vi "Dust_Control_Giraffe.vi"(7 "error in":errorcluster) -> (0 "error out":errorcluster)   [LabVIEW 2013]
doc: "This VI specifies the properties of the pulse used for running the dust source. When program is stopped, the voltage is incrementally reduced to zero to avoid quick drops."
uses:
  Private/Controls/dust_soruce_control.ctl
  Private/Controls/XYVoltageFGV.ctl
  <vilib>/Utility/miscctls.llb/LVPointTypeDef.ctl
  <vilib>/Utility/error.llb/DialogType.ctl
  <vilib>/Utility/miscctls.llb/LVMinMaxIncTypeDef.ctl
  <vilib>/Utility/miscctls.llb/LVRangeTypeDef.ctl
  <vilib>/DAQmx/read.llb/DAQmx Read (Analog 1D Wfm NChan NSamp).vi
  <vilib>/Analysis/baseanly.llb/Mean (DBL).vi
  <vilib>/DAQmx/write.llb/DAQmx Write (Analog 1D Wfm NChan NSamp).vi
  <vilib>/DAQmx/read.llb/DAQmx Read (Counter U32 1Chan 1Samp).vi
  <vilib>/DAQmx/create/channels.llb/DAQmx Create Channel (AI-Voltage-Basic).vi
  <vilib>/DAQmx/configure/timing.llb/DAQmx Timing (Sample Clock).vi
  <vilib>/DAQmx/create/channels.llb/DAQmx Create Channel (AO-Voltage-Basic).vi
  <vilib>/DAQmx/create/channels.llb/DAQmx Create Channel (CI-Count Edges).vi
  <vilib>/measure/mascope.llb/Amplitude and Levels 1 chan.vi
  <vilib>/DAQmx/miscellaneous.llb/DAQmx Fill In Error Info.vi
  Private/UI Elements/throttle.vi
  <userlib>/_OpenG.lib/comparison/comparison.llb/Boolean Changed__ogtk.vi
  Private/UI Elements/throttle from query.vi
  <userlib>/_OpenG.lib/comparison/comparison.llb/DBL Changed__ogtk.vi
  <vilib>/addons/database/Connection.llb/Conn Execute.vi
  <vilib>/addons/database/Recordset.llb/Rec Fetch Recordset Data (R).vi
  <vilib>/addons/database/Recordset.llb/Rec Destroy - Connection.vi
  Private/Sub-Polymorphic/post_dust_source.vi
  <vilib>/addons/database/_DB Variant To Data/Database Variant To Data.xnode
  <resource>/objmgr/daqmx.rc
  <vilib>/measure/NI_MAPro.lvlib
  <vilib>/Analysis/NI_AALBase.lvlib
  <vilib>/addons/database/NI_Database_API.lvlib
panel:
  out "Einzel and Steering":T1
  out "Y Vs":dbl[](array[numeric])
  out "X Vs":dbl[](array[numeric])
  out "Einzel Vs":dbl[](array[numeric])
  out "Old Einzel":dbl min=0.0 max=10.0 step=0.01 format="%.2g"
  out "Rate Data":dbl[][][](array[numeric])
  out "Freq. Before Throttle":dbl
  out "On/Off":bool
  out "Finished":bool=TRUE
  out "Output waveform":waveform(dbl)={"t0"=timestamp(0 s since 1904-01-01), "dt"=4e-06, "Y"=array[50000 elements]}
  out "Input waveform":waveform(dbl)={"t0"=timestamp(3437998856.0330505 s since 1904-01-01), "dt"=0.00019999999999999998, "Y"=array[1000 elements], "attributes"=variant("NI_ChannelName"=variant(string "Dev5/ai20"), "NI_UnitDescription"=variant(string "Volts"))}
  out "output cluster":T2={"Integer Timestamp"=0, "Einzel Voltage"=0.0, "Needle Voltage"=0.0, "Frequency"=1.0, "Width (ms) : 0.1 "=0.1, "Desired Amplitude (V)"=0.0, "X Voltage"=0.0, "Y Voltage"=0.0, "Settings ID"="", "ID#"=0} {"Needle Voltage" min=0.0 max=10.0 step=0.01 format="%.2g"; "Y Voltage" min=0.0 max=9.0 step=0.01 format="%.2g"; "X Voltage" min=0.0 max=9.0 step=0.01 format="%.2g"; "Einzel Voltage" min=0.0 max=10.0 step=0.01 format="%.2g"; "Desired Amplitude (V)" min=0.0 max=10.0 step=0.01 format="%5.2f"; "Width (ms) : 0.1" min=0.05 max=5.0 step=0.01 format="%6.2f"; "Frequency" min=1.0 max=100.0 step=0.01 format="%.1f"}
  in  "Tab Control":T3(tab)
  in  "Things to Scan":cluster{"Einzel":bool, "X":bool, "Y":bool}={"Einzel"=TRUE, "X"=TRUE, "Y"=TRUE}
  in  "Ein. Range":dbl[](array[numeric])=[0.0, 10.0] min=0.0 max=10.0 step=0.05 format="%#.2g"
  out "Steps to go":i32
  out "Num Steps":i16
  in  "# of Steps":i16[](array[numeric])=[5, 5, 5] min=0 max=10 step=1
  in  "Y Range":dbl[](array[numeric])=[-2.5, 2.5] min=-2.5 max=2.5 step=0.05 format="%#.2g"
  in  "X Range":dbl[](array[numeric])=[-2.5, 2.5] min=-2.5 max=2.5 step=0.05 format="%#.2g"
  in  "Calibrate XY":bool
  out "Actual output width (ms)":dbl caption="Output Width (ms)" format="%.2f"
  out "Actual output Frequency":dbl caption="Output  Freq.(hz)" format="%.2f"
  in  "Width (ms) : 0.1":dbl=0.1 caption="Width (ms)" min=0.0 max=5.0 step=0.01 format="%6.2f"
  out "Actual Amplitude (V) 2":dbl=0.0012999050305587314 caption="Tube Drive" format="%.2f"
  in  "Desired Amplitude (V)":dbl caption="Amplitude (V)" min=0.0 max=10.0 step=0.01 format="%5.2f"
  out "Actual output Amplitude (V)":dbl caption="Output Amp. (V)" format="%.2f"
  in  "Frequency":dbl=1.0 caption="Freq. (Hz)" min=0.0 max=30.0 step=0.01 format="%.1f"
  in  "Abort Change":bool
  out "Actual Needle (kV)":dbl=-1.1093266413053247 caption="Actual Einzel (V)" format="%.2f"
  out "Actual Needle Output (V)":dbl caption="Actual Einzel (V)" format="%.2f"
  in  "Needle Voltage":dbl min=0.0 max=10.0 step=0.01 format="%.2g"
  out "Actual Steerer Y (kV)":dbl=-0.02640654867851852 caption="Actual Einzel (V)" format="%.2f"
  out "Actual Y Output (V)":dbl=4.5 caption="Actual Einzel (V)" format="%.2f"
  in  "Y Voltage":dbl min=-2.5 max=2.5 step=0.01 format="%.2g"
  out "Actual Steerer X (kV)":dbl=-0.07767573560151271 caption="Actual Einzel (V)" format="%.2f"
  out "Actual X Output (V)":dbl=4.5 caption="Actual Einzel (V)" format="%.2f"
  in  "X Voltage":dbl min=-2.5 max=2.5 step=0.01 format="%.2g"
  out "Actual Einzel (kV)":dbl=-1.1709848579608468 caption="Actual Einzel (V)" format="%.2f"
  out "Actual Einzel Output (V)":dbl caption="Actual Einzel (V)" format="%.2f"
  in  "Einzel Voltage":dbl min=0.0 max=10.0 step=0.01 format="%.2g"
  in  "Save Settings?":bool
  in  "Settings ID":string
  out "CONTROLS":waveform(dbl)[](graph)=[{"t0"=timestamp(0 s since 1904-01-01), "dt"=4e-06, "Y"=array[50000 elements]}, {"t0"=timestamp(3437998856.0330505 s since 1904-01-01), "dt"=0.00019999999999999998, "Y"=array[1000 elements], "attributes"=variant("NI_ChannelName"=variant(string "Dev5/ai20"), "NI_UnitDescription"=variant(string "Volts"))}]
  in  "Retrieve Settings":bool
  out "Det2/Det1":dbl
  out "Det3/Det1":dbl
  out "PSU/Det3":dbl
  out "PSU/Det2":dbl
  out "First detector since\nlast source change:":i64
  out "Third detector since\nlast source change:":i64
  out "Source Efficiency":dbl
  out "Det1 Rate":dbl
  out "PSU Rate":dbl
  out "Det3 Rate":dbl
  in  "Cycles to Avg.":i32=10
  out "Hours Run":dbl
  in  "Y Slice":dbl(slide) min=-2.5 max=2.5 step=1.25 scale=-2.5..2.5
  in  "X Slice":dbl(slide) min=-2.5 max=2.5 step=1.25 scale=-2.5..2.5
  in  "Einzel Slice":dbl(slide) min=0.0 max=10.0 step=2.5 scale=0.0..10.0
  out "Y Slice Data":dbl[][](graph)
  out "X Slice Data":dbl[][](graph)
  out "Einzel Slice Data":dbl[][](graph)
  in  "Maximums":cluster{"Width":dbl, "Freq.":dbl}
  out "Testing":bool
  in  "Physical Channels":tag="Dev4/ao19, Dev4/ao9, Dev4/ao11:12, Dev4/ao16" caption="Physical Output Channels"
  in  "Physical Input Channels":tag="Dev5/ai19:23"
  out "Execution Number:":i32=341
  in  "Cal Test?":bool
  in  "Counters On/Off":bool=TRUE
  in  "Reset Counters":bool
  in  "Det1":tag="Dev5/ctr0"
  in  "Det2":tag="Dev5/ctr1"
  in  "Det3":tag="Dev4/ctr0"
  in  "PSU":tag="Dev4/ctr1"
  out "PSU":u32
  out "Det3":u32
  out "Det2":u32
  out "Det1":u32
  out "error?":bool
  out "Actual Sample Clock Rate":dbl=250000.0 format="%.2f"
  in  "stop":bool
  # "Dust Source Control"
  # "Hold Down to\nStop Changes"
  # "E"
  # "x"
  # "y"
  # "Tube Drive (Ao0, Ai4)"
  # "Needle Control (Ao4, Ai0)"
  # "Steerer Y Control (Ao3, Ai3)"
  # "Steerer X Control (Ao2, Ai2)"
  # "Einzel Lens (Ao1, Ai1)"
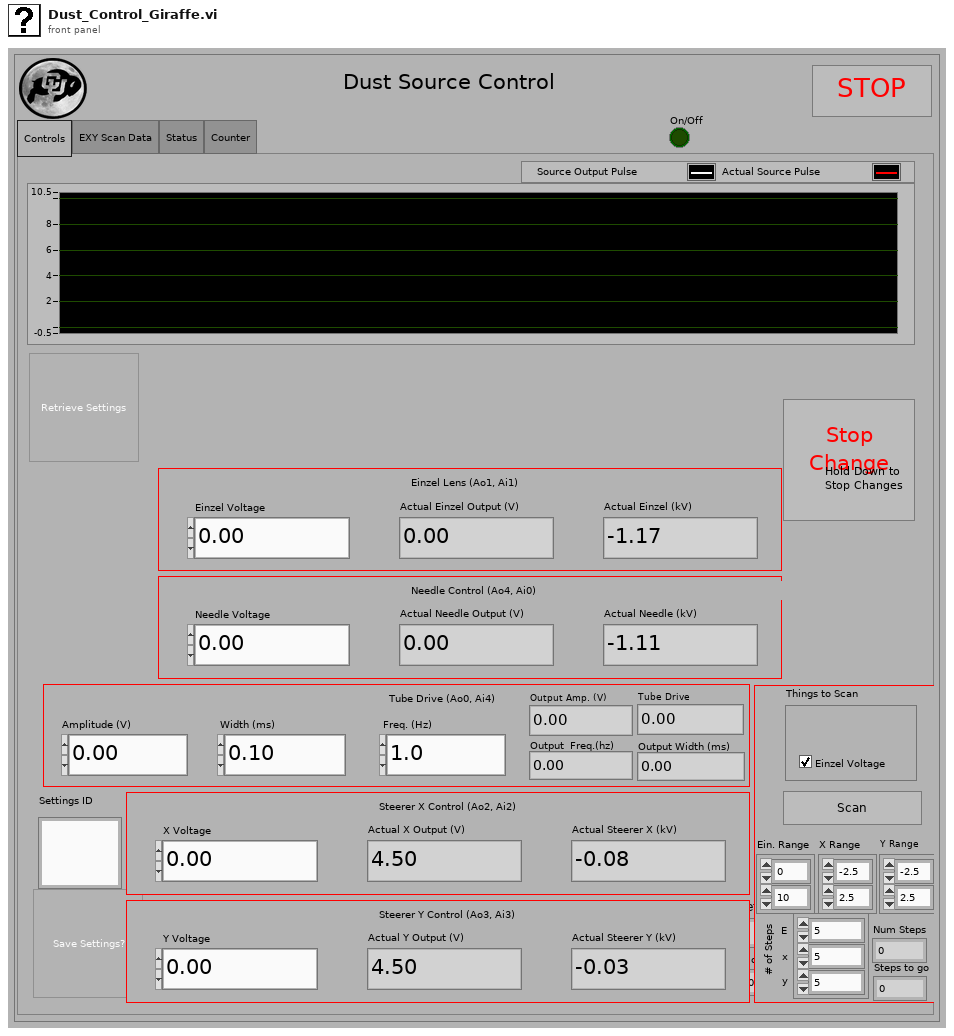
[diagram p1: front panel]
types:
  T1 = cluster{"Einzel Voltage":dbl, "X Voltage":dbl, "Y Voltage":dbl}
  T2 = typedef "dust_soruce_control.ctl" = cluster{"Integer Timestamp":u64, "Einzel Voltage":dbl, "Needle Voltage":dbl, "Frequency":dbl, "Width (ms) : 0.1 ":dbl, "Desired Amplitude (V)":dbl, "X Voltage":dbl, "Y Voltage":dbl, "Settings ID":string, "ID#":i32}
  T3 = enum32{"Controls", "EXY Scan Data", "Status", "Counter"}
  T4 = typedef "LVPointTypeDef.ctl" = cluster{"Horizontal":i16, "Vertical":i16}
  T5 = typedef "XYVoltageFGV.ctl" = u16
  T6 = enum8{"Enabled", "Disabled", "Disabled and Grayed Out"}
  T7 = typedef "DialogType.ctl" = u16
  T8 = typedef "NI_Database_API.lvlib/Conn ObjectReference.ctl" = refnum<k1>
  T9 = typedef "NI_Database_API.lvlib/Rec ObjectReference.ctl" = refnum<k1>
  T10 = typedef "LVRangeTypeDef.ctl" = cluster{"Minimum":dbl, "Maximum":dbl, "Increment":dbl, "Minor Increment":dbl, "Start":dbl}
  T11 = typedef "LVMinMaxIncTypeDef.ctl" = cluster{"Minimum":dbl, "Maximum":dbl, "Increment":dbl}
  T12 = cluster{"data":u32, "data":u32, "data":u32, "data":u32}
  T13 = cluster{"Minimum":dbl, dbl, "Increment":dbl, "Minor Increment":dbl, "Start":dbl}
  T14 = cluster{"Integer Time":i64, "Integer Time":i64, "data":i32}
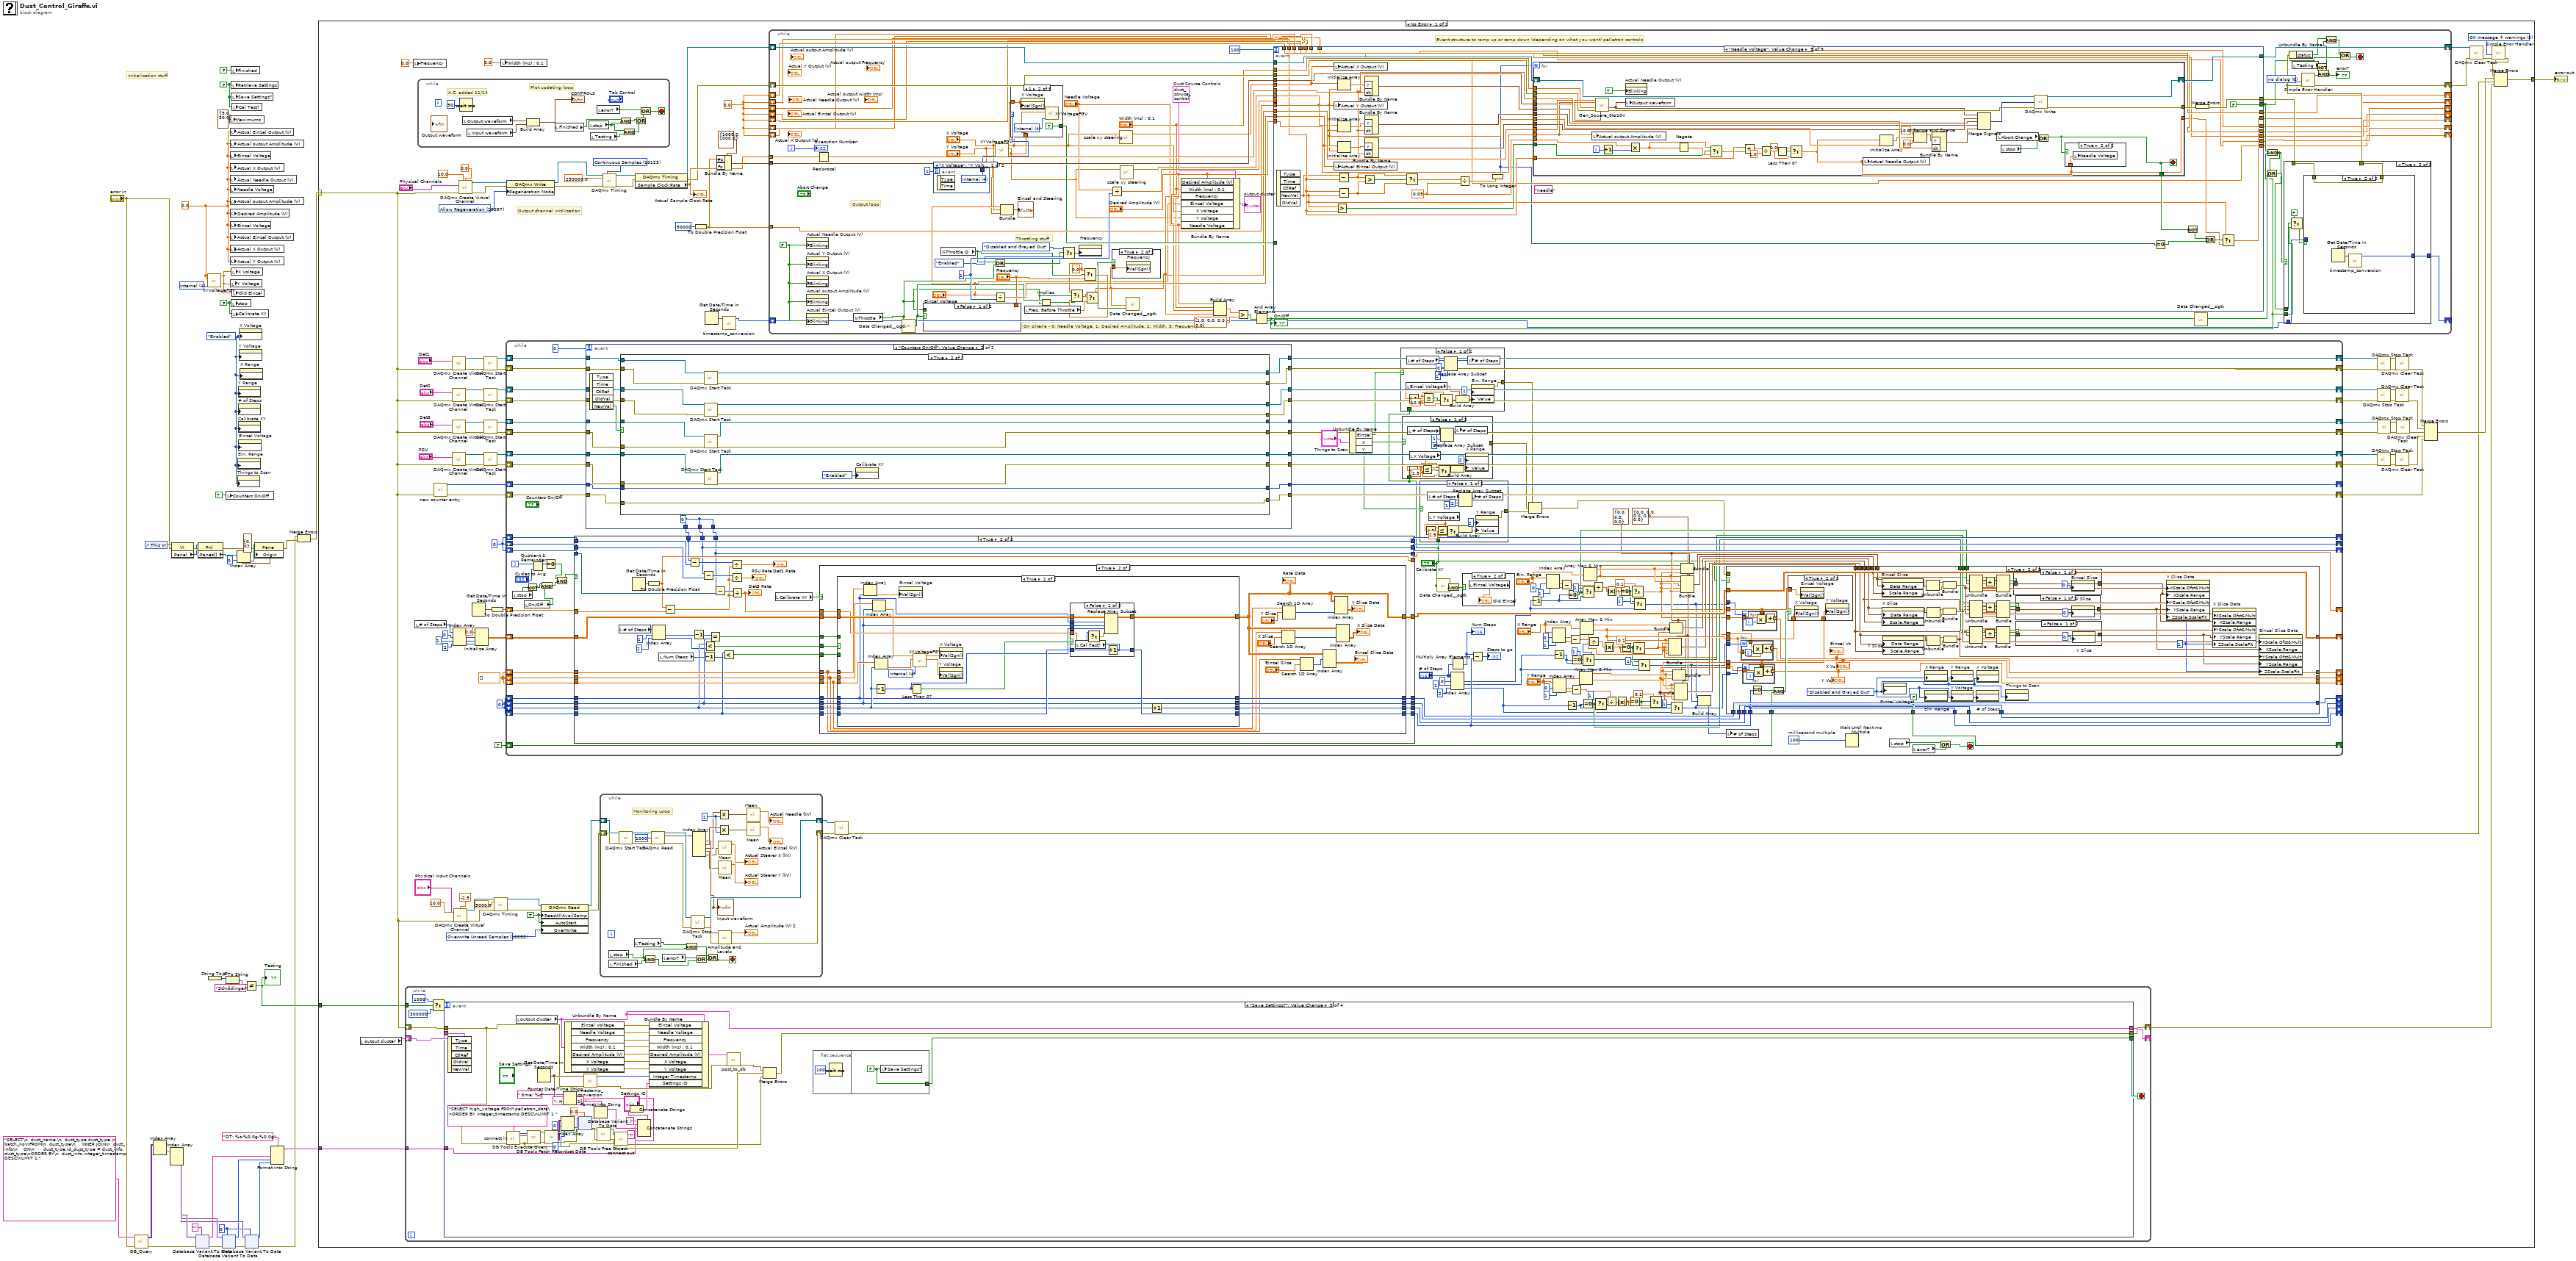
[diagram p0: block diagram]
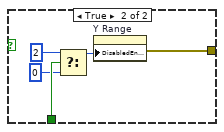
[diagram p2: hidden frame]
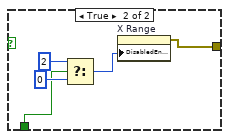
[diagram p3: hidden frame]
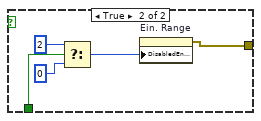
[diagram p4: hidden frame]
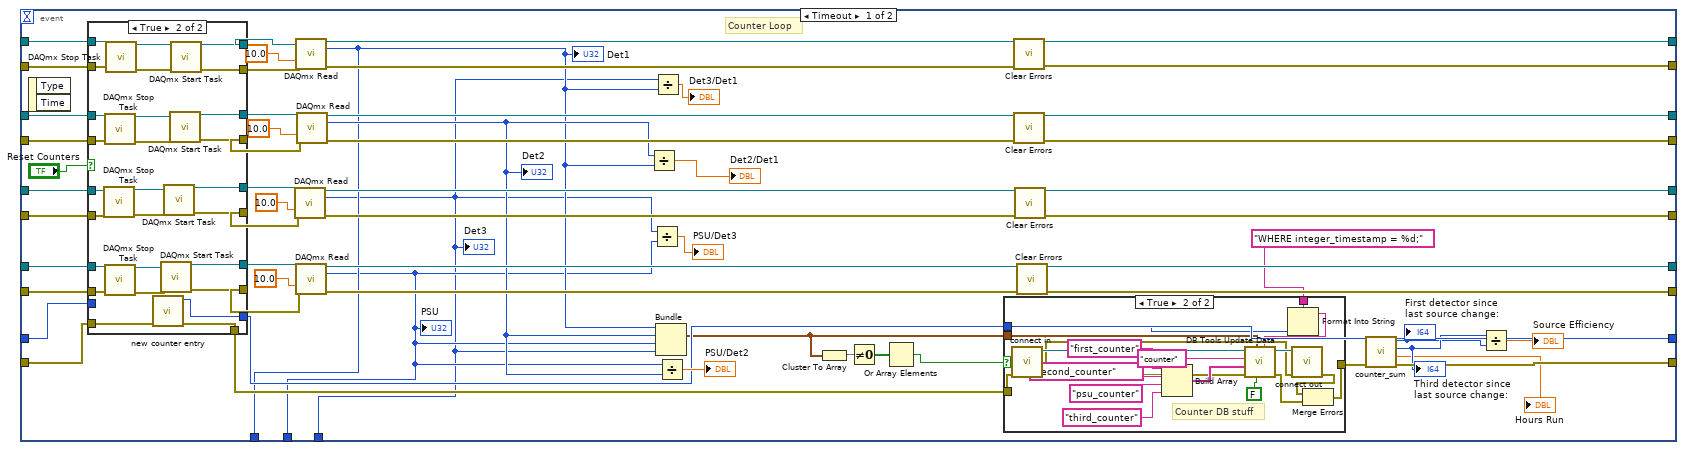
[diagram p6: hidden frame]
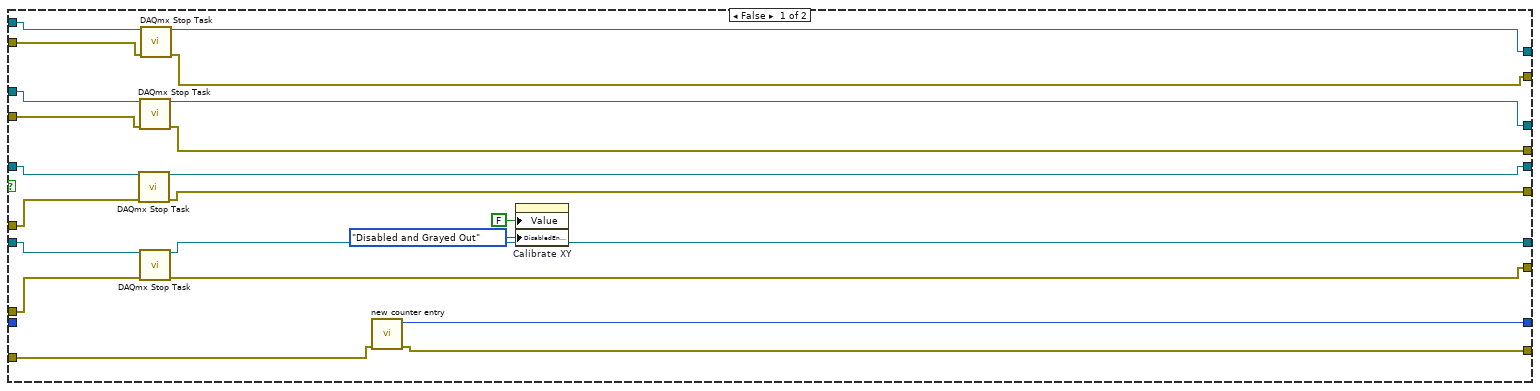
[diagram p9: hidden frame]
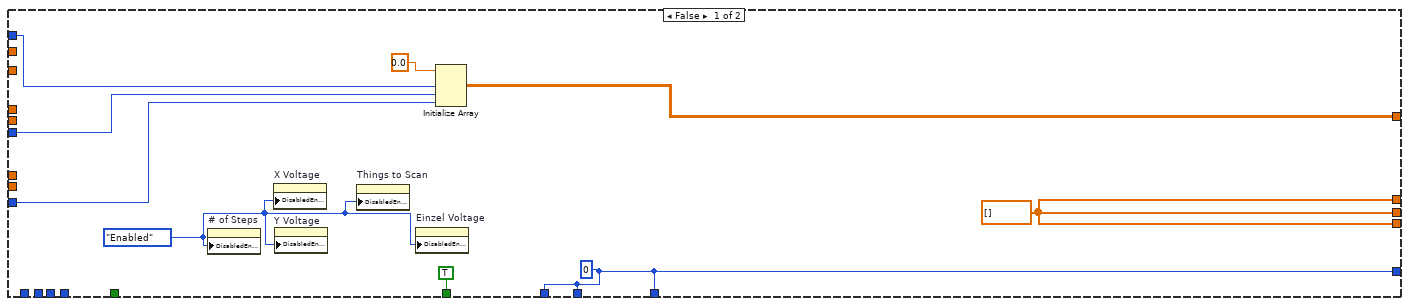
[diagram p10: hidden frame]
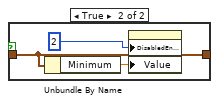
[diagram p11: hidden frame]
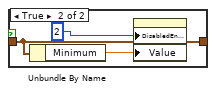
[diagram p12: hidden frame]
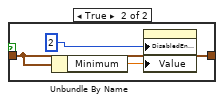
[diagram p13: hidden frame]
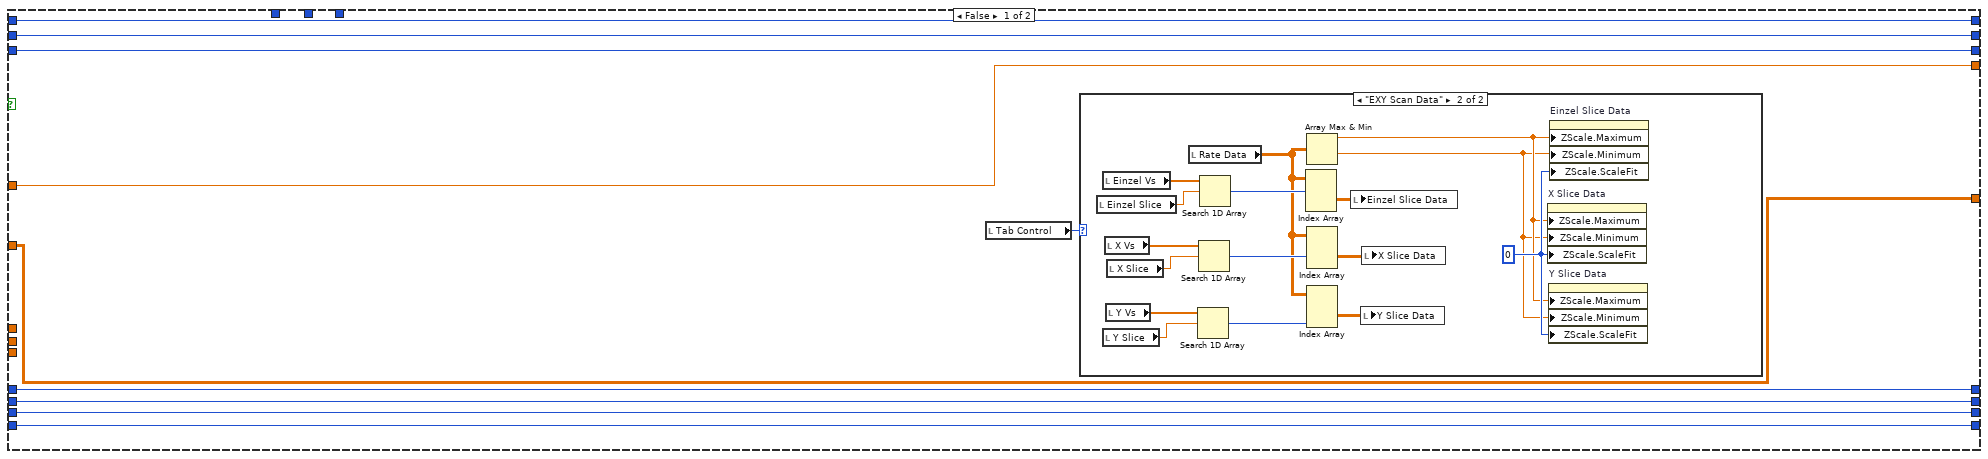
[diagram p15: hidden frame]
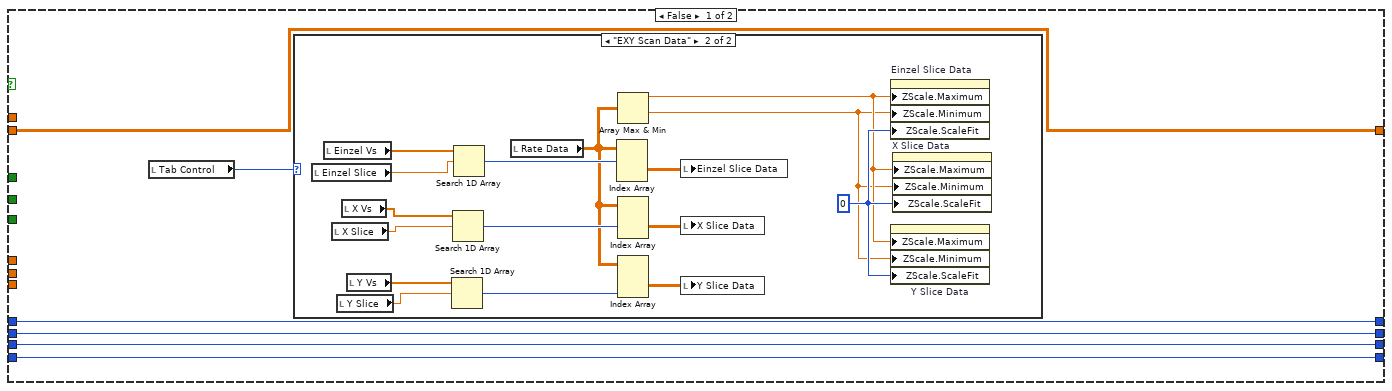
[diagram p17: hidden frame]
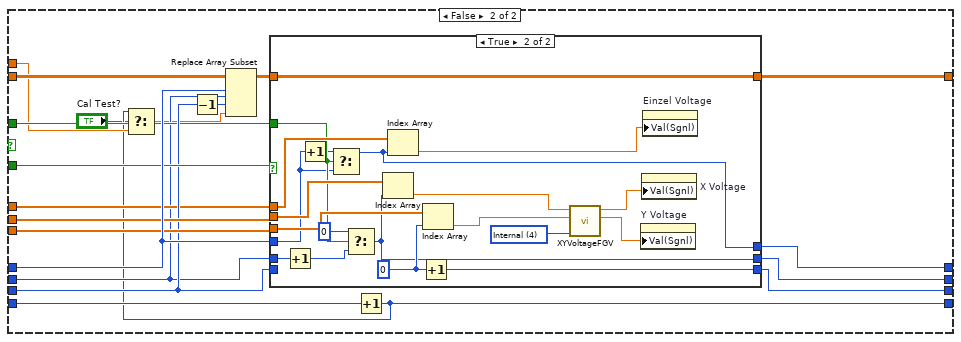
[diagram p20: hidden frame]
diagram:
  w29 = 0
  w38 = T5 4 items=["Get", "Set X", "Set Y", "Set XY", "Internal"] ("Ring")
  w16 = T6."Enabled" ("Disabled")
  w17 = FALSE ("Retrieve Settings")
  w40 = 0.0 ("Actual Output (V)")
  w39 = FALSE ("Shutdown")
  # "Initialization stuff"
  n1 = call "DB_Query.vi"("error in (no error)"="error in", "Parameterized Query"="SELECT\n  dust_name,\n  dust_type.dust_type,\n  batch_no\nFROM\n  dust_type\n    INNER JOIN\n  dust_info\n    ON\n      dust_type.id_dust_type = dust_info.dust_type\nORDER BY\n  dust_info.integer_timestamp DESC\nLIMIT 1;" ("SQL query")) -> ("error out"=w3:errorcluster, "Results"=w2:variant[][])  [unwired: 7 in, 1 out]
  n2 = control-ref of="This VI"() -> (w15:refnum<vi>)
  n3 = Index Array(array=w2) -> (element=w36:variant[])  [unwired: 2 in]
  n4 = Index Array(array=w36) -> (element #1=w35:variant, element #2=w32:variant, element #3=w31:variant)  [unwired: 3 in]
  n5 = property class="VI"(reference=w15, error in="error in") -> (error out=w14:errorcluster, "Panel"=w13:refnum<vi>)  [unwired: 1 out]
  n6 = xnode "Database Variant To Data"("database variant"=w35, "error in (no error)"=w3, "type"="") -> ("data"=w27:string, "error out"=w34:errorcluster)
  n7 = property class="Pnl"(reference=w13, error in=w14) -> (error out=w12:errorcluster, "Panes[]"=w11:refnum<vi>[])  [unwired: 1 out]
  n8 = call "XYVoltageFGV.vi"("X Voltage"=w40, "Y Voltage"=w40, "Ring"=w38) -> ("X Voltage 2"=w18:dbl)  [unwired: 5 in, 2 out]
  n9 = String To IP() -> (0:w23:u32)  [unwired: 1 in]
  n10 = xnode "Database Variant To Data"("database variant"=w32, "error in (no error)"=w34, "type"=w29) -> ("data"=w26:i32, "error out"=w33:errorcluster)
  n11 = local write "Counters On/Off"(TRUE ("Counters On/Off")) -> ()
  n12 = IP To String(2:w23) -> (0:w22:string)  [unwired: 1 in]
  n13 = local write "Maximums"(cluster{"Width":dbl, "Freq.":dbl} {"Width"=5.0, "Freq."=30.0} ("Maximums")) -> ()
  n14 = local write "Actual Einzel Output (V)"(w40) -> ()
  n15 = local write "Actual output Amplitude (V)"(w40) -> ()
  n16 = local write "Einzel Voltage"(w40) -> ()
  n17 = local write "Actual X Output (V)"(w40) -> ()
  n18 = local write "Actual Needle Output (V)"(w40) -> ()
  n19 = local write "Needle Voltage"(w40) -> ()
  n20 = local write "Actual output Amplitude (V)"(w40) -> ()
  n21 = local write "Desired Amplitude (V)"(w40) -> ()
  n22 = local write "Einzel Voltage"(w40) -> ()
  n23 = local write "Actual Einzel Output (V)"(w40) -> ()
  n24 = local write "Actual X Output (V)"(w40) -> ()
  n25 = local write "Actual Y Output (V)"(w40) -> ()
  n26 = local write "Y Voltage"(w18) -> ()
  n27 = local write "Finished"(FALSE ("Finished")) -> ()
  n28 = local write "Retrieve Settings"(w17) -> ()
  n29 = local write "Save Settings?"(w17) -> ()
  n30 = local write "X Voltage"(w18) -> ()
  n31 = local write "stop"(w39) -> ()
  n32 = local write "Cal Test?"(w17) -> ()
  n33 = local write "Old Einzel"(w18) -> ()
  n34 = local write "Calibrate XY"(w39) -> ()
  n35 = Index Array(array=w11, index=0) -> (element=w9:refnum<vi>)
  n36 = property on="Things to Scan" class="Clust (strict)"("DisabledEnum"=w16) -> ()  [unwired: 2 in, 2 out]
  n37 = property on="Ein. Range" class="Arr (strict)"("DisabledEnum"=w16) -> ()  [unwired: 2 in, 2 out]
  n38 = property on="Y Range" class="Arr (strict)"("DisabledEnum"=w16) -> ()  [unwired: 2 in, 2 out]
  n39 = property on="# of Steps" class="Arr (strict)"("DisabledEnum"=w16) -> ()  [unwired: 2 in, 2 out]
  n40 = property on="Calibrate XY" class="Bool (strict)"("DisabledEnum"=w16) -> ()  [unwired: 2 in, 2 out]
  n41 = property on="Einzel Voltage" class="DigNum (strict)"("DisabledEnum"=w16) -> ()  [unwired: 2 in, 2 out]
  n42 = property on="Y Voltage" class="DigNum (strict)"("DisabledEnum"=w16) -> ()  [unwired: 2 in, 2 out]
  n43 = property on="X Voltage" class="DigNum (strict)"("DisabledEnum"=w16) -> ()  [unwired: 2 in, 2 out]
  n44 = property on="X Range" class="Arr (strict)"("DisabledEnum"=w16) -> ()  [unwired: 2 in, 2 out]
  n45 = Not Equal?(x=w22, y="Schrödinger") -> (x != y?=w20:bool)
  "Testing" <- w20
  n46 = xnode "Database Variant To Data"("database variant"=w31, "error in (no error)"=w33, "type"=w29) -> ("data"=w25:i32, "error out"=w1:errorcluster)
  n47 = property class="Pane"(reference=w9, error in=w12, "Origin"=T4 {"Horizontal"=0, "Vertical"=0}) -> (error out=w7:errorcluster)  [unwired: 1 out]
  n48 = Format Into String(format string="DT: %s-%0.0g-%0.0g", w27, w26, w25) -> (resulting string=w24:string)  [unwired: 2 in, 1 out]
  n49 = Merge Errors(w1, w7) -> (w6:errorcluster)
  n50 = case shown="No Error" w6 {
    selector: w6 -> [w64 w2376]
    tunnel: [w43 w2376] -> w42
    tunnel: w24 -> [w50 _]
    tunnel: w20 -> [w49 _]
    frame No Error {
      w53 = 0.0 ("Width (ms) : 3.5")
      w48 = dbl[] []
      w45 = 0
      w74 = 10252 items=["Overwrite Unread Samples"=10252, "Do Not Overwrite Unread Samples"=10159] ("OverWrite")
      w75 = TRUE ("ReadAllAvailSamp")
      w44 = u32 0 ("data")
      w142 = 10097 items=["Allow Regeneration"=10097, "Do Not Allow Regeneration"=10158] ("RegenMode")
      w147 = T7 3 items=["no dialog", "OK message", "continue or stop message", "OK message + warnings", "continue/stop + warnings"] ("type of dialog (OK msg:1)")
      w151 = 10123 items=["Finite Samples"=10178, "Continuous Samples"=10123] ("sample mode")
      # "Output channel initilization"
      n51 = local read "output cluster"() -> (w127:T2)
      n52 = while {
        shift-right: [w907] -> w83
        shift-left: w64 -> [w906]
        shift-right: [w910] -> _
        shift-left: w127 -> [w909]
        tunnel: w50 -> [w904]
        tunnel: w49 -> [w902]
        stop <- w905 stop-if-true
        n53 = Select(t=1000, s=w902, f=300000) -> (s? t:f=w903:i32)
        n54 = event shown="[2] \"Save Settings?\": Value Change" {
          selector: _ -> [_ _ _ _]
          dyn-events: _ -> [_ _ _ _]
          timeout: w903 -> [_ _ _ _]
          tunnel: [w940 w1017 w1061 w1098] -> w910
          tunnel: w909 -> [w939 w1017 _ _]
          tunnel: [w912 w1018 w1028 w1100] -> w907
          tunnel: w906 -> [w913 w1018 w1030 w1099]
          tunnel: [w915 w1014 w1058 _] -> w905
          tunnel: w904 -> [w911 _ w1024 _]
          event Timeout {
            n55 = event-data() -> ()  [unwired: 1 in, 2 out]
            n56 = local read "output cluster"() -> (w940:T2)
            n57 = Unbundle By Name(w940) -> ("Einzel Voltage"=w937:dbl, "Needle Voltage"=w936:dbl, "Frequency"=w934:dbl, "Width (ms) : 0.1"=w932:dbl, "Desired Amplitude (V)"=w930:dbl, "X Voltage"=w929:dbl, "Y Voltage"=w927:dbl)
            n58 = Unbundle By Name(w939) -> ("Einzel Voltage"=w938:dbl, "Needle Voltage"=w935:dbl, "Frequency"=w933:dbl, "Width (ms) : 0.1"=w918:dbl, "Desired Amplitude (V)"=w931:dbl, "X Voltage"=w928:dbl, "Y Voltage"=w926:dbl)
            n59 = Equal?(x=w937, y=w938) -> (x = y?=w925:bool)
            n60 = Equal?(x=w936, y=w935) -> (x = y?=w924:bool)
            n61 = Equal?(x=w934, y=w933) -> (x = y?=w923:bool)
            n62 = Equal?(x=w932, y=w918) -> (x = y?=w922:bool)
            n63 = Equal?(x=w930, y=w931) -> (x = y?=w921:bool)
            n64 = Equal?(x=w929, y=w928) -> (x = y?=w920:bool)
            n65 = Equal?(x=w927, y=w926) -> (x = y?=w919:bool)
            n66 = Compound Arithmetic op=AND(w925, w924, w923, w922, w921, w920, w919) -> (w914:bool)
            n67 = case shown="False" w914 {
              tunnel: w913 -> [w942 w1013]
              tunnel: [w957 w1013] -> w912
              tunnel: w911 -> [w947 _]
              frame False {
                n68 = call "DB_Query.vi"("error in (no error)"=w942, "Parameterized Query"="SELECT\n  high_voltage\nFROM\n  pelletron_data\nORDER BY\n  integer_timestamp DESC\nLIMIT 1; " ("SQL query")) -> ("error out"=w943:errorcluster, "Results"=w944:variant[][])  [unwired: 7 in, 1 out]
                n69 = local read "output cluster"() -> (w959:T2)
                n70 = Get Date/Time In Seconds() -> (seconds since 1Jan1904=w974:timestamp)
                n71 = Format Date/Time String(time format string (%c)="Time: %c)" ("Settings ID"), seconds (now)=w974) -> (date/time string=w949:string)  [unwired: 1 in]
                n72 = Index Array(array=w944, index (row)=0, index (col)=0 ("disabled index (col)")) -> (element=w954:variant)
                n73 = Unbundle By Name(w959) -> ("Einzel Voltage"=w972:dbl, "Needle Voltage"=w971:dbl, "Frequency"=w965:dbl, "Width (ms) : 0.1"=w964:dbl, "Desired Amplitude (V)"=w970:dbl, "X Voltage"=w968:dbl, "Y Voltage"=w967:dbl)
                n74 = xnode "Database Variant To Data"("database variant"=w954, "error in (no error)"=w943, "type"=0.0 ("input 1")) -> ("data"=w952:dbl, "error out"=w941:errorcluster)
                n75 = call "timestamp_conversion.vi"("error in (no error)"=w941, "Time Stamp"=w974) -> ("error out"=w975:errorcluster, "Integer Time"=w976:i64)  [unwired: 7 in]
                n76 = Format Into String(format string="Automatic Update (%s; HV: %0.1f; ", w947, w952) -> (resulting string=w950:string)  [unwired: 2 in, 1 out]
                n77 = Concatenate Strings(w950, w949) -> (w948:string)
                n78 = Bundle By Name(cluster=w959, "Einzel Voltage"=w972, "Needle Voltage"=w971, "Frequency"=w965, "Width (ms) : 0.1"=w964, "Desired Amplitude (V)"=w970, "X Voltage"=w968, "Y Voltage"=w967, "Integer Timestamp"=w976, "Settings ID"=w948) -> (w960:T2)
                n79 = Build Array(w971, w970) -> (w969:dbl[])
                n80 = Less Or Equal?(x=w964, y=0.01) -> (x <= y?=w958:bool)
                n81 = Less?(x=w969, y=0.1) -> (x < y?=w962:bool[])
                n82 = Build Array (concatenate)(w962, w958) -> (w961:bool[])
                n83 = Or Array Elements(Boolean array=w961) -> (logical OR=w946:bool)
                n84 = case shown="False" w946 {
                  tunnel: w960 -> [w1009 _]
                  tunnel: [w1011 w1012] -> w957
                  tunnel: w975 -> [w1010 w1012]
                  frame False {
                    n85 = call-poly "post_to_db.vi"("error in (no error)"=w1010, "Dust control settings"=w1009) -> ("error out"=w1011:errorcluster)  [unwired: 9 in]
                  }
                  frame True {
                  }
                }
              }
              frame True {
              }
            }
            n86 = local read "error?"() -> (w916:bool)
            n87 = local read "stop"() -> (w917:bool)
            n88 = Or(x=w917, y=w916) -> (x .or. y?=w915:bool)
          }
          event "stop": Value Change {
            n89 = event-data() -> ()  [unwired: 1 in, 5 out]
            n90 = local read "stop"() -> (w1016:bool)
            n91 = local read "error?"() -> (w1015:bool)
            n92 = Or(x=w1016, y=w1015) -> (x .or. y?=w1014:bool)
          }
          event "Save Settings?": Value Change {
            n93 = event-data() -> ()  [unwired: 1 in, 5 out]
            n94 = call "connect in.vi"("error in (no error)"=w1030) -> ("error out"=w1043:errorcluster, "Database Connection"=w1046:T8)  [unwired: 6 in, 1 out]
            n95 = local read "output cluster"() -> (w1061:T2)
            n96 = call-poly <vilib>:"DB Tools Execute Query.vi"("error in (no error)"=w1043, "SQL query"="SELECT high_voltage FROM pelletron_data\nORDER BY integer_timestamp DESC\nLIMIT 1 ", "connection reference"=w1046) -> ("error out"=w1045:errorcluster, "recordset reference"=w1044:T9)  [unwired: 5 in]
            n97 = Get Date/Time In Seconds() -> (seconds since 1Jan1904=w1056:timestamp)
            n98 = call-poly <vilib>:"DB Tools Fetch Recordset Data.vi"("error in (no error)"=w1045, "recordset reference"=w1044) -> ("error out"=w1034:errorcluster, "recordset data"=w1038:variant[][], "recordset reference out"=w1042:T9)  [unwired: 3 in]
            n99 = Index Array(array=w1038, index (row)=0, index (col)=0 ("disabled index (col)")) -> (element=w1035:variant)
            n100 = Format Date/Time String(time format string (%c)=" time: %c" ("Settings ID"), seconds (now)=w1056) -> (date/time string=w1022:string)  [unwired: 1 in]
            n101 = Unbundle By Name(w1061) -> ("Einzel Voltage"=w1055:dbl, "Needle Voltage"=w1054:dbl, "Frequency"=w1053:dbl, "Width (ms) : 0.1"=w1052:dbl, "Desired Amplitude (V)"=w1051:dbl, "X Voltage"=w1050:dbl, "Y Voltage"=w1049:dbl)
            n102 = xnode "Database Variant To Data"("database variant"=w1035, "error in (no error)"=w1034, "type"=0.0 ("input 1")) -> ("data"=w1031:dbl, "error out"=w1033:errorcluster)
            n103 = call "timestamp_conversion.vi"("error in (no error)"=w1030, "Time Stamp"=w1056) -> ("error out"=w1059:errorcluster, "Integer Time"=w1060:i64)  [unwired: 7 in]
            n104 = Format Into String(format string="; HV: %0.1f; ", w1031) -> (resulting string=w1023:string)  [unwired: 2 in, 1 out]
            n105 = call-poly <vilib>:"DB Tools Free Object.vi"("error in (no error)"=w1033, "recordset reference"=w1042) -> ("error out"=w1027:errorcluster, "connection reference"=w1041:T8)  [unwired: 8 in]
            n106 = call "connect out.vi"("error in (no error)"=w1043, "connection reference"=w1041) -> ("error out"=w1026:errorcluster)  [unwired: 9 in]
            n107 = Concatenate Strings(" (" ("string"), w1024, w1023, w1022, ")" ("string")) -> (w1020:string)
            n108 = Concatenate Strings("Settings ID", w1020) -> (w1047:string)
            n109 = Bundle By Name(cluster=w1061, "Einzel Voltage"=w1055, "Needle Voltage"=w1054, "Frequency"=w1053, "Width (ms) : 0.1"=w1052, "Desired Amplitude (V)"=w1051, "X Voltage"=w1050, "Y Voltage"=w1049, "Integer Timestamp"=w1060, "Settings ID"=w1047) -> (w1019:T2)
            n110 = call-poly "post_to_db.vi"("error in (no error)"=w1059, "Dust control settings"=w1019) -> ("error out"=w1029:errorcluster)  [unwired: 9 in]
            n111 = Merge Errors(w1029, w1027, w1026) -> (w1028:errorcluster)
            n112 = flat-sequence {
              tunnel: [w1095] -> w1058
              frame #0 {
                n113 = Wait (ms)(milliseconds to wait=u32 100) -> ()  [unwired: 1 out]
              }
              frame #1 {
                w1095 = FALSE
                n114 = local write "Save Settings?"(w1095) -> ()
              }
            }
          }
          event "Retrieve Settings": Value Change {
            n115 = event-data() -> ()  [unwired: 1 in, 5 out]
            n116 = local write "Retrieve Settings"(FALSE) -> ()
            n117 = call "Query_source_settings_menu.vi"("error in (no error)"=w1099) -> ("error out"=w1097:errorcluster, "Cancelled?"=w1096:bool, "Output cluster"=w1098:T2)  [unwired: 8 in]
            n118 = Unbundle By Name(w1098) -> ("Einzel Voltage"=w1108:dbl, "Needle Voltage"=w1107:dbl, "Frequency"=w1106:dbl, "Width (ms) : 0.1"=w1105:dbl, "Desired Amplitude (V)"=w1104:dbl, "X Voltage"=w1103:dbl, "Y Voltage"=w1102:dbl)
            n119 = case shown="False" w1096 {
              tunnel: w1108 -> [w1121 _]
              tunnel: w1097 -> [w1145 w1253]
              tunnel: w1107 -> [w1118 _]
              tunnel: w1106 -> [w1112 _]
              tunnel: w1105 -> [w1115 _]
              tunnel: w1104 -> [w1111 _]
              tunnel: w1103 -> [w1144 _]
              tunnel: w1102 -> [w1128 _]
              tunnel: [w1122 w1253] -> w1100
              frame False {
                n120 = flat-sequence {
                  tunnel: w1145 -> [w1147]
                  tunnel: [w1146] -> w1143
                  tunnel: w1144 -> [w1148]
                  tunnel: [w1148] -> w1142
                  tunnel: w1143 -> [w1150]
                  tunnel: [w1150] -> w1141
                  tunnel: w1142 -> [w1149]
                  tunnel: [w1149] -> w1140
                  tunnel: w1141 -> [w1153]
                  tunnel: [w1152] -> w1139
                  tunnel: w1140 -> [w1154]
                  tunnel: w1139 -> [w1168]
                  tunnel: [w1169] -> w1127
                  tunnel: w1128 -> [w1167]
                  tunnel: [w1167] -> w1123
                  tunnel: w1127 -> [w1172]
                  tunnel: [w1172] -> w1126
                  tunnel: [w1170] -> w1124
                  tunnel: w1123 -> [w1170]
                  tunnel: w1126 -> [w1175]
                  tunnel: [w1174] -> w1125
                  tunnel: w1124 -> [w1173]
                  tunnel: w1125 -> [w1189]
                  tunnel: [w1190] -> w1138
                  tunnel: w1121 -> [w1188]
                  tunnel: [w1188] -> w1120
                  tunnel: w1138 -> [w1192]
                  tunnel: [w1192] -> w1137
                  tunnel: w1120 -> [w1191]
                  tunnel: [w1191] -> w1119
                  tunnel: w1137 -> [w1195]
                  tunnel: [w1196] -> w1136
                  tunnel: w1119 -> [w1194]
                  tunnel: w1136 -> [w1206]
                  tunnel: [w1207] -> w1135
                  tunnel: w1118 -> [w1205]
                  tunnel: [w1205] -> w1116
                  tunnel: [w1209] -> w1134
                  tunnel: w1135 -> [w1209]
                  tunnel: [w1208] -> w1117
                  tunnel: w1116 -> [w1208]
                  tunnel: w1134 -> [w1212]
                  tunnel: [w1213] -> w1133
                  tunnel: w1117 -> [w1211]
                  tunnel: w1133 -> [w1227]
                  tunnel: [w1226] -> w1132
                  tunnel: w1111 -> [w1225]
                  tunnel: [w1225] -> w1109
                  tunnel: w1132 -> [w1230]
                  tunnel: [w1231] -> w1131
                  tunnel: w1115 -> [w1229]
                  tunnel: [w1228] -> w1110
                  tunnel: w1109 -> [w1228]
                  tunnel: w1131 -> [w1234]
                  tunnel: [w1233] -> w1130
                  tunnel: [w1235] -> w1113
                  tunnel: w1112 -> [w1232]
                  tunnel: w1110 -> [w1235]
                  tunnel: w1130 -> [w1237]
                  tunnel: [w1237] -> w1129
                  tunnel: [w1236] -> w1114
                  tunnel: w1113 -> [w1236]
                  tunnel: w1129 -> [w1241]
                  tunnel: [w1240] -> w1122
                  tunnel: w1114 -> [w1239]
                  frame #0 {
                    n121 = property on="X Voltage" class="DigNum (strict)"(error in=w1147, "Val(Sgnl)"=w1148) -> (error out=w1146:errorcluster)  [unwired: 1 in, 1 out]
                  }
                  frame #1 {
                    n122 = Wait (ms)(milliseconds to wait=u32 100) -> ()  [unwired: 1 out]
                  }
                  frame #2 {
                    n123 = while {
                      tunnel: w1154 -> [w1162]
                      shift-right: [w1166] -> w1152
                      shift-left: w1153 -> [w1166]
                      stop <- w1160 stop-if-true
                      n124 = local read "Actual X Output (V)"() -> (w1155:dbl)
                      n125 = local read "stop"() -> (w1157:bool)
                      n126 = local read "Abort Change"() -> (w1158:bool)
                      n127 = call "scale xy steering.vi"("0 to 9 V input"=w1155) -> ("-2.5 to 2.5 V output"=w1156:dbl)  [unwired: 1 in, 1 out]
                      n128 = Subtract(x=w1162, y=w1156) -> (x-y=w1165:dbl)
                      n129 = Absolute Value(x=w1165) -> (abs(x)=w1164:dbl)
                      n130 = Or(x=w1157, y=w1158) -> (x .or. y?=w1159:bool)
                      n131 = Less?(x=w1164, y=0.1) -> (x < y?=w1161:bool)
                      n132 = Or(x=w1161, y=w1159) -> (x .or. y?=w1160:bool)
                    }
                  }
                  frame #3 {
                    n133 = property on="Y Voltage" class="DigNum (strict)"(error in=w1168, "Val(Sgnl)"=w1167) -> (error out=w1169:errorcluster)  [unwired: 1 in, 1 out]
                  }
                  frame #4 {
                    n134 = Wait (ms)(milliseconds to wait=u32 100) -> ()  [unwired: 1 out]
                  }
                  frame #5 {
                    n135 = while {
                      shift-right: [w1187] -> w1174
                      shift-left: w1175 -> [w1187]
                      tunnel: w1173 -> [w1178]
                      stop <- w1181 stop-if-true
                      n136 = local read "Actual Y Output (V)"() -> (w1177:dbl)
                      n137 = local read "Abort Change"() -> (w1180:bool)
                      n138 = local read "stop"() -> (w1179:bool)
                      n139 = call "scale xy steering.vi"("0 to 9 V input"=w1177) -> ("-2.5 to 2.5 V output"=w1176:dbl)  [unwired: 1 in, 1 out]
                      n140 = Subtract(x=w1178, y=w1176) -> (x-y=w1186:dbl)
                      n141 = Absolute Value(x=w1186) -> (abs(x)=w1185:dbl)
                      n142 = Or(x=w1180, y=w1179) -> (x .or. y?=w1182:bool)
                      n143 = Less?(x=w1185, y=0.1) -> (x < y?=w1184:bool)
                      n144 = Or(x=w1184, y=w1182) -> (x .or. y?=w1181:bool)
                    }
                  }
                  frame #6 {
                    n145 = property on="Einzel Voltage" class="DigNum (strict)"(error in=w1189, "Val(Sgnl)"=w1188) -> (error out=w1190:errorcluster)  [unwired: 1 in, 1 out]
                  }
                  frame #7 {
                    n146 = Wait (ms)(milliseconds to wait=u32 100) -> ()  [unwired: 1 out]
                  }
                  frame #8 {
                    n147 = while {
                      shift-right: [w1204] -> w1196
                      shift-left: w1195 -> [w1204]
                      tunnel: w1194 -> [w1197]
                      stop <- w1201 stop-if-true
                      n148 = local read "Actual Einzel Output (V)"() -> (w1202:dbl)
                      n149 = local read "Abort Change"() -> (w1200:bool)
                      n150 = local read "stop"() -> (w1198:bool)
                      n151 = Or(x=w1200, y=w1198) -> (x .or. y?=w1199:bool)
                      n152 = Equal?(x=w1202, y=w1197) -> (x = y?=w1203:bool)
                      n153 = Or(x=w1203, y=w1199) -> (x .or. y?=w1201:bool)
                    }
                  }
                  frame #9 {
                    n154 = property on="Needle Voltage" class="DigNum (strict)"(error in=w1206, "Val(Sgnl)"=w1205) -> (error out=w1207:errorcluster)  [unwired: 1 in, 1 out]
                  }
                  frame #10 {
                    n155 = Wait (ms)(milliseconds to wait=u32 100) -> ()  [unwired: 1 out]
                  }
                  frame #11 {
                    n156 = while {
                      shift-right: [w1224] -> w1213
                      shift-left: w1212 -> [w1224]
                      tunnel: w1211 -> [w1214]
                      stop <- w1218 stop-if-true
                      n157 = local read "Actual Needle Output (V)"() -> (w1220:dbl)
                      n158 = local read "stop"() -> (w1215:bool)
                      n159 = local read "Abort Change"() -> (w1217:bool)
                      n160 = Subtract(x=w1220, y=w1214) -> (x-y=w1223:dbl)
                      n161 = Absolute Value(x=w1223) -> (abs(x)=w1222:dbl)
                      n162 = Or(x=w1215, y=w1217) -> (x .or. y?=w1216:bool)
                      n163 = Less?(x=w1222, y=0.1) -> (x < y?=w1219:bool)
                      n164 = Or(x=w1216, y=w1219) -> (x .or. y?=w1218:bool)
                    }
                  }
                  frame #12 {
                    n165 = property on="Desired Amplitude (V)" class="DigNum (strict)"(error in=w1227, "Val(Sgnl)"=w1225) -> (error out=w1226:errorcluster)  [unwired: 1 in, 1 out]
                  }
                  frame #13 {
                    n166 = property on="Width (ms) : 0.1" class="DigNum (strict)"(error in=w1230, "Val(Sgnl)"=w1229) -> (error out=w1231:errorcluster)  [unwired: 1 in, 1 out]
                  }
                  frame #14 {
                    n167 = property on="Frequency" class="DigNum (strict)"(error in=w1234, "Val(Sgnl)"=w1232) -> (error out=w1233:errorcluster)  [unwired: 1 in, 1 out]
                  }
                  frame #15 {
                    n168 = Wait (ms)(milliseconds to wait=u32 100) -> ()  [unwired: 1 out]
                  }
                  frame #16 {
                    n169 = while {
                      shift-right: [w1251] -> w1240
                      shift-left: w1241 -> [w1251]
                      tunnel: w1239 -> [w1242]
                      stop <- w1246 stop-if-true
                      n170 = local read "Actual output Amplitude (V)"() -> (w1252:dbl)
                      n171 = local read "stop"() -> (w1243:bool)
                      n172 = local read "Abort Change"() -> (w1244:bool)
                      n173 = Subtract(x=w1252, y=w1242) -> (x-y=w1249:dbl)
                      n174 = Absolute Value(x=w1249) -> (abs(x)=w1248:dbl)
                      n175 = Or(x=w1244, y=w1243) -> (x .or. y?=w1245:bool)
                      n176 = Less?(x=w1248, y=0.1) -> (x < y?=w1250:bool)
                      n177 = Or(x=w1250, y=w1245) -> (x .or. y?=w1246:bool)
                    }
                  }
                }
              }
              frame True {
              }
            }
          }
        }
      }
      n178 = local write "Frequency"(0.0 ("Frequency")) -> ()
      n179 = local read "# of Steps"() -> (w59:i16[])
      n180 = while {
        stop <- w867 stop-if-true
        # "Plot updating loop"
        # "A.C. added 11/14"
        n181 = Wait (ms)(milliseconds to wait=u32 50) -> ()  [unwired: 1 out]
        n182 = local read "Output waveform"() -> (w864:waveform(dbl))
        n183 = local read "Input waveform"() -> (w865:waveform(dbl))
        n184 = Build Array(w864, w865) -> (→"CONTROLS":waveform(dbl)[])
        n185 = local read "Finished"() -> (w863:bool)
        n186 = local read "stop"() -> (w858:bool)
        n187 = local read "Testing"() -> (w859:bool)
        n188 = local read "error?"() -> (w866:bool)
        n189 = And(x=w863, y=w858) -> (x .and. y?=w860:bool)
        n190 = And(x=w858, y=w859) -> (x .and. y?=w857:bool)
        n191 = Or(x=w860, y=w857) -> (x .or. y?=w861:bool)
        n192 = Or(x=w866, y=w861) -> (x .or. y?=w867:bool)
      }
      n193 = call "new counter entry.vi"("error in"=w64) -> ("error out"=w81:errorcluster, "Integer Time"=w80:i64)  [unwired: 9 in]
      n194 = call-poly <vilib>:"DAQmx Create Virtual Channel.vi"("counter"="Det1", "error in"=w64) -> ("task out"=w97:refnum<k21>, "error out"=w90:errorcluster)  [unwired: 12 in]
      n195 = call-poly <vilib>:"DAQmx Create Virtual Channel.vi"("counter"="Det2", "error in"=w64) -> ("task out"=w96:refnum<k21>, "error out"=w91:errorcluster)  [unwired: 12 in]
      n196 = call-poly <vilib>:"DAQmx Create Virtual Channel.vi"("counter"="Det3", "error in"=w64) -> ("task out"=w95:refnum<k21>, "error out"=w94:errorcluster)  [unwired: 12 in]
      n197 = call-poly <vilib>:"DAQmx Create Virtual Channel.vi"("counter"="PSU", "error in"=w64) -> ("task out"=w93:refnum<k21>, "error out"=w92:errorcluster)  [unwired: 12 in]
      n198 = Index Array(array=w59, index #1=0 ("index"), index #2=1 ("index"), index #3=2 ("index")) -> (element #1=w56:i16, element #2=w55:i16, element #3=w46:i16)
      n199 = call-poly <vilib>:"DAQmx Create Virtual Channel.vi"("maximum value"=10.0 ("Maximum Value"), "minimum value"=-2.5 ("Minimum Value"), "physical channels"="Physical Input Channels", "error in"=w64) -> ("task out"=w68:refnum<k21>, "error out"=w67:errorcluster)  [unwired: 10 in]
      n200 = call-poly <vilib>:"DAQmx Create Virtual Channel.vi"("maximum value"=10.0 ("Maximum Value"), "minimum value"=0.0 ("Minimum Value"), "physical channels"="Physical Channels", "error in"=w64) -> ("task out"=w141:refnum<k21>, "error out"=w140:errorcluster)  [unwired: 10 in]
      n201 = Get Date/Time In Seconds() -> (seconds since 1Jan1904=w79:timestamp)
      n202 = Initialize Array(0.0 ("element"), w56, w55, w46) -> (w60:dbl[][][])
      n203 = call <vilib>:"DAQmx Start Task.vi"("task/channels in"=w97, "error in"=w90) -> ("task out"=w121:refnum<k21>, "error out"=w114:errorcluster)  [unwired: 12 in]
      n204 = call <vilib>:"DAQmx Start Task.vi"("task/channels in"=w96, "error in"=w91) -> ("task out"=w120:refnum<k21>, "error out"=w115:errorcluster)  [unwired: 12 in]
      n205 = call <vilib>:"DAQmx Start Task.vi"("task/channels in"=w95, "error in"=w94) -> ("task out"=w119:refnum<k21>, "error out"=w116:errorcluster)  [unwired: 12 in]
      n206 = call <vilib>:"DAQmx Start Task.vi"("task/channels in"=w93, "error in"=w92) -> ("task out"=w118:refnum<k21>, "error out"=w117:errorcluster)  [unwired: 12 in]
      n207 = To Double Precision Float(number=w79) -> (double precision float=w78:dbl)
      n208 = call-poly <vilib>:"DAQmx Timing.vi"("task/channels in"=w68, "rate"=5000.0, "error in"=w67) -> ("task out"=w73:refnum<k21>, "error out"=w72:errorcluster)  [unwired: 11 in]
      n209 = local write "Width (ms) : 0.1"(0.0 ("Width (ms) : 3.5")) -> ()
      n210 = while {
        shift-right: [w283] -> _
        shift-left: w80 -> [w285]
        shift-right: [w275] -> _
        shift-left: w78 -> [w270]
        shift-right: [w274] -> _
        shift-left: w44 -> [w281]
        shift-right: [w273] -> _
        shift-left: w44 -> [w280]
        shift-right: [w272] -> _
        shift-left: w44 -> [w279]
        shift-right: [w252] -> _
        shift-left: w48 -> [w248]
        shift-right: [w251] -> _
        shift-left: w48 -> [w247]
        shift-right: [w253] -> _
        shift-left: w60 -> [w254]
        shift-right: [w250] -> _
        shift-left: w45 -> [w246]
        shift-right: [w249] -> _
        shift-left: w45 -> [w245]
        shift-right: [w242] -> _
        shift-left: w45 -> [w241]
        shift-right: [w235] -> _
        shift-left: TRUE -> [w236]
        shift-right: [w305] -> w113
        shift-left: w121 -> [w293]
        shift-right: [w295] -> w112
        shift-left: w114 -> [w292]
        shift-right: [w304] -> w111
        shift-left: w120 -> [w291]
        shift-right: [w301] -> w110
        shift-left: w115 -> [w290]
        shift-right: [w303] -> w109
        shift-left: w119 -> [w289]
        shift-right: [w300] -> w108
        shift-left: w116 -> [w288]
        shift-right: [w302] -> w107
        shift-left: w118 -> [w287]
        shift-right: [w299] -> w106
        shift-left: w117 -> [w286]
        shift-right: [w294] -> w88
        shift-left: w81 -> [w284]
        shift-right: [w213] -> _
        shift-left: w48 -> [w212]
        shift-right: [w208] -> _
        shift-left: w45 -> [w223]
        i -> [w226]
        stop <- w296 stop-if-true
        w183 = T10 {"Minimum"=0.0, "Maximum"=0.0, "Increment"=0.0, "Minor Increment"=0.0, "Start"=0.0} ("Scale.Range")
        w184 = T11 {"Minimum"=0.0, "Maximum"=0.0, "Increment"=0.0} ("Data Entry Limits")
        w298 = u32 100  # millisecond multiple
        n211 = local read "stop"() -> (w269:bool)
        n212 = local read "On/Off"() -> (w225:bool)
        n213 = Not(x=w269) -> (.not. x?=w268:bool)
        n214 = Quotient & Remainder(x=w226, y="Cycles to Avg.") -> (x-y*floor(x/y)=w271:i32)  [unwired: 1 out]
        n215 = And(x=w268, y=w225) -> (x .and. y?=w265:bool)
        n216 = Equal To 0?(x=w271) -> (x = 0?=w266:bool)
        n217 = And(x=w266, y=w265) -> (x .and. y?=w267:bool)
        n218 = event shown="[1] \"Counters On/Off\": Value Change" {
          selector: _ -> [_ _]
          dyn-events: _ -> [_ _]
          timeout: 0 -> [_ _]
          tunnel: [w413 w486] -> w305
          tunnel: [w408 w484] -> w304
          tunnel: [w407 w482] -> w303
          tunnel: [w406 w480] -> w302
          tunnel: [w405 w483] -> w301
          tunnel: [w404 w481] -> w300
          tunnel: [w403 w479] -> w299
          tunnel: [w394 w485] -> w295
          tunnel: [w393 w471] -> w294
          tunnel: w293 -> [w389 w475]
          tunnel: w292 -> [w388 w490]
          tunnel: w291 -> [w387 w476]
          tunnel: w290 -> [w386 w489]
          tunnel: w289 -> [w385 w477]
          tunnel: w288 -> [w384 w488]
          tunnel: w287 -> [w383 w478]
          tunnel: w286 -> [w382 w487]
          tunnel: w285 -> [w372 w474]
          tunnel: w284 -> [w371 w472]
          tunnel: [w369 w473] -> w283
          tunnel: [w365 w470] -> w278
          tunnel: [w364 w470] -> w277
          tunnel: [w363 w470] -> w276
          event Timeout {
            # "Counter Loop"
            n219 = event-data() -> ()  [unwired: 1 in, 2 out]
            n220 = case shown="True" "Reset Counters" {
              tunnel: w389 -> [w442 w469]
              tunnel: [w442 w467] -> w381
              tunnel: w388 -> [w441 w466]
              tunnel: [w441 w464] -> w380
              tunnel: w387 -> [w440 w463]
              tunnel: [w440 w461] -> w379
              tunnel: w386 -> [w439 w460]
              tunnel: [w439 w458] -> w378
              tunnel: w385 -> [w438 w457]
              tunnel: [w438 w455] -> w377
              tunnel: w384 -> [w437 w454]
              tunnel: [w437 w452] -> w376
              tunnel: w383 -> [w436 w451]
              tunnel: [w436 w449] -> w375
              tunnel: w382 -> [w435 w448]
              tunnel: [w435 w446] -> w374
              tunnel: w371 -> [w434 w444]
              tunnel: [w433 w445] -> w369
              tunnel: [w434 w443] -> w370
              tunnel: w372 -> [w433 _]
              frame False {
              }
              frame True {
                n221 = call <vilib>:"DAQmx Stop Task.vi"("task/channels in"=w457, "error in"=w454) -> ("task out"=w456:refnum<k21>, "error out"=w453:errorcluster)  [unwired: 12 in]
                n222 = call <vilib>:"DAQmx Stop Task.vi"("task/channels in"=w463, "error in"=w460) -> ("task out"=w462:refnum<k21>, "error out"=w459:errorcluster)  [unwired: 12 in]
                n223 = call <vilib>:"DAQmx Stop Task.vi"("task/channels in"=w451, "error in"=w448) -> ("task out"=w450:refnum<k21>, "error out"=w447:errorcluster)  [unwired: 12 in]
                n224 = call <vilib>:"DAQmx Stop Task.vi"("task/channels in"=w469, "error in"=w466) -> ("task out"=w468:refnum<k21>, "error out"=w465:errorcluster)  [unwired: 12 in]
                n225 = call "new counter entry.vi"("error in"=w444) -> ("error out"=w443:errorcluster, "Integer Time"=w445:i64)  [unwired: 9 in]
                n226 = call <vilib>:"DAQmx Start Task.vi"("task/channels in"=w450, "error in"=w447) -> ("task out"=w449:refnum<k21>, "error out"=w446:errorcluster)  [unwired: 12 in]
                n227 = call <vilib>:"DAQmx Start Task.vi"("task/channels in"=w456, "error in"=w453) -> ("task out"=w455:refnum<k21>, "error out"=w452:errorcluster)  [unwired: 12 in]
                n228 = call <vilib>:"DAQmx Start Task.vi"("task/channels in"=w462, "error in"=w459) -> ("task out"=w461:refnum<k21>, "error out"=w458:errorcluster)  [unwired: 12 in]
                n229 = call <vilib>:"DAQmx Start Task.vi"("task/channels in"=w468, "error in"=w465) -> ("task out"=w467:refnum<k21>, "error out"=w464:errorcluster)  [unwired: 12 in]
              }
            }
            n230 = call-poly <vilib>:"DAQmx Read.vi"("task/channels in"=w377, "timeout"=10.0, "error in"=w376) -> ("task out"=w407:refnum<k21>, "data"=w363:u32, "error out"=w400:errorcluster)  [unwired: 10 in]
            "Det3" <- w363
            n231 = call-poly <vilib>:"DAQmx Read.vi"("task/channels in"=w381, "timeout"=10.0, "error in"=w380) -> ("task out"=w413:refnum<k21>, "data"=w365:u32, "error out"=w402:errorcluster)  [unwired: 10 in]
            "Det1" <- w365
            n232 = call-poly <vilib>:"DAQmx Read.vi"("task/channels in"=w375, "timeout"=10.0, "error in"=w374) -> ("task out"=w406:refnum<k21>, "data"=w364:u32, "error out"=w399:errorcluster)  [unwired: 10 in]
            "PSU" <- w364
            n233 = call-poly <vilib>:"DAQmx Read.vi"("task/channels in"=w379, "timeout"=10.0, "error in"=w378) -> ("task out"=w408:refnum<k21>, "data"=w390:u32, "error out"=w401:errorcluster)  [unwired: 10 in]
            "Det2" <- w390
            n234 = Divide(x=w390, y=w365) -> (x/y=→"Det2/Det1":dbl)
            n235 = Divide(x=w363, y=w364) -> (x/y=→"PSU/Det3":dbl)
            n236 = Divide(x=w363, y=w365) -> (x/y=→"Det3/Det1":dbl)
            n237 = Bundle("data"=w365, "data"=w390, "data"=w364, "data"=w363) -> (w362:T12)  [unwired: 1 in]
            n238 = Divide(x=w364, y=w390) -> (x/y=→"PSU/Det2":dbl)
            n239 = Cluster To Array(cluster=w362) -> (array=w361:u32[])
            n240 = Not Equal To 0?(x=w361) -> (x != 0?=w360:bool[])
            n241 = Or Array Elements(Boolean array=w360) -> (logical OR=w359:bool)
            n242 = case shown="True" w359 {
              tunnel: [w414 w420] -> w392
              tunnel: "WHERE integer_timestamp = %d;" ("condition") -> [_ w419]
              tunnel: w370 -> [w414 w417]
              tunnel: w369 -> [_ w416]
              tunnel: w362 -> [_ w415]
              frame False {
              }
              frame True {
                # "Counter DB stuff"
                n243 = call "connect in.vi"("error in (no error)"=w417) -> ("error out"=w423:errorcluster, "Database Connection"=w431:T8)  [unwired: 6 in, 1 out]
                n244 = Build Array("first_counter" ("string"), "second_counter" ("string"), "psu_counter" ("string"), "third_counter" ("string")) -> (w427:string[])
                n245 = Format Into String(format string=w419, w416) -> (resulting string=w418:string)  [unwired: 2 in, 1 out]
                n246 = call <vilib>:"DB Tools Update Data.vi"("condition"=w418, "flatten cluster? (F)"=FALSE ("create table? (F)"), "data"=w415, "error in (no error)"=w423, "columns"=w427, "table"="counter", "connection reference"=w431) -> ("error out"=w421:errorcluster, "connection reference out"=w429:T8)  [unwired: 3 in]
                n247 = call "connect out.vi"("error in (no error)"=w423, "connection reference"=w429) -> ("error out"=w422:errorcluster)  [unwired: 9 in]
                n248 = Merge Errors(w422, w421) -> (w420:errorcluster)
              }
            }
            n249 = call <vilib>:"Clear Errors.vi"("error in (no error)"=w402) -> ("error out"=w394:errorcluster)  [unwired: 6 in]
            n250 = call <vilib>:"Clear Errors.vi"("error in (no error)"=w401) -> ("error out"=w405:errorcluster)  [unwired: 6 in]
            n251 = call <vilib>:"Clear Errors.vi"("error in (no error)"=w400) -> ("error out"=w404:errorcluster)  [unwired: 6 in]
            n252 = call <vilib>:"Clear Errors.vi"("error in (no error)"=w399) -> ("error out"=w403:errorcluster)  [unwired: 6 in]
            n253 = call "counter_sum.vi"("error in"=w392) -> ("error IO"=w393:errorcluster, "Number of Hours"=→"Hours Run":dbl, "Third Detector Sum"=w368:i64, "First Detector Sum"=w367:i64)  [unwired: 7 in]
            "First detector since\nlast source change:" <- w367
            "Third detector since\nlast source change:" <- w368
            n254 = Divide(x=w368, y=w367) -> (x/y=→"Source Efficiency":dbl)
          }
          event "Counters On/Off": Value Change {
            w470 = u32 0 ("data")
            n255 = event-data() -> ("NewVal"=w491:bool)  [unwired: 1 in, 4 out]
            n256 = case shown="True" w491 {
              tunnel: w490 -> [w511 w523]
              tunnel: w489 -> [w509 w522]
              tunnel: w488 -> [w507 w521]
              tunnel: w487 -> [w505 w520]
              tunnel: [w497 w531] -> w486
              tunnel: [w498 w530] -> w485
              tunnel: [w499 w529] -> w484
              tunnel: [w500 w528] -> w483
              tunnel: [w501 w527] -> w482
              tunnel: [w502 w526] -> w481
              tunnel: [w504 w525] -> w480
              tunnel: [w503 w524] -> w479
              tunnel: w478 -> [w506 w519]
              tunnel: w477 -> [w508 w518]
              tunnel: w476 -> [w510 w517]
              tunnel: w475 -> [w512 w516]
              tunnel: w474 -> [_ w515]
              tunnel: [w496 w515] -> w473
              tunnel: w472 -> [w495 w514]
              tunnel: [w494 w514] -> w471
              frame False {
                n257 = call <vilib>:"DAQmx Stop Task.vi"("task/channels in"=w508, "error in"=w507) -> ("task out"=w501:refnum<k21>, "error out"=w502:errorcluster)  [unwired: 12 in]
                n258 = call <vilib>:"DAQmx Stop Task.vi"("task/channels in"=w510, "error in"=w509) -> ("task out"=w499:refnum<k21>, "error out"=w500:errorcluster)  [unwired: 12 in]
                n259 = call <vilib>:"DAQmx Stop Task.vi"("task/channels in"=w506, "error in"=w505) -> ("task out"=w504:refnum<k21>, "error out"=w503:errorcluster)  [unwired: 12 in]
                n260 = call <vilib>:"DAQmx Stop Task.vi"("task/channels in"=w512, "error in"=w511) -> ("task out"=w497:refnum<k21>, "error out"=w498:errorcluster)  [unwired: 12 in]
                n261 = call "new counter entry.vi"("error in"=w495) -> ("error out"=w494:errorcluster, "Integer Time"=w496:i64)  [unwired: 9 in]
                n262 = property on="Calibrate XY" class="Bool (strict)"("Value"=FALSE ("Calibrate XY"), "DisabledEnum"=T6."Disabled and Grayed Out" ("Disabled")) -> ()  [unwired: 2 in, 2 out]
              }
              frame True {
                n263 = call <vilib>:"DAQmx Start Task.vi"("task/channels in"=w516, "error in"=w523) -> ("task out"=w531:refnum<k21>, "error out"=w530:errorcluster)  [unwired: 12 in]
                n264 = call <vilib>:"DAQmx Start Task.vi"("task/channels in"=w517, "error in"=w522) -> ("task out"=w529:refnum<k21>, "error out"=w528:errorcluster)  [unwired: 12 in]
                n265 = call <vilib>:"DAQmx Start Task.vi"("task/channels in"=w518, "error in"=w521) -> ("task out"=w527:refnum<k21>, "error out"=w526:errorcluster)  [unwired: 12 in]
                n266 = call <vilib>:"DAQmx Start Task.vi"("task/channels in"=w519, "error in"=w520) -> ("task out"=w525:refnum<k21>, "error out"=w524:errorcluster)  [unwired: 12 in]
                n267 = property on="Calibrate XY" class="Bool (strict)"("DisabledEnum"=T6."Enabled" ("Disabled")) -> ()  [unwired: 2 in, 2 out]
              }
            }
          }
        }
        n268 = case shown="True" w267 {
          tunnel: w270 -> [w648 w704]
          tunnel: w281 -> [w639 w703]
          tunnel: w280 -> [w647 w702]
          tunnel: w279 -> [w646 w701]
          tunnel: w278 -> [_ w695]
          tunnel: w277 -> [_ w694]
          tunnel: w276 -> [_ w693]
          tunnel: [w648 w696] -> w275
          tunnel: [w639 w695] -> w274
          tunnel: [w647 w694] -> w273
          tunnel: [w646 w693] -> w272
          tunnel: w254 -> [w643 w688]
          tunnel: w248 -> [_ w676]
          tunnel: w247 -> [_ w675]
          tunnel: w246 -> [w645 w689]
          tunnel: w245 -> [w644 w670]
          tunnel: [w643 w687] -> w234
          tunnel: [w645 w686] -> w244
          tunnel: [w644 w685] -> w243
          tunnel: w241 -> [w642 w682]
          tunnel: [w642 w683] -> w239
          tunnel: w223 -> [w641 w673]
          tunnel: w212 -> [_ w677]
          tunnel: [w641 w674] -> w207
          frame False {
            n269 = local read "Tab Control"() -> (w640:T3)
            n270 = case shown="\"EXY Scan Data\"" w640 {
              frame "Controls", Default {
              }
              frame "EXY Scan Data" {
                w651 = u8 0 ("Z Scale.Scale Fit")
                n271 = local read "Einzel Slice"() -> (w661:dbl)
                n272 = local read "Einzel Vs"() -> (w664:dbl[])
                n273 = local read "Y Slice"() -> (w659:dbl)
                n274 = local read "X Vs"() -> (w663:dbl[])
                n275 = local read "Y Vs"() -> (w662:dbl[])
                n276 = local read "X Slice"() -> (w660:dbl)
                n277 = local read "Rate Data"() -> (w655:dbl[][][])
                n278 = Search 1D Array(1D array=w662, element=w659) -> (index of element=w658:i32)  [unwired: 1 in]
                n279 = Search 1D Array(1D array=w663, element=w660) -> (index of element=w657:i32)  [unwired: 1 in]
                n280 = Search 1D Array(1D array=w664, element=w661) -> (index of element=w656:i32)  [unwired: 1 in]
                n281 = Index Array(array=w655, index (dim 0)=w656) -> (element=w654:dbl[][])  [unwired: 2 in]
                n282 = Array Max & Min(array=w655) -> (max value=w650:dbl, min value=w649:dbl)  [unwired: 2 out]
                n283 = Index Array(array=w655, index (dim 1)=w657) -> (element=w653:dbl[][])  [unwired: 2 in]
                n284 = Index Array(array=w655, index (dim 2)=w658) -> (element=w652:dbl[][])  [unwired: 2 in]
                n285 = local write "Einzel Slice Data"(w654) -> ()
                n286 = local write "Y Slice Data"(w652) -> ()
                n287 = local write "X Slice Data"(w653) -> ()
                n288 = property on="X Slice Data" class="IntGraph (strict)"("ZScale.Maximum"=w650, "ZScale.Minimum"=w649, "ZScale.ScaleFit"=w651) -> ()  [unwired: 2 in, 2 out]
                n289 = property on="Y Slice Data" class="IntGraph (strict)"("ZScale.Maximum"=w650, "ZScale.Minimum"=w649, "ZScale.ScaleFit"=w651) -> ()  [unwired: 2 in, 2 out]
                n290 = property on="Einzel Slice Data" class="IntGraph (strict)"("ZScale.Maximum"=w650, "ZScale.Minimum"=w649, "ZScale.ScaleFit"=w651) -> ()  [unwired: 2 in, 2 out]
              }
            }
          }
          frame True {
            n291 = local read "# of Steps"() -> (w684:i16[])
            n292 = Get Date/Time In Seconds() -> (seconds since 1Jan1904=w705:timestamp)
            n293 = To Double Precision Float(number=w705) -> (double precision float=w696:dbl)
            n294 = Index Array(array=w684, index #1=1 ("index"), index #2=2 ("index")) -> (element #1=w667:i16, element #2=w666:i16)
            n295 = local read "Num Steps"() -> (w680:i16)
            n296 = Subtract(x=w696, y=w704) -> (x-y=w697:dbl)
            n297 = Subtract(x=w695, y=w703) -> (x-y=w700:u32)
            n298 = Decrement(x=w667) -> (x-1=w665:i16)
            n299 = Subtract(x=w694, y=w702) -> (x-y=w699:u32)
            n300 = Decrement(x=w680) -> (x-1=w679:i16)
            n301 = Less?(x=w673, y=w666) -> (x < y?=w672:bool)
            n302 = Equal?(x=w665, y=w670) -> (x = y?=w671:bool)
            n303 = Subtract(x=w693, y=w701) -> (x-y=w698:u32)
            n304 = Less?(x=w682, y=w679) -> (x < y?=w681:bool)
            n305 = Divide(x=w700, y=w697) -> (x/y=→"Det1 Rate":dbl)
            n306 = Divide(x=w699, y=w697) -> (x/y=→"PSU Rate":dbl)
            n307 = Divide(x=w698, y=w697) -> (x/y=w678:dbl)
            "Det3 Rate" <- w678
            n308 = local read "Calibrate XY"() -> (w690:bool)
            n309 = case shown="True" w690 {
              tunnel: w676 -> [_ w731]
              tunnel: w675 -> [_ w730]
              tunnel: w689 -> [w710 w753]
              tunnel: w670 -> [w709 w752]
              tunnel: w688 -> [w711 w751]
              tunnel: [w711 w742] -> w687
              tunnel: w678 -> [_ w750]
              tunnel: [w710 w749] -> w686
              tunnel: [w709 w748] -> w685
              tunnel: w682 -> [w708 w747]
              tunnel: [w708 w746] -> w683
              tunnel: w681 -> [_ w745]
              tunnel: w673 -> [w707 w744]
              tunnel: w677 -> [_ w738]
              tunnel: [w707 w732] -> w674
              tunnel: w672 -> [_ w729]
              tunnel: w671 -> [_ w728]
              frame False {
                n310 = local read "Tab Control"() -> (w706:T3)
                n311 = case shown="\"EXY Scan Data\"" w706 {
                  frame "Controls", Default {
                  }
                  frame "EXY Scan Data" {
                    w715 = u8 0 ("Z Scale.Scale Fit")
                    n312 = local read "Einzel Slice"() -> (w726:dbl)
                    n313 = local read "Einzel Vs"() -> (w727:dbl[])
                    n314 = local read "X Slice"() -> (w724:dbl)
                    n315 = local read "Y Slice"() -> (w722:dbl)
                    n316 = local read "X Vs"() -> (w725:dbl[])
                    n317 = local read "Y Vs"() -> (w723:dbl[])
                    n318 = Search 1D Array(1D array=w723, element=w722) -> (index of element=w719:i32)  [unwired: 1 in]
                    n319 = Search 1D Array(1D array=w725, element=w724) -> (index of element=w720:i32)  [unwired: 1 in]
                    n320 = Search 1D Array(1D array=w727, element=w726) -> (index of element=w721:i32)  [unwired: 1 in]
                    n321 = local read "Rate Data"() -> (w714:dbl[][][])
                    n322 = Index Array(array=w714, index (dim 0)=w721) -> (element=w718:dbl[][])  [unwired: 2 in]
                    n323 = Array Max & Min(array=w714) -> (max value=w713:dbl, min value=w712:dbl)  [unwired: 2 out]
                    n324 = Index Array(array=w714, index (dim 1)=w720) -> (element=w717:dbl[][])  [unwired: 2 in]
                    n325 = Index Array(array=w714, index (dim 2)=w719) -> (element=w716:dbl[][])  [unwired: 2 in]
                    n326 = local write "Einzel Slice Data"(w718) -> ()
                    n327 = local write "X Slice Data"(w717) -> ()
                    n328 = local write "Y Slice Data"(w716) -> ()
                    n329 = property on="Einzel Slice Data" class="IntGraph (strict)"("ZScale.Maximum"=w713, "ZScale.Minimum"=w712, "ZScale.ScaleFit"=w715) -> ()  [unwired: 2 in, 2 out]
                    n330 = property on="Y Slice Data" class="IntGraph (strict)"("ZScale.Maximum"=w713, "ZScale.Minimum"=w712, "ZScale.ScaleFit"=w715) -> ()  [unwired: 2 in, 2 out]
                    n331 = property on="X Slice Data" class="IntGraph (strict)"("ZScale.Maximum"=w713, "ZScale.Minimum"=w712, "ZScale.ScaleFit"=w715) -> ()  [unwired: 2 in, 2 out]
                  }
                }
              }
              frame True {
                n332 = case shown="True" w729 {
                  tunnel: w753 -> [w756 w805]
                  tunnel: w752 -> [w755 w790]
                  tunnel: w751 -> [w773 w804]
                  tunnel: w750 -> [w772 w788]
                  tunnel: [w756 w803] -> w749
                  tunnel: [w755 w802] -> w748
                  tunnel: w747 -> [w771 w792]
                  tunnel: [w770 w787] -> w746
                  tunnel: w745 -> [_ w801]
                  tunnel: w731 -> [w769 w800]
                  tunnel: w730 -> [w768 w799]
                  tunnel: w744 -> [w759 w798]
                  tunnel: [w767 w797] -> w742
                  tunnel: w738 -> [w766 w796]
                  tunnel: [w758 w795] -> w732
                  tunnel: w728 -> [_ w791]
                  frame True {
                    w761 = T5 4 items=["Get", "Set X", "Set Y", "Set XY", "Internal"] ("Ring")
                    n333 = Index Array(array=w766, index=w756) -> (element=w760:dbl)
                    n334 = Index Array(array=w769, index=w755) -> (element=w764:dbl)
                    n335 = Decrement(x=w759) -> (x-1=w757:i32)
                    n336 = Index Array(array=w768, index=w759) -> (element=w765:dbl)
                    n337 = property on="Einzel Voltage" class="DigNum (strict)"("Val(Sgnl)"=w760) -> ()  [unwired: 2 in, 2 out]
                    n338 = Less Than 0?(x=w757) -> (x < 0?=w754:bool)
                    n339 = call "XYVoltageFGV.vi"("X Voltage"=w764, "Y Voltage"=w765, "Ring"=w761) -> ("X Voltage 2"=w763:dbl, "Y Voltage 2"=w762:dbl)  [unwired: 5 in, 1 out]
                    n340 = property on="Y Voltage" class="DigNum (strict)"("Val(Sgnl)"=w762) -> ()  [unwired: 2 in, 2 out]
                    n341 = property on="X Voltage" class="DigNum (strict)"("Val(Sgnl)"=w763) -> ()  [unwired: 2 in, 2 out]
                    n342 = case shown="False" w754 {
                      tunnel: w773 -> [w783 w785]
                      tunnel: [w782 w785] -> w767
                      tunnel: w757 -> [w779 _]
                      tunnel: w755 -> [w780 _]
                      tunnel: w772 -> [w776 _]
                      tunnel: w771 -> [w778 w784]
                      tunnel: [w775 w784] -> w770
                      tunnel: w756 -> [w781 _]
                      frame False {
                        n343 = local read "Cal Test?"() -> (w774:bool)
                        n344 = Increment(x=w778) -> (x+1=w775:i32)
                        n345 = Select(t=w775, s=w774, f=w776) -> (s? t:f=w777:dbl)
                        n346 = Replace Array Subset(array=w783, new element=w777, index (dim 0)=w781, index (dim 1)=w780, index (dim 2)=w779) -> (w782:dbl[][][])
                      }
                      frame True {
                      }
                    }
                    n347 = Increment(x=w759) -> (x+1=w758:i32)
                  }
                  frame False {
                    n348 = Decrement(x=w798) -> (x-1=w793:i32)
                    n349 = Increment(x=w792) -> (x+1=w787:i32)
                    n350 = Select(t=w787, s="Cal Test?", f=w788) -> (s? t:f=w789:dbl)
                    n351 = Replace Array Subset(array=w804, new element=w789, index (dim 0)=w805, index (dim 1)=w790, index (dim 2)=w793) -> (w794:dbl[][][])
                    n352 = case shown="True" w801 {
                      tunnel: w800 -> [w810 w856]
                      tunnel: w799 -> [w809 w855]
                      tunnel: w805 -> [_ w839]
                      tunnel: w790 -> [_ w847]
                      tunnel: [w807 w844] -> w802
                      tunnel: w794 -> [w808 w849]
                      tunnel: [w808 w849] -> w797
                      tunnel: [w807 w841] -> w803
                      tunnel: w796 -> [w806 w848]
                      tunnel: w798 -> [_ _]
                      tunnel: [w807 w837] -> w795
                      tunnel: w791 -> [_ w840]
                      frame False {
                        w807 = 0
                        n353 = Less Or Equal To 0?(x=w808) -> (x <= 0?=w812:bool[][][])
                        n354 = And Array Elements(Boolean array=w812) -> (logical AND=w811:bool)
                        n355 = case shown="False" w811 {
                          tunnel: w808 -> [w830 _]
                          tunnel: w810 -> [w826 _]
                          tunnel: w809 -> [w825 _]
                          tunnel: w806 -> [w815 _]
                          frame False {
                            w822 = T5 4 items=["Get", "Set X", "Set Y", "Set XY", "Internal"] ("Ring")
                            n356 = Array Max & Min(array=w830) -> (max index (indices)=w829:i32[])  [unwired: 3 out]
                            n357 = Index Array(array=w829, index #1=0 ("index"), index #2=1 ("index"), index #3=2 ("index")) -> (element #1=w816:i32, element #2=w817:i32, element #3=w818:i32)
                            n358 = Index Array(array=w825, index=w818) -> (element=w824:dbl)
                            n359 = Index Array(array=w815, index=w816) -> (element=w814:dbl)
                            n360 = Index Array(array=w826, index=w817) -> (element=w823:dbl)
                            n361 = property on="Einzel Voltage" class="DigNum (strict)"("Val(Sgnl)"=w814) -> ()  [unwired: 2 in, 2 out]
                            n362 = call "XYVoltageFGV.vi"("X Voltage"=w823, "Y Voltage"=w824, "Ring"=w822) -> ("X Voltage 2"=w821:dbl, "Y Voltage 2"=w820:dbl)  [unwired: 5 in, 1 out]
                            n363 = property on="X Voltage" class="DigNum (strict)"("Val(Sgnl)"=w821) -> ()  [unwired: 2 in, 2 out]
                            n364 = property on="Y Voltage" class="DigNum (strict)"("Val(Sgnl)"=w820) -> ()  [unwired: 2 in, 2 out]
                          }
                          frame True {
                            w834 = T5 4 items=["Get", "Set X", "Set Y", "Set XY", "Internal"] ("Ring")
                            n365 = local read "Old Einzel"() -> (w831:dbl)
                            n366 = call "XYVoltageFGV.vi"("X Voltage"=0.0, "Y Voltage"=0.0, "Ring"=w834) -> ("X Voltage 2"=w833:dbl, "Y Voltage 2"=w832:dbl)  [unwired: 5 in, 1 out]
                            n367 = property on="X Voltage" class="DigNum (strict)"("Val(Sgnl)"=w833) -> ()  [unwired: 2 in, 2 out]
                            n368 = property on="Y Voltage" class="DigNum (strict)"("Val(Sgnl)"=w832) -> ()  [unwired: 2 in, 2 out]
                            n369 = property on="Einzel Voltage" class="DigNum (strict)"("Val(Sgnl)"=w831) -> ()  [unwired: 2 in, 2 out]
                          }
                        }
                        n370 = local write "Calibrate XY"(FALSE ("Calibrate XY")) -> ()
                      }
                      frame True {
                        w845 = 0
                        w850 = T5 4 items=["Get", "Set X", "Set Y", "Set XY", "Internal"] ("Ring")
                        n371 = Increment(x=w847) -> (x+1=w843:i32)
                        n372 = Increment(x=w839) -> (x+1=w838:i32)
                        n373 = Select(t=w838, s=w840, f=w839) -> (s? t:f=w841:i32)
                        n374 = Select(t=0, s=w840, f=w843) -> (s? t:f=w844:i32)
                        n375 = Index Array(array=w856, index=w844) -> (element=w853:dbl)
                        n376 = Index Array(array=w848, index=w841) -> (element=w846:dbl)
                        n377 = Increment(x=w845) -> (x+1=w837:i32)
                        n378 = Index Array(array=w855, index=w845) -> (element=w854:dbl)
                        n379 = call "XYVoltageFGV.vi"("X Voltage"=w853, "Y Voltage"=w854, "Ring"=w850) -> ("X Voltage 2"=w851:dbl, "Y Voltage 2"=w852:dbl)  [unwired: 5 in, 1 out]
                        n380 = property on="Y Voltage" class="DigNum (strict)"("Val(Sgnl)"=w852) -> ()  [unwired: 2 in, 2 out]
                        n381 = property on="X Voltage" class="DigNum (strict)"("Val(Sgnl)"=w851) -> ()  [unwired: 2 in, 2 out]
                        n382 = property on="Einzel Voltage" class="DigNum (strict)"("Val(Sgnl)"=w846) -> ()  [unwired: 2 in, 2 out]
                      }
                    }
                  }
                }
                "Rate Data" <- w742
                n383 = Search 1D Array(1D array=w731, element="X Slice") -> (index of element=w733:i32)  [unwired: 1 in]
                n384 = Search 1D Array(1D array=w730, element="Y Slice") -> (index of element=w734:i32)  [unwired: 1 in]
                n385 = Search 1D Array(1D array=w738, element="Einzel Slice") -> (index of element=w737:i32)  [unwired: 1 in]
                n386 = Index Array(array=w742, index (dim 0)=w737) -> (element=→"Einzel Slice Data":dbl[][])  [unwired: 2 in]
                n387 = Index Array(array=w742, index (dim 2)=w734) -> (element=→"Y Slice Data":dbl[][])  [unwired: 2 in]
                n388 = Index Array(array=w742, index (dim 1)=w733) -> (element=→"X Slice Data":dbl[][])  [unwired: 2 in]
              }
            }
          }
        }
        n389 = Unbundle By Name("Things to Scan") -> ("Einzel"=w176:bool, "X"=w175:bool, "Y"=w174:bool)
        n390 = case shown="False" w176 {
          tunnel: [w344 w356] -> w180
          tunnel: "Calibrate XY" -> [_ w353]
          frame False {
            w341 = 10.0 ("y")
            n391 = local read "Einzel Voltage"() -> (w351:dbl)
            n392 = local read "# of Steps"() -> (w348:i16[])
            n393 = Increment(x=w351) -> (x+1=w342:dbl)
            n394 = Less Or Equal?(x=w342, y=w341) -> (x <= y?=w343:bool)
            n395 = Select(t=w342, s=w343, f=w341) -> (s? t:f=w340:dbl)
            n396 = Replace Array Subset(array=w348, new element=i16 1 ("new element/subarray"), index=0) -> (w347:i16[])
            n397 = Build Array(w351, w340) -> (w350:dbl[])
            n398 = local write "# of Steps"(w347) -> ()
            n399 = property on="Ein. Range" class="Arr (strict)"("DisabledEnum"=2 ("element"), "Value"=w350) -> (error out=w344:errorcluster)  [unwired: 2 in, 1 out]
          }
          frame True {
            n400 = Select(t=2, s=w353, f=0 ("element")) -> (s? t:f=w354:i32)
            n401 = property on="Ein. Range" class="Arr (strict)"("DisabledEnum"=w354) -> (error out=w356:errorcluster)  [unwired: 2 in, 1 out]
          }
        }
        n402 = case shown="False" w175 {
          tunnel: [w327 w339] -> w181
          tunnel: "Calibrate XY" -> [_ w336]
          frame False {
            w325 = 2.5 ("y")
            n403 = local read "# of Steps"() -> (w331:i16[])
            n404 = local read "X Voltage"() -> (w334:dbl)
            n405 = Increment(x=w334) -> (x+1=w324:dbl)
            n406 = Less Or Equal?(x=w324, y=w325) -> (x <= y?=w326:bool)
            n407 = Select(t=w324, s=w326, f=w325) -> (s? t:f=w323:dbl)
            n408 = Replace Array Subset(array=w331, new element=i16 1 ("new element/subarray"), index=1) -> (w330:i16[])
            n409 = Build Array(w334, w323) -> (w333:dbl[])
            n410 = local write "# of Steps"(w330) -> ()
            n411 = property on="X Range" class="Arr (strict)"("DisabledEnum"=2 ("element"), "Value"=w333) -> (error out=w327:errorcluster)  [unwired: 2 in, 1 out]
          }
          frame True {
            n412 = Select(t=2, s=w336, f=0 ("element")) -> (s? t:f=w337:i32)
            n413 = property on="X Range" class="Arr (strict)"("DisabledEnum"=w337) -> (error out=w339:errorcluster)  [unwired: 2 in, 1 out]
          }
        }
        n414 = case shown="False" w174 {
          tunnel: [w310 w322] -> w182
          tunnel: "Calibrate XY" -> [_ w320]
          frame False {
            w308 = 2.5 ("y")
            n415 = local read "# of Steps"() -> (w314:i16[])
            n416 = local read "Y Voltage"() -> (w316:dbl)
            n417 = Increment(x=w316) -> (x+1=w307:dbl)
            n418 = Less Or Equal?(x=w307, y=w308) -> (x <= y?=w309:bool)
            n419 = Select(t=w307, s=w309, f=w308) -> (s? t:f=w306:dbl)
            n420 = Replace Array Subset(array=w314, new element=i16 1 ("new element/subarray"), index=2) -> (w313:i16[])
            n421 = Build Array(w316, w306) -> (w317:dbl[])
            n422 = local write "# of Steps"(w313) -> ()
            n423 = property on="Y Range" class="Arr (strict)"("DisabledEnum"=2 ("element"), "Value"=w317) -> (error out=w310:errorcluster)  [unwired: 2 in, 1 out]
          }
          frame True {
            n424 = Select(t=2, s=w320, f=0 ("element")) -> (s? t:f=w321:i32)
            n425 = property on="Y Range" class="Arr (strict)"("DisabledEnum"=w321) -> (error out=w322:errorcluster)  [unwired: 2 in, 1 out]
          }
        }
        n426 = call-poly <userlib>:"Data Changed__ogtk.vi"("Boolean"="Calibrate XY") -> ("Changed"=w196:bool)
        n427 = And(x=w196, y="Calibrate XY") -> (x .and. y?=w197:bool)
        n428 = Index Array(array="# of Steps", index #1=0 ("index"), index #2=1 ("index"), index #3=2 ("index")) -> (element #1=w158:i16, element #2=w160:i16, element #3=w163:i16)
        n429 = Multiply Array Elements(1:"# of Steps") -> (0:w240:i16)
        "Num Steps" <- w240
        n430 = case shown="True" w197 {
          frame False {
          }
          frame True {
            n431 = local read "Einzel Voltage"() -> (→"Old Einzel":dbl)
          }
        }
        n432 = Subtract(x=w240, y=w239) -> (x-y=→"Steps to go":i32)
        n433 = Merge Errors(w180, w181, w182) -> (w179:errorcluster)
        n434 = Decrement(x=w158) -> (x-1=w188:i16)
        n435 = Index Array(array="Ein. Range", index #1=0 ("index"), index #2=1 ("index")) -> (element #1=w220:dbl, element #2=w219:dbl)
        n436 = Index Array(array="X Range", index #1=0 ("index"), index #2=1 ("index")) -> (element #1=w263:dbl, element #2=w264:dbl)
        n437 = Decrement(x=w160) -> (x-1=w229:i16)
        n438 = Index Array(array="Y Range", index #1=0 ("index"), index #2=1 ("index")) -> (element #1=w262:dbl, element #2=w261:dbl)
        n439 = Subtract(x=w220, y=w219) -> (x-y=w218:dbl)
        n440 = Decrement(x=w163) -> (x-1=w231:i16)
        n441 = Equal To 0?(x=w188) -> (x = 0?=w187:bool)
        n442 = Subtract(x=w263, y=w264) -> (x-y=w259:dbl)
        n443 = Subtract(x=w262, y=w261) -> (x-y=w260:dbl)
        n444 = Equal To 0?(x=w229) -> (x = 0?=w186:bool)
        n445 = Array Max & Min(array="Y Range") -> (max value=w203:dbl, min value=w202:dbl)  [unwired: 2 out]
        n446 = Array Max & Min(array="X Range") -> (max value=w201:dbl, min value=w200:dbl)  [unwired: 2 out]
        n447 = Equal To 0?(x=w231) -> (x = 0?=w185:bool)
        n448 = Select(t=i16 1, s=w187, f=w188) -> (s? t:f=w216:i16)
        n449 = Select(t=i16 1, s=w186, f=w229) -> (s? t:f=w227:i16)
        n450 = Array Max & Min(array="Ein. Range") -> (max value=w206:dbl, min value=w205:dbl)  [unwired: 2 out]
        n451 = Divide(x=w259, y=w227) -> (x/y=w258:dbl)
        n452 = Divide(x=w218, y=w216) -> (x/y=w215:dbl)
        n453 = Select(t=i16 1, s=w185, f=w231) -> (s? t:f=w230:i16)
        n454 = Absolute Value(x=w258) -> (abs(x)=w169:dbl)
        n455 = Absolute Value(x=w215) -> (abs(x)=w172:dbl)
        n456 = Divide(x=w260, y=w230) -> (x/y=w257:dbl)
        n457 = Absolute Value(x=w257) -> (abs(x)=w165:dbl)
        n458 = Equal To 0?(x=w172) -> (x = 0?=w157:bool)
        n459 = Equal To 0?(x=w169) -> (x = 0?=w161:bool)
        n460 = Equal To 0?(x=w165) -> (x = 0?=w164:bool)
        n461 = Select(t=0.1, s=w157, f=w172) -> (s? t:f=w171:dbl)
        n462 = Select(t=0.1, s=w161, f=w169) -> (s? t:f=w168:dbl)
        n463 = Select(t=i16 1, s=w157, f=w158) -> (s? t:f=w155:i16)
        n464 = Select(t=i16 1, s=w161, f=w160) -> (s? t:f=w154:i16)
        n465 = Select(t=0.1, s=w164, f=w165) -> (s? t:f=w166:dbl)
        n466 = Bundle(cluster=w183, "Minimum"=w200, "Maximum"=w201, "Increment"=w168, "Minor Increment"=w168, "Start"=w200) -> (w199:T10)
        n467 = Bundle(cluster=w184, "Minimum"=w200, "Maximum"=w201, "Increment"=w168) -> (w211:T11)
        n468 = Select(t=i16 1, s=w164, f=w163) -> (s? t:f=w153:i16)
        n469 = Bundle(cluster=w184, "Minimum"=w202, "Maximum"=w203, "Increment"=w166) -> (w210:T11)
        n470 = Bundle(cluster=w183, "Minimum"=w202, "Maximum"=w203, "Increment"=w166, "Minor Increment"=w166, "Start"=w202) -> (w198:T10)
        n471 = Bundle(cluster=w184, "Minimum"=w205, "Maximum"=w206, "Increment"=w171) -> (w209:T11)
        n472 = Bundle(cluster=w183, "Minimum"=w205, "Maximum"=w206, "Increment"=w171, "Minor Increment"=w171, "Start"=w205) -> (w204:T10)
        n473 = Build Array(w155, w154, w153) -> (w152:i16[])
        n474 = case shown="True" "Calibrate XY" {
          tunnel: w153 -> [w534 w601]
          tunnel: w202 -> [_ w592]
          tunnel: w200 -> [_ w587]
          tunnel: w168 -> [_ w597]
          tunnel: w166 -> [_ w591]
          tunnel: [w536 w589] -> w252
          tunnel: [w536 w590] -> w251
          tunnel: [w538 w605] -> w253
          tunnel: [w537 w604] -> w250
          tunnel: [w537 w603] -> w249
          tunnel: w234 -> [_ w605]
          tunnel: w244 -> [_ w604]
          tunnel: w243 -> [_ w603]
          tunnel: w154 -> [w533 w602]
          tunnel: [w537 w600] -> w242
          tunnel: w239 -> [_ w600]
          tunnel: w236 -> [_ w586]
          tunnel: [TRUE FALSE] -> w235
          tunnel: w205 -> [_ w593]
          tunnel: w171 -> [_ w596]
          tunnel: w155 -> [w535 w595]
          tunnel: [w536 w594] -> w213
          tunnel: w211 -> [_ w583]
          tunnel: w210 -> [_ w582]
          tunnel: w209 -> [_ w584]
          tunnel: w207 -> [_ w588]
          tunnel: [w537 w588] -> w208
          tunnel: w204 -> [_ w559]
          tunnel: w199 -> [_ w551]
          tunnel: w198 -> [_ w543]
          tunnel: w187 -> [_ w568]
          tunnel: w186 -> [_ w567]
          tunnel: w185 -> [_ w566]
          tunnel: w179 -> [_ _]
          frame False {
            w532 = T6."Enabled" ("Disabled")
            w537 = 0
            w536 = dbl[] []
            n475 = property on="# of Steps" class="Arr (strict)"("DisabledEnum"=w532) -> ()  [unwired: 2 in, 2 out]
            n476 = property on="X Voltage" class="DigNum (strict)"("DisabledEnum"=w532) -> ()  [unwired: 2 in, 2 out]
            n477 = property on="Y Voltage" class="DigNum (strict)"("DisabledEnum"=w532) -> ()  [unwired: 2 in, 2 out]
            n478 = property on="Things to Scan" class="Clust (strict)"("DisabledEnum"=w532) -> ()  [unwired: 2 in, 2 out]
            n479 = property on="Einzel Voltage" class="DigNum (strict)"("DisabledEnum"=w532) -> ()  [unwired: 2 in, 2 out]
            n480 = Initialize Array(0.0 ("element"), w535, w533, w534) -> (w538:dbl[][][])
          }
          frame True {
            w569 = u8 1 ("Z Scale.Scale Fit")
            w541 = T6."Disabled and Grayed Out" ("Disabled")
            n481 = for {
              N: w602 -> [_]
              tunnel: w597 -> [w637]
              tunnel: w587 -> [w635]
              tunnel: [w634] -> w589 mode=indexing
              i -> [w638]
              n482 = Multiply(x=w637, y=w638) -> (x*y=w636:dbl)
              n483 = Add(x=w635, y=w636) -> (x+y=w634:dbl)
            }
            "X Vs" <- w589
            n484 = for {
              N: w595 -> [_]
              tunnel: w596 -> [w624]
              tunnel: w593 -> [w623]
              tunnel: [w621] -> w594 mode=indexing
              i -> [w625]
              n485 = Multiply(x=w624, y=w625) -> (x*y=w622:dbl)
              n486 = Add(x=w623, y=w622) -> (x+y=w621:dbl)
            }
            "Einzel Vs" <- w594
            n487 = for {
              N: w601 -> [_]
              tunnel: w591 -> [w632]
              tunnel: w592 -> [w631]
              tunnel: [w629] -> w590 mode=indexing
              i -> [w633]
              n488 = Multiply(x=w632, y=w633) -> (x*y=w630:dbl)
              n489 = Add(x=w631, y=w630) -> (x+y=w629:dbl)
            }
            "Y Vs" <- w590
            n490 = Equal To 0?(x=w600) -> (x = 0?=w585:bool)
            n491 = And(x=w585, y=w586) -> (x .and. y?=w599:bool)
            n492 = case shown="True" w599 {
              tunnel: w587 -> [_ w628]
              tunnel: w592 -> [_ w627]
              tunnel: w593 -> [_ w626]
              frame False {
              }
              frame True {
                n493 = property on="X Voltage" class="DigNum (strict)"("Val(Sgnl)"=w628) -> ()  [unwired: 2 in, 2 out]
                n494 = property on="Einzel Voltage" class="DigNum (strict)"("Val(Sgnl)"=w626) -> ()  [unwired: 2 in, 2 out]
                n495 = property on="Y Voltage" class="DigNum (strict)"("Val(Sgnl)"=w627) -> ()  [unwired: 2 in, 2 out]
              }
            }
            n496 = property on="Einzel Slice" class="Slide (strict)"("Data Range"=w584, "Scale.Range"=w559) -> ()  [unwired: 2 in, 2 out]
            n497 = property on="X Slice" class="Slide (strict)"("Data Range"=w583, "Scale.Range"=w551) -> ()  [unwired: 2 in, 2 out]
            n498 = property on="Y Slice" class="Slide (strict)"("Data Range"=w582, "Scale.Range"=w543) -> ()  [unwired: 2 in, 2 out]
            n499 = property on="Einzel Voltage" class="DigNum (strict)"("DisabledEnum"=w541) -> ()  [unwired: 2 in, 2 out]
            n500 = property on="Ein. Range" class="Arr (strict)"("DisabledEnum"=w541) -> ()  [unwired: 2 in, 2 out]
            n501 = property on="X Range" class="Arr (strict)"("DisabledEnum"=w541) -> ()  [unwired: 2 in, 2 out]
            n502 = Unbundle(w584) -> ("Minimum"=w581:dbl, "Increment"=w580:dbl)  [unwired: 1 out]
            n503 = Unbundle(w582) -> ("Minimum"=w577:dbl, "Increment"=w576:dbl)  [unwired: 1 out]
            n504 = Unbundle(w583) -> ("Minimum"=w579:dbl, "Increment"=w578:dbl)  [unwired: 1 out]
            n505 = Bundle("Minimum"=w581, "Increment"=w580) -> (w575:cluster{"Minimum":dbl, "Increment":dbl})  [unwired: 1 in]
            n506 = Bundle("Minimum"=w579, "Increment"=w578) -> (w574:cluster{"Minimum":dbl, "Increment":dbl})  [unwired: 1 in]
            n507 = Bundle("Minimum"=w577, "Increment"=w576) -> (w573:cluster{"Minimum":dbl, "Increment":dbl})  [unwired: 1 in]
            n508 = property on="Y Range" class="Arr (strict)"("DisabledEnum"=w541) -> ()  [unwired: 2 in, 2 out]
            n509 = property on="Y Voltage" class="DigNum (strict)"("DisabledEnum"=w541) -> ()  [unwired: 2 in, 2 out]
            n510 = Unbundle(w543) -> ("Minimum"=w549:dbl, "Maximum"=w548:dbl, "Increment"=w546:dbl, "Minor Increment"=w545:dbl, "Start"=w544:dbl)
            n511 = Unbundle(w559) -> ("Minimum"=w565:dbl, "Maximum"=w564:dbl, "Increment"=w562:dbl, "Minor Increment"=w561:dbl, "Start"=w560:dbl)
            n512 = Unbundle(w551) -> ("Minimum"=w557:dbl, "Maximum"=w556:dbl, "Increment"=w554:dbl, "Minor Increment"=w553:dbl, "Start"=w552:dbl)
            n513 = property on="# of Steps" class="Arr (strict)"("DisabledEnum"=w541) -> ()  [unwired: 2 in, 2 out]
            n514 = property on="X Voltage" class="DigNum (strict)"("DisabledEnum"=w541) -> ()  [unwired: 2 in, 2 out]
            n515 = Add(x=w548, y=w546) -> (x+y=w547:dbl)
            n516 = Add(x=w564, y=w562) -> (x+y=w563:dbl)
            n517 = Add(x=w556, y=w554) -> (x+y=w555:dbl)
            n518 = Bundle("Minimum"=w549, w547, "Increment"=w546, "Minor Increment"=w545, "Start"=w544) -> (w542:T13)  [unwired: 1 in]
            n519 = Bundle("Minimum"=w565, w563, "Increment"=w562, "Minor Increment"=w561, "Start"=w560) -> (w558:T13)  [unwired: 1 in]
            n520 = Bundle("Minimum"=w557, w555, "Increment"=w554, "Minor Increment"=w553, "Start"=w552) -> (w550:T13)  [unwired: 1 in]
            n521 = property on="Things to Scan" class="Clust (strict)"("DisabledEnum"=w541) -> ()  [unwired: 2 in, 2 out]
            n522 = case shown="False" w568 {
              tunnel: w558 -> [w616 w618]
              tunnel: [w616 w618] -> w572
              frame False {
                n523 = property on="Einzel Slice" class="Slide (strict)"("DisabledEnum"=0) -> ()  [unwired: 2 in, 2 out]
              }
              frame True {
                n524 = Unbundle By Name(w618) -> ("Minimum"=w619:dbl)
                n525 = property on="Einzel Slice" class="Slide (strict)"("DisabledEnum"=2, "Value"=w619) -> ()  [unwired: 2 in, 2 out]
              }
            }
            n526 = case shown="False" w567 {
              tunnel: w550 -> [w611 w614]
              tunnel: [w611 w614] -> w571
              frame False {
                n527 = property on="X Slice" class="Slide (strict)"("DisabledEnum"=0) -> ()  [unwired: 2 in, 2 out]
              }
              frame True {
                n528 = Unbundle By Name(w614) -> ("Minimum"=w613:dbl)
                n529 = property on="X Slice" class="Slide (strict)"("DisabledEnum"=2, "Value"=w613) -> ()  [unwired: 2 in, 2 out]
              }
            }
            n530 = case shown="False" w566 {
              tunnel: w542 -> [w606 w609]
              tunnel: [w606 w609] -> w570
              frame False {
                n531 = property on="Y Slice" class="Slide (strict)"("DisabledEnum"=0) -> ()  [unwired: 2 in, 2 out]
              }
              frame True {
                n532 = Unbundle By Name(w609) -> ("Minimum"=w608:dbl)
                n533 = property on="Y Slice" class="Slide (strict)"("DisabledEnum"=2, "Value"=w608) -> ()  [unwired: 2 in, 2 out]
              }
            }
            n534 = property on="Y Slice Data" class="IntGraph (strict)"("XScale.Ofst&Mult"=w575, "XScale.Range"=w572, "YScale.Ofst&Mult"=w574, "YScale.Range"=w571, "ZScale.ScaleFit"=w569) -> ()  [unwired: 2 in, 2 out]
            n535 = property on="X Slice Data" class="IntGraph (strict)"("XScale.Ofst&Mult"=w575, "XScale.Range"=w572, "YScale.Ofst&Mult"=w573, "YScale.Range"=w570, "ZScale.ScaleFit"=w569) -> ()  [unwired: 2 in, 2 out]
            n536 = property on="Einzel Slice Data" class="IntGraph (strict)"("XScale.Ofst&Mult"=w574, "XScale.Range"=w571, "YScale.Ofst&Mult"=w573, "YScale.Range"=w570, "ZScale.ScaleFit"=w569) -> ()  [unwired: 2 in, 2 out]
          }
        }
        n537 = local write "# of Steps"(w152) -> ()
        n538 = Wait Until Next ms Multiple(millisecond multiple=w298) -> ()  [unwired: 1 out]
        n539 = local read "stop"() -> (w232:bool)
        n540 = local read "error?"() -> (w297:bool)
        n541 = Or(x=w232, y=w297) -> (x .or. y?=w296:bool)
      }
      n542 = property class="DAQmx Write"(reference=w141, error in=w140, "Regeneration Mode"=w142) -> (reference out=w138:refnum<k21>, error out=w137:errorcluster)
      n543 = property class="DAQmx Read"(reference=w73, error in=w72, "ReadAllAvailSamp"=w75, "AutoStart"=w75, "OverWrite"=w74) -> (reference out=w65:refnum<k21>, error out=w63:errorcluster)
      n544 = while {
        shift-right: [w879] -> w62
        shift-left: w65 -> [w880]
        shift-right: [w881] -> w77
        shift-left: w63 -> [w877]
        stop <- w878 stop-if-true
        w885 = 2
        # "Monitoring Loop"
        n545 = local read "stop"() -> (w874:bool)
        n546 = local read "Finished"() -> (w900:bool)
        n547 = call <vilib>:"DAQmx Start Task.vi"("task/channels in"=w880, "error in"=w877) -> ("task out"=w886:refnum<k21>, "error out"=w887:errorcluster)  [unwired: 12 in]
        n548 = local read "Testing"() -> (w876:bool)
        n549 = And(x=w874, y=w900) -> (x .and. y?=w899:bool)
        n550 = call-poly <vilib>:"DAQmx Read.vi"("task/channels in"=w886, "number of samples per channel"=1000, "error in"=w887) -> ("task out"=w888:refnum<k21>, "data"=w883:waveform(dbl)[], "error out"=w889:errorcluster)  [unwired: 10 in]
        n551 = local read "error?"() -> (w884:bool)
        n552 = And(x=w876, y=w874) -> (x .and. y?=w875:bool)
        n553 = call <vilib>:"DAQmx Stop Task.vi"("task/channels in"=w888, "error in"=w889) -> ("task out"=w879:refnum<k21>, "error out"=w898:errorcluster)  [unwired: 12 in]
        n554 = Index Array(array=w883) -> (element #1=w873:waveform(dbl), element #2=w872:waveform(dbl), element #3=w871:waveform(dbl), element #4=w870:waveform(dbl), element #5=w869:waveform(dbl))  [unwired: 5 in]
        "Input waveform" <- w873
        n555 = Or(x=w884, y=w899) -> (x .or. y?=w882:bool)
        n556 = Or(x=w875, y=w882) -> (x .or. y?=w878:bool)
        n557 = Multiply(x=w871, y=w885) -> (x*y=w894:waveform(dbl))
        n558 = Multiply(x=w872, y=w885) -> (x*y=w892:waveform(dbl))
        n559 = call-poly <vilib>:"Mean.vi"("X"=w869) -> ("mean"=→"Actual Steerer X (kV)":dbl)  [unwired: 1 out]
        n560 = call-poly <vilib>:"Mean.vi"("X"=w870) -> ("mean"=→"Actual Steerer Y (kV)":dbl)  [unwired: 1 out]
        n561 = call-poly <vilib>:"Amplitude and Levels.vi"("error in (no error)"=w898, "signal in"=w873) -> ("error out"=w881:errorcluster, "amplitude"=→"Actual Amplitude (V) 2":dbl)  [unwired: 6 in, 2 out]
        n562 = call-poly <vilib>:"Mean.vi"("X"=w894) -> ("mean"=→"Actual Needle (kV)":dbl)  [unwired: 1 out]
        n563 = call-poly <vilib>:"Mean.vi"("X"=w892) -> ("mean"=→"Actual Einzel (kV)":dbl)  [unwired: 1 out]
      }
      n564 = call-poly <vilib>:"DAQmx Timing.vi"("task/channels in"=w138, "sample mode"=w151, "rate"=250000.0 ("Sample Clock Rate"), "error in"=w137) -> ("task out"=w145:refnum<k21>, "error out"=w126:errorcluster)  [unwired: 10 in]
      n565 = property class="DAQmx Timing"(reference=w145, error in=w126) -> (reference out=w129:refnum<k21>, error out=w89:errorcluster, "Sample Clock:Rate"=w134:dbl)
      "Actual Sample Clock Rate" <- w134
      n566 = To Double Precision Float(number=u32 50000 ("Size (Samples)")) -> (double precision float=w133:dbl)
      n567 = Get Date/Time In Seconds() -> (seconds since 1Jan1904=w52:timestamp)
      n568 = Bundle By Name(cluster=cluster{"Fs":dbl, "#s":dbl} {"Fs"=1000.0, "#s"=1000.0} ("sampling info"), "#s"=w133, "Fs"=w134) -> (w143:cluster{"Fs":dbl, "#s":dbl})
      n569 = call "timestamp_conversion.vi"("Time Stamp"=w52) -> ("Integer Time"=w51:i64)  [unwired: 8 in, 1 out]
      n570 = while {
        tunnel: w143 -> [w1331]
        tunnel: w134 -> [w1329]
        tunnel: w133 -> [w1316]
        shift-right: [w1328] -> w132
        shift-left: w129 -> [w1326]
        shift-right: [w1324] -> w128
        shift-left: w89 -> [w1333]
        shift-right: [w1278] -> _
        shift-left: w53 -> [w1285]
        shift-right: [w1277] -> _
        shift-left: w53 -> [w1284]
        shift-right: [w1276] -> _
        shift-left: w53 -> [w1283]
        shift-right: [w1275] -> _
        shift-left: w53 -> [w1282]
        shift-right: [w1274] -> _
        shift-left: w53 -> [w1281]
        shift-right: [w1273] -> _
        shift-left: w53 -> [w1280]
        shift-right: [w1272] -> _
        shift-left: w53 -> [w1279]
        shift-right: [w1268] -> _
        shift-left: w51 -> [w1269]
        i -> [w1332]
        stop <- w1325 stop-if-true
        w1310 = 0.0 ("t")
        w1318 = T2 {"Integer Timestamp"=0, "Einzel Voltage"=0.05, "Needle Voltage"=1.0, "Frequency"=0.0, "Width (ms) : 0.1 "=0.0, "Desired Amplitude (V)"=0.0, "X Voltage"=0.0, "Y Voltage"=0.0, "Settings ID"="", "ID#"=0}  # Dust Source Controls
        w1319 = 1
        w1323 = T7 0 items=["no dialog", "OK message", "continue or stop message", "OK message + warnings", "continue/stop + warnings"] ("type of dialog (OK msg:1)")
        w1322 = FALSE ("Blinking")
        # "On criteria - 0: Needle Voltage, 1: Desired Amplitude, 2: Width, 3: Frequency"
        # "Event structure to ramp up or ramp down (depending on what you want) pelletron controls"
        # "Throttling stuff"
        # "Output loop"
        n571 = property on="Actual Needle Output (V)" class="DigNum (strict)"("Blinking"=w1322) -> ()  [unwired: 2 in, 2 out]
        n572 = property on="Actual Y Output (V)" class="DigNum (strict)"("Blinking"=w1322) -> ()  [unwired: 2 in, 2 out]
        n573 = property on="Actual X Output (V)" class="DigNum (strict)"("Blinking"=w1322) -> ()  [unwired: 2 in, 2 out]
        n574 = property on="Actual output Amplitude (V)" class="DigNum (strict)"("Blinking"=w1322) -> ()  [unwired: 2 in, 2 out]
        n575 = property on="Actual Einzel Output (V)" class="DigNum (strict)"("Blinking"=w1322) -> ()  [unwired: 2 in, 2 out]
        n576 = Reciprocal(x=w1329) -> (1/x=w1330:dbl)
        n577 = global read "throttle.vi" "Throttle"() -> (w1286:bool)
        n578 = call-poly <userlib>:"Data Changed__ogtk.vi"("Boolean"=w1286) -> ("Changed"=w1288:bool)
        n579 = case shown="False" w1288 {
          tunnel: w1286 -> [_ w1335]
          tunnel: "Frequency" -> [_ w1334]
          frame False {
          }
          frame True {
            n580 = case shown="True" w1335 {
              tunnel: w1334 -> [_ w1336]
              frame False {
              }
              frame True {
                "Freq. Before Throttle" <- w1336
              }
            }
          }
        }
        n581 = event shown="[1] \"X Voltage\", \"Y Voltage\": Value Change" {
          selector: _ -> [_ _]
          dyn-events: _ -> [_ _]
          timeout: 1 -> [_ _]
          tunnel: [w1411 w1412] -> w1309
          event Timeout {
            w1411 = T5 0 items=["Get", "Set X", "Set Y", "Set XY", "Internal"] ("Ring")
            n582 = event-data() -> ()  [unwired: 1 in, 2 out]
          }
          event "X Voltage", "Y Voltage": Value Change {
            w1412 = T5 4 items=["Get", "Set X", "Set Y", "Set XY", "Internal"] ("Ring")
            n583 = event-data() -> ()  [unwired: 1 in, 2 out]
          }
        }
        n584 = global read "throttle from query.vi" "Throttle Q"() -> (w1311:bool)
        n585 = Or(x=w1311, y=w1286) -> (x .or. y?=w1312:bool)
        n586 = Divide(x="Einzel Voltage", y=w1319) -> (x/y=w1320:dbl)
        n587 = call "XYVoltageFGV.vi"("X Voltage"="X Voltage", "Y Voltage"="Y Voltage", "Ring"=w1309) -> ("X Voltage 2"=w1257:dbl, "Y Voltage 2"=w1255:dbl, "Ring 2"=w1307:T5)  [unwired: 5 in]
        n588 = Bundle("Einzel Voltage"="Einzel Voltage", "X Voltage"="X Voltage", "Y Voltage"="Y Voltage") -> (→"Einzel and Steering":T1)  [unwired: 1 in]
        n589 = case shown="1" w1307 {
          tunnel: w1257 -> [_ w1417 w1421 w1424 _]
          tunnel: w1255 -> [_ w1416 w1419 w1422 _]
          tunnel: [FALSE TRUE TRUE TRUE FALSE] -> w1306
          frame 0, Default {
          }
          frame 1 {
            w1414 = T5 4 items=["Get", "Set X", "Set Y", "Set XY", "Internal"] ("Ring")
            n590 = property on="X Voltage" class="DigNum (strict)"("Val(Sgnl)"=w1417) -> ()  [unwired: 2 in, 2 out]
            n591 = call "XYVoltageFGV.vi"("X Voltage"=w1417, "Y Voltage"=w1416, "Ring"=w1414) -> ()  [unwired: 5 in, 3 out]
          }
          frame 2 {
            w1418 = T5 4 items=["Get", "Set X", "Set Y", "Set XY", "Internal"] ("Ring")
            n592 = property on="Y Voltage" class="DigNum (strict)"("Val(Sgnl)"=w1419) -> ()  [unwired: 2 in, 2 out]
            n593 = call "XYVoltageFGV.vi"("X Voltage"=w1421, "Y Voltage"=w1419, "Ring"=w1418) -> ()  [unwired: 5 in, 3 out]
          }
          frame 3 {
            w1423 = T5 2 items=["Get", "Set X", "Set Y", "Set XY", "Internal"] ("Ring")
            n594 = property on="X Voltage" class="DigNum (strict)"("Val(Sgnl)"=w1424) -> ()  [unwired: 2 in, 2 out]
            n595 = property on="Y Voltage" class="DigNum (strict)"("Value"=w1422) -> ()  [unwired: 2 in, 2 out]
            n596 = call "XYVoltageFGV.vi"("X Voltage"=w1424, "Y Voltage"=w1422, "Ring"=w1423) -> ()  [unwired: 5 in, 3 out]
          }
          frame 4 {
          }
        }
        n597 = local read "Freq. Before Throttle"() -> (w1289:dbl)
        n598 = Implies(1:w1286, 2:w1288) -> (0:w1287:bool)
        n599 = Select(t=T6."Disabled and Grayed Out" ("Disabled"), s=w1312, f=T6."Enabled" ("Disabled")) -> (s? t:f=w1313:T6)
        n600 = property on="Frequency" class="DigNum (strict)"("DisabledEnum"=w1313) -> ()  [unwired: 2 in, 2 out]
        n601 = Select(t=w1310, s=w1311, f="Frequency") -> (s? t:f=w1304:dbl)
        n602 = Select(t=w1310, s=w1286, f=w1304) -> (s? t:f=w1300:dbl)
        n603 = Select(t=w1300, s=w1287, f=w1289) -> (s? t:f=w1290:dbl)
        n604 = Divide(x="Needle Voltage", y=w1319) -> (x/y=w1321:dbl)
        n605 = call "scale xy steering.vi"("-2.5 to 2.5 V input"=w1257) -> ("0 to 9 V output"=w1256:dbl)  [unwired: 1 in, 1 out]
        n606 = call "scale xy steering.vi"("-2.5 to 2.5 V input"=w1255) -> ("0 to 9 V output"=w1254:dbl)  [unwired: 1 in, 1 out]
        n607 = call-poly <userlib>:"Data Changed__ogtk.vi"("DBL"=w1290) -> ("Changed"=w1305:bool)
        n608 = case shown="True" w1305 {
          tunnel: w1290 -> [_ w1410]
          frame False {
          }
          frame True {
            n609 = property on="Frequency" class="DigNum (strict)"("Val(Sgnl)"=w1410) -> ()  [unwired: 2 in, 2 out]
          }
        }
        n610 = Bundle By Name(cluster=w1318, "Desired Amplitude (V)"="Desired Amplitude (V)", "Width (ms) : 0.1"="Width (ms) : 0.1", "Frequency"=w1290, "Einzel Voltage"="Einzel Voltage", "X Voltage"=w1257, "Y Voltage"=w1255, "Needle Voltage"="Needle Voltage") -> (→"output cluster":T2)
        n611 = Build Array("Needle Voltage", "Desired Amplitude (V)", "Width (ms) : 0.1", w1290) -> (w1299:dbl[])
        n612 = Greater?(x=w1299, y=dbl[] [1.0, 0.0, 0.0, 0.0]) -> (0:w1297:bool[])
        n613 = And Array Elements(Boolean array=w1297) -> (logical AND=w1270:bool)
        "On/Off" <- w1270
        n614 = event shown="[4] \"Needle Voltage\": Value Change" {
          selector: _ -> [_ _ _ _ _ _ _ _ _]
          dyn-events: _ -> [_ _ _ _ _ _ _ _ _]
          timeout: 100 -> [_ _ _ _ _ _ _ _ _]
          tunnel: w1331 -> [w1440 w1502 w1629 w1751 w1870 w1958 w2079 w2192 w2307]
          tunnel: w1333 -> [w1464 w1494 w1644 w1766 w1865 w1957 w2055 w2168 w2283]
          tunnel: w1290 -> [w1435 w1517 w1645 w1767 w1888 w1936 w2035 w2194 w2265]
          tunnel: "Width (ms) : 0.1" -> [w1436 w1518 w1646 w1768 w1889 w1935 w2037 w2149 w2309]
          tunnel: [w1463 w1492 w1647 w1769 w1864 w1948 w2053 w2166 w2281] -> w1296
          tunnel: w1326 -> [w1462 w1516 w1643 w1765 w1887 w1952 w2080 w2193 w2308]
          tunnel: "Desired Amplitude (V)" -> [w1438 w1491 w1618 w1740 w1862 w1942 w2036 w2150 w2264]
          tunnel: w1316 -> [w1444 w1506 w1634 w1756 w1878 w1954 w2067 w2180 w2295]
          tunnel: w1330 -> [w1443 w1505 w1633 w1755 w1877 w1955 w2066 w2179 w2294]
          tunnel: w1320 -> [w1455 w1474 w1640 w1762 w1884 w1937 w2076 w2189 w2304]
          tunnel: [w1454 w1515 w1642 w1764 w1886 w1953 w2075 w2188 w2303] -> w1328
          tunnel: w1256 -> [w1447 w1512 _ w1758 w1880 _ w2073 w2186 w2301]
          tunnel: w1254 -> [w1448 w1509 w1636 _ w1874 _ w2071 w2184 w2299]
          tunnel: [FALSE ("y") FALSE ("y") FALSE ("y") FALSE ("y") FALSE ("y") TRUE ("y") FALSE ("y") FALSE ("y") FALSE ("y")] -> w1293
          tunnel: w1321 -> [w1442 w1504 w1631 w1753 _ w1941 w2063 w2176 w2291]
          tunnel: w1306 -> [_ _ w1619 w1741 _ _ _ _ _]
          tunnel: w1285 -> [w1434 w1485 w1617 w1738 w1860 _ w2051 w2164 w2279]
          tunnel: w1284 -> [w1433 w1484 w1615 w1737 w1861 _ w2050 w2163 w2278]
          tunnel: w1283 -> [w1432 w1490 w1614 w1736 w1859 _ w2052 w2162 w2277]
          tunnel: w1282 -> [w1431 w1489 w1613 w1735 w1858 _ w2049 w2161 w2280]
          tunnel: w1281 -> [w1430 w1488 w1612 w1734 w1857 _ w2048 w2165 w2276]
          tunnel: w1280 -> [w1429 w1487 w1616 w1733 w1856 _ w2047 w2160 w2275]
          tunnel: w1279 -> [w1428 w1486 w1611 w1739 w1855 _ w2046 w2159 w2274]
          tunnel: [w1434 w1476 w1617 w1738 w1860 w1943 w2051 w2164 w2279] -> w1278
          tunnel: [w1433 w1484 w1615 w1737 w1849 w1943 w2050 w2163 w2278] -> w1277
          tunnel: [w1432 w1490 w1614 w1736 w1859 w1943 w2040 w2162 w2277] -> w1276
          tunnel: [w1431 w1489 w1613 w1735 w1858 w1943 w2049 w2161 w2268] -> w1275
          tunnel: [w1430 w1488 w1612 w1734 w1857 w1943 w2048 w2151 w2276] -> w1274
          tunnel: [w1429 w1487 w1605 w1733 w1856 w1943 w2047 w2160 w2275] -> w1273
          tunnel: [w1428 w1486 w1611 w1727 w1855 w1943 w2046 w2159 w2274] -> w1272
          event Timeout {
            w1437 = FALSE ("Blinking")
            n615 = event-data() -> ()  [unwired: 1 in, 2 out]
            n616 = local write "Actual X Output (V)"(w1447) -> ()
            n617 = local write "Actual Y Output (V)"(w1448) -> ()
            n618 = local write "Actual Needle Output (V)"(w1442) -> ()
            n619 = local write "Actual Einzel Output (V)"(w1455) -> ()
            n620 = local write "Actual output Amplitude (V)"(w1438) -> ()
            n621 = call "Gen_Square_0to10V.vi"("sampling info"=w1440, "error in (no error)"=w1464, "Width (ms)"=w1436, "amplitude"=w1438, "frequency"=w1435) -> ("error out"=w1459:errorcluster, "signal out"=w1439:waveform(dbl))  [unwired: 5 in]
            n622 = Initialize Array(w1447, w1444) -> (w1452:dbl[])
            n623 = Initialize Array(w1448, w1444) -> (w1450:dbl[])
            n624 = Initialize Array(w1442, w1444) -> (w1445:dbl[])
            n625 = Initialize Array(w1455, w1444) -> (w1456:dbl[])
            n626 = local write "Actual output width (ms)"(w1436) -> ()
            n627 = local write "Actual output Frequency"(w1435) -> ()
            n628 = local write "Output waveform"(w1439) -> ()
            n629 = Bundle By Name("Y"=w1452, "dt"=w1443) -> (w1451:waveform(dbl))  [unwired: 1 in]
            n630 = Bundle By Name("Y"=w1450, "dt"=w1443) -> (w1449:waveform(dbl))  [unwired: 1 in]
            n631 = Bundle By Name("Y"=w1445, "dt"=w1443) -> (w1441:waveform(dbl))  [unwired: 1 in]
            n632 = Bundle By Name("Y"=w1456, "dt"=w1443) -> (w1453:waveform(dbl))  [unwired: 1 in]
            n633 = Merge Signals(w1439, w1453, w1451, w1449, w1441) -> (w1457:dynamicdata)
            n634 = local read "Tab Control"() -> (w1427:T3)
            n635 = call-poly <vilib>:"DAQmx Write.vi"("task/channels in"=w1462, "data"=w1457, "error in"=w1459) -> ("task out"=w1461:refnum<k21>, "error out"=w1458:errorcluster)  [unwired: 10 in, 1 out]
            n636 = case shown="\"EXY Scan Data\"" w1427 {
              frame "Controls", Default {
              }
              frame "EXY Scan Data" {
              }
              frame "Status" {
                n637 = Unbundle By Name("Maximums") -> ("Width"=w1466:dbl, "Freq."=w1465:dbl)
                n638 = property on="Frequency" class="DigNum (strict)"("Maximum"=w1465) -> ()  [unwired: 2 in, 2 out]
                n639 = property on="Width (ms) : 0.1" class="DigNum (strict)"("Maximum"=w1466) -> ()  [unwired: 2 in, 2 out]
              }
            }
            n640 = First Call?() -> (First Call?: T/F=w1460:bool)
            n641 = case shown="True" w1460 {
              tunnel: [w1468 w1473] -> w1463
              tunnel: [w1469 w1472] -> w1454
              tunnel: w1461 -> [w1469 w1471]
              tunnel: w1458 -> [w1468 w1470]
              frame False {
              }
              frame True {
                n642 = call <vilib>:"DAQmx Start Task.vi"("task/channels in"=w1471, "error in"=w1470) -> ("task out"=w1472:refnum<k21>, "error out"=w1473:errorcluster)  [unwired: 12 in]
              }
            }
            n643 = property on="Actual output Amplitude (V)" class="DigNum (strict)"("Blinking"=w1437) -> ()  [unwired: 2 in, 2 out]
            n644 = property on="Actual X Output (V)" class="DigNum (strict)"("Blinking"=w1437) -> ()  [unwired: 2 in, 2 out]
            n645 = property on="Actual Needle Output (V)" class="DigNum (strict)"("Blinking"=w1437) -> ()  [unwired: 2 in, 2 out]
            n646 = property on="Actual Einzel Output (V)" class="DigNum (strict)"("Blinking"=w1437) -> ()  [unwired: 2 in, 2 out]
            n647 = property on="Actual Y Output (V)" class="DigNum (strict)"("Blinking"=w1437) -> ()  [unwired: 2 in, 2 out]
            n648 = property on="Actual output width (ms)" class="DigNum (strict)"("Blinking"=w1437) -> ()  [unwired: 2 in, 2 out]
            n649 = property on="Actual output Frequency" class="DigNum (strict)"("Blinking"=w1437) -> ()  [unwired: 2 in, 2 out]
          }
          event "Einzel Voltage": Value Change {
            w1500 = 0.05 ("y")
            n650 = event-data() -> ("NewVal"=w1477:dbl)  [unwired: 1 in, 4 out]
            n651 = local write "Actual X Output (V)"(w1512) -> ()
            n652 = local write "Actual Y Output (V)"(w1509) -> ()
            n653 = local write "Actual Needle Output (V)"(w1504) -> ()
            n654 = Greater?(x=w1477, y=w1485) -> (0:w1501:bool)
            n655 = Subtract(x=w1485, y=w1477) -> (x-y=w1496:dbl)
            n656 = Subtract(x=w1477, y=w1485) -> (x-y=w1498:dbl)
            n657 = Initialize Array(w1512, w1506) -> (w1514:dbl[])
            n658 = Initialize Array(w1509, w1506) -> (w1511:dbl[])
            n659 = Initialize Array(w1504, w1506) -> (w1507:dbl[])
            n660 = Greater?(x=w1496, y=w1498) -> (0:w1499:bool)
            n661 = Bundle By Name("Y"=w1514, "dt"=w1505) -> (w1513:waveform(dbl))  [unwired: 1 in]
            n662 = Bundle By Name("Y"=w1511, "dt"=w1505) -> (w1510:waveform(dbl))  [unwired: 1 in]
            n663 = Bundle By Name("Y"=w1507, "dt"=w1505) -> (w1503:waveform(dbl))  [unwired: 1 in]
            n664 = Select(t=w1496, s=w1499, f=w1498) -> (s? t:f=w1495:dbl)
            n665 = local read "Calibrate XY"() -> (w1475:bool)
            n666 = Divide(x=w1495, y=w1500) -> (x/y=w1497:dbl)
            n667 = To Long Integer(number=w1497) -> (32bit integer=w1478:i32)
            n668 = case shown="False" w1475 {
              tunnel: w1518 -> [w1537 w1601]
              tunnel: w1517 -> [w1536 w1600]
              tunnel: w1516 -> [w1535 w1599]
              tunnel: [w1534 w1598] -> w1515
              tunnel: w1513 -> [w1533 w1597]
              tunnel: w1510 -> [w1532 w1596]
              tunnel: w1506 -> [w1531 w1595]
              tunnel: w1505 -> [w1530 w1594]
              tunnel: w1503 -> [w1529 w1593]
              tunnel: w1502 -> [w1528 w1592]
              tunnel: w1501 -> [w1527 _]
              tunnel: w1500 -> [w1526 _]
              tunnel: w1494 -> [w1525 w1591]
              tunnel: [w1524 w1590] -> w1493
              tunnel: w1491 -> [w1523 w1589]
              tunnel: w1485 -> [w1522 _]
              tunnel: [w1521 w1580] -> w1480
              tunnel: [w1520 w1588] -> w1479
              tunnel: w1478 -> [w1519 _]
              tunnel: w1474 -> [_ w1580]
              frame False {
                n669 = for {
                  N: w1519 -> [_]
                  tunnel: w1526 -> [w1572]
                  tunnel: w1522 -> [w1571]
                  tunnel: w1530 -> [w1570]
                  tunnel: w1531 -> [w1569]
                  tunnel: [w1568] -> w1524
                  tunnel: w1537 -> [w1561]
                  tunnel: w1523 -> [w1549]
                  tunnel: w1536 -> [w1564]
                  tunnel: w1525 -> [w1563]
                  tunnel: w1533 -> [w1559]
                  tunnel: w1532 -> [w1558]
                  tunnel: w1529 -> [w1556]
                  shift-right: [w1567] -> w1534
                  shift-left: w1535 -> [w1562]
                  tunnel: w1528 -> [w1555]
                  tunnel: w1527 -> [w1551]
                  tunnel: [w1546] -> w1521
                  tunnel: [w1544] -> w1520
                  i -> [w1573]
                  stop <- w1544 stop-if-true
                  n670 = local write "Actual output Amplitude (V)"(w1549) -> ()
                  n671 = call "Gen_Square_0to10V.vi"("sampling info"=w1555, "error in (no error)"=w1563, "Width (ms)"=w1561, "amplitude"=w1549, "frequency"=w1564) -> ("error out"=w1565:errorcluster, "signal out"=w1550:waveform(dbl))  [unwired: 5 in]
                  n672 = Increment(x=w1573) -> (x+1=w1574:i32)
                  n673 = property on="Actual Einzel Output (V)" class="DigNum (strict)"("Blinking"=TRUE) -> ()  [unwired: 2 in, 2 out]
                  n674 = local write "Output waveform"(w1550) -> ()
                  n675 = Multiply(x=w1572, y=w1574) -> (x*y=w1553:dbl)
                  n676 = Negate(x=w1553) -> (-x=w1552:dbl)
                  n677 = Select(t=w1553, s=w1551, f=w1552) -> (s? t:f=w1554:dbl)
                  n678 = Add(x=w1571, y=w1554) -> (x+y=w1542:dbl)
                  n679 = Less Than 0?(x=w1542) -> (x < 0?=w1548:bool)
                  n680 = Select(t=0.0, s=w1548, f=w1542) -> (s? t:f=w1546:dbl)
                  n681 = local write "Actual Einzel Output (V)"(w1546) -> ()
                  n682 = Initialize Array(w1546, w1569) -> (w1539:dbl[])
                  n683 = In Range and Coerce(upper limit=10.0, x=w1539, lower limit=0.0) -> (coerced(x)=w1538:dbl[])  [unwired: 1 out]
                  n684 = Bundle By Name("Y"=w1538, "dt"=w1570) -> (w1560:waveform(dbl))  [unwired: 1 in]
                  n685 = local read "Abort Change"() -> (w1545:bool)
                  n686 = local read "stop"() -> (w1543:bool)
                  n687 = Or(x=w1543, y=w1545) -> (x .or. y?=w1544:bool)
                  n688 = Merge Signals(w1550, w1560, w1559, w1558, w1556) -> (w1566:dynamicdata)
                  n689 = case shown="True" w1544 {
                    tunnel: w1546 -> [_ w1575]
                    frame False {
                    }
                    frame True {
                      n690 = local write "Einzel Voltage"(w1575) -> ()
                    }
                  }
                  n691 = call-poly <vilib>:"DAQmx Write.vi"("task/channels in"=w1562, "data"=w1566, "error in"=w1565) -> ("task out"=w1567:refnum<k21>, "error out"=w1568:errorcluster)  [unwired: 10 in, 1 out]
                }
              }
              frame True {
                n692 = local write "Actual output Amplitude (V)"(w1589) -> ()
                n693 = call "Gen_Square_0to10V.vi"("sampling info"=w1592, "error in (no error)"=w1591, "Width (ms)"=w1601, "amplitude"=w1589, "frequency"=w1600) -> ("error out"=w1586:errorcluster, "signal out"=w1583:waveform(dbl))  [unwired: 5 in]
                n694 = property on="Actual Einzel Output (V)" class="DigNum (strict)"("Blinking"=TRUE) -> ()  [unwired: 2 in, 2 out]
                n695 = local write "Output waveform"(w1583) -> ()
                n696 = local write "Actual Einzel Output (V)"(w1580) -> ()
                n697 = Initialize Array(w1580, w1595) -> (w1577:dbl[])
                n698 = In Range and Coerce(upper limit=10.0, x=w1577, lower limit=0.0) -> (coerced(x)=w1576:dbl[])  [unwired: 1 out]
                n699 = Bundle By Name("Y"=w1576, "dt"=w1594) -> (w1585:waveform(dbl))  [unwired: 1 in]
                n700 = local read "Abort Change"() -> (w1582:bool)
                n701 = local read "stop"() -> (w1581:bool)
                n702 = Or(x=w1581, y=w1582) -> (x .or. y?=w1588:bool)
                n703 = Merge Signals(w1583, w1585, w1597, w1596, w1593) -> (w1587:dynamicdata)
                n704 = case shown="True" w1588 {
                  tunnel: w1580 -> [_ w1602]
                  frame False {
                  }
                  frame True {
                    n705 = local write "Einzel Voltage"(w1602) -> ()
                  }
                }
                n706 = call-poly <vilib>:"DAQmx Write.vi"("task/channels in"=w1599, "data"=w1587, "error in"=w1586) -> ("task out"=w1598:refnum<k21>, "error out"=w1590:errorcluster)  [unwired: 10 in, 1 out]
              }
            }
            n707 = Equal To 0?(x=w1478) -> (x = 0?=w1482:bool)
            n708 = Not(x=w1479) -> (.not. x?=w1483:bool)
            n709 = Merge Errors(w1493) -> (w1492:errorcluster)
            n710 = Or(x=w1483, y=w1482) -> (x .or. y?=w1481:bool)
            n711 = Select(t=w1477, s=w1481, f=w1480) -> (s? t:f=w1476:dbl)
          }
          event "X Voltage": Value Change {
            w1626 = 0.05 ("y")
            n712 = event-data() -> ("NewVal"=w1604:dbl)  [unwired: 1 in, 4 out]
            n713 = local write "Actual Y Output (V)"(w1636) -> ()
            n714 = local write "Actual Needle Output (V)"(w1631) -> ()
            n715 = local write "Actual Einzel Output (V)"(w1640) -> ()
            n716 = Greater?(x=w1604, y=w1616) -> (0:w1628:bool)
            n717 = Subtract(x=w1604, y=w1616) -> (x-y=w1622:dbl)
            n718 = Subtract(x=w1616, y=w1604) -> (x-y=w1625:dbl)
            n719 = Initialize Array(w1636, w1634) -> (w1638:dbl[])
            n720 = Initialize Array(w1631, w1634) -> (w1632:dbl[])
            n721 = Initialize Array(w1640, w1634) -> (w1641:dbl[])
            n722 = Greater?(x=w1622, y=w1625) -> (0:w1627:bool)
            n723 = Bundle By Name("Y"=w1638, "dt"=w1633) -> (w1637:waveform(dbl))  [unwired: 1 in]
            n724 = Bundle By Name("Y"=w1632, "dt"=w1633) -> (w1630:waveform(dbl))  [unwired: 1 in]
            n725 = Bundle By Name("Y"=w1641, "dt"=w1633) -> (w1639:waveform(dbl))  [unwired: 1 in]
            n726 = Select(t=w1622, s=w1627, f=w1625) -> (s? t:f=w1623:dbl)
            n727 = Divide(x=w1623, y=w1626) -> (x/y=w1624:dbl)
            n728 = local read "Calibrate XY"() -> (w1621:bool)
            n729 = To Long Integer(number=w1624) -> (32bit integer=w1603:i32)
            n730 = Or(x=w1621, y=w1619) -> (x .or. y?=w1620:bool)
            n731 = case shown="True" w1620 {
              tunnel: [w1666 w1711] -> w1647
              tunnel: w1646 -> [w1665 w1724]
              tunnel: w1618 -> [w1664 w1723]
              tunnel: w1645 -> [w1663 w1722]
              tunnel: w1644 -> [w1662 w1721]
              tunnel: w1643 -> [w1661 w1720]
              tunnel: [w1660 w1712] -> w1642
              tunnel: w1639 -> [w1659 w1719]
              tunnel: w1637 -> [w1658 w1718]
              tunnel: w1634 -> [w1657 w1717]
              tunnel: w1633 -> [w1656 w1716]
              tunnel: w1630 -> [w1655 w1715]
              tunnel: w1629 -> [w1654 w1714]
              tunnel: w1628 -> [w1653 _]
              tunnel: w1626 -> [w1652 _]
              tunnel: w1603 -> [w1651 _]
              tunnel: w1616 -> [w1650 _]
              tunnel: w1604 -> [_ w1704]
              tunnel: [w1649 w1703] -> w1606
              tunnel: [w1648 FALSE ("Abort Change")] -> w1607
              frame False {
                n732 = for {
                  N: w1651 -> [_]
                  tunnel: w1652 -> [w1696]
                  tunnel: w1650 -> [w1695]
                  tunnel: w1656 -> [w1694]
                  tunnel: w1657 -> [w1693]
                  tunnel: [w1692] -> w1666
                  tunnel: w1665 -> [w1674]
                  tunnel: w1664 -> [w1673]
                  tunnel: w1663 -> [w1688]
                  tunnel: w1662 -> [w1687]
                  tunnel: w1659 -> [w1684]
                  tunnel: w1658 -> [w1682]
                  tunnel: w1655 -> [w1681]
                  shift-right: [w1691] -> w1660
                  shift-left: w1661 -> [w1686]
                  tunnel: w1654 -> [w1680]
                  tunnel: w1653 -> [w1676]
                  tunnel: [w1668] -> w1649
                  tunnel: [w1672] -> w1648
                  i -> [w1697]
                  stop <- w1672 stop-if-true
                  n733 = local write "Actual output Amplitude (V)"(w1673) -> ()
                  n734 = call "Gen_Square_0to10V.vi"("sampling info"=w1680, "error in (no error)"=w1687, "Width (ms)"=w1674, "amplitude"=w1673, "frequency"=w1688) -> ("error out"=w1689:errorcluster, "signal out"=w1675:waveform(dbl))  [unwired: 5 in]
                  n735 = Increment(x=w1697) -> (x+1=w1698:i32)
                  n736 = property on="Actual X Output (V)" class="DigNum (strict)"("Blinking"=TRUE) -> ()  [unwired: 2 in, 2 out]
                  n737 = local write "Output waveform"(w1675) -> ()
                  n738 = Multiply(x=w1696, y=w1698) -> (x*y=w1678:dbl)
                  n739 = Negate(x=w1678) -> (-x=w1679:dbl)
                  n740 = Select(t=w1678, s=w1676, f=w1679) -> (s? t:f=w1677:dbl)
                  n741 = Add(x=w1695, y=w1677) -> (x+y=w1668:dbl)
                  n742 = call "scale xy steering.vi"("-2.5 to 2.5 V input"=w1668) -> ("0 to 9 V output"=w1667:dbl)  [unwired: 1 in, 1 out]
                  n743 = local write "Actual X Output (V)"(w1667) -> ()
                  n744 = Initialize Array(w1667, w1693) -> (w1669:dbl[])
                  n745 = Bundle By Name("Y"=w1669, "dt"=w1694) -> (w1683:waveform(dbl))  [unwired: 1 in]
                  n746 = local read "Abort Change"() -> (w1671:bool)
                  n747 = Merge Signals(w1675, w1684, w1683, w1682, w1681) -> (w1690:dynamicdata)
                  n748 = local read "stop"() -> (w1670:bool)
                  n749 = Or(x=w1670, y=w1671) -> (x .or. y?=w1672:bool)
                  n750 = call-poly <vilib>:"DAQmx Write.vi"("task/channels in"=w1686, "data"=w1690, "error in"=w1689) -> ("task out"=w1691:refnum<k21>, "error out"=w1692:errorcluster)  [unwired: 10 in, 1 out]
                  n751 = case shown="True" w1672 {
                    tunnel: w1668 -> [_ w1700]
                    frame False {
                    }
                    frame True {
                      w1699 = T5 4 items=["Get", "Set X", "Set Y", "Set XY", "Internal"] ("Ring")
                      w1702 = T5 0 items=["Get", "Set X", "Set Y", "Set XY", "Internal"] ("Ring")
                      n752 = local write "X Voltage"(w1700) -> ()
                      n753 = call "XYVoltageFGV.vi"("Ring"=w1702) -> ("Y Voltage 2"=w1701:dbl)  [unwired: 7 in, 2 out]
                      n754 = call "XYVoltageFGV.vi"("X Voltage"=w1700, "Y Voltage"=w1701, "Ring"=w1699) -> ()  [unwired: 5 in, 3 out]
                    }
                  }
                }
              }
              frame True {
                n755 = local write "Actual output Amplitude (V)"(w1723) -> ()
                n756 = call "Gen_Square_0to10V.vi"("sampling info"=w1714, "error in (no error)"=w1721, "Width (ms)"=w1724, "amplitude"=w1723, "frequency"=w1722) -> ("error out"=w1709:errorcluster, "signal out"=w1706:waveform(dbl))  [unwired: 5 in]
                n757 = property on="Actual X Output (V)" class="DigNum (strict)"("Blinking"=TRUE) -> ()  [unwired: 2 in, 2 out]
                n758 = local write "Output waveform"(w1706) -> ()
                n759 = call "scale xy steering.vi"("-2.5 to 2.5 V input"=w1704) -> ("0 to 9 V output"=w1703:dbl)  [unwired: 1 in, 1 out]
                n760 = local write "Actual X Output (V)"(w1703) -> ()
                n761 = Initialize Array(w1703, w1717) -> (w1713:dbl[])
                n762 = Bundle By Name("Y"=w1713, "dt"=w1716) -> (w1707:waveform(dbl))  [unwired: 1 in]
                n763 = Merge Signals(w1706, w1719, w1707, w1718, w1715) -> (w1710:dynamicdata)
                n764 = call-poly <vilib>:"DAQmx Write.vi"("task/channels in"=w1720, "data"=w1710, "error in"=w1709) -> ("task out"=w1712:refnum<k21>, "error out"=w1711:errorcluster)  [unwired: 10 in, 1 out]
              }
            }
            n765 = Equal To 0?(x=w1603) -> (x = 0?=w1609:bool)
            n766 = Not(x=w1607) -> (.not. x?=w1610:bool)
            n767 = Or(x=w1610, y=w1609) -> (x .or. y?=w1608:bool)
            n768 = Select(t=w1604, s=w1608, f=w1606) -> (s? t:f=w1605:dbl)
          }
          event "Y Voltage": Value Change {
            w1748 = 0.05 ("y")
            n769 = event-data() -> ("NewVal"=w1726:dbl)  [unwired: 1 in, 4 out]
            n770 = local write "Actual X Output (V)"(w1758) -> ()
            n771 = local write "Actual Needle Output (V)"(w1753) -> ()
            n772 = local write "Actual Einzel Output (V)"(w1762) -> ()
            n773 = Greater?(x=w1726, y=w1739) -> (0:w1750:bool)
            n774 = Subtract(x=w1726, y=w1739) -> (x-y=w1746:dbl)
            n775 = Subtract(x=w1739, y=w1726) -> (x-y=w1747:dbl)
            n776 = Initialize Array(w1758, w1756) -> (w1760:dbl[])
            n777 = Initialize Array(w1753, w1756) -> (w1754:dbl[])
            n778 = Initialize Array(w1762, w1756) -> (w1763:dbl[])
            n779 = Greater?(x=w1746, y=w1747) -> (0:w1749:bool)
            n780 = Bundle By Name("Y"=w1760, "dt"=w1755) -> (w1759:waveform(dbl))  [unwired: 1 in]
            n781 = Bundle By Name("Y"=w1754, "dt"=w1755) -> (w1752:waveform(dbl))  [unwired: 1 in]
            n782 = Bundle By Name("Y"=w1763, "dt"=w1755) -> (w1761:waveform(dbl))  [unwired: 1 in]
            n783 = Select(t=w1746, s=w1749, f=w1747) -> (s? t:f=w1745:dbl)
            n784 = local read "Calibrate XY"() -> (w1743:bool)
            n785 = Divide(x=w1745, y=w1748) -> (x/y=w1744:dbl)
            n786 = To Long Integer(number=w1744) -> (32bit integer=w1725:i32)
            n787 = Or(x=w1743, y=w1741) -> (x .or. y?=w1742:bool)
            n788 = case shown="False" w1742 {
              tunnel: [w1788 w1833] -> w1769
              tunnel: w1768 -> [w1787 w1846]
              tunnel: w1740 -> [w1786 w1845]
              tunnel: w1767 -> [w1785 w1844]
              tunnel: w1766 -> [w1784 w1843]
              tunnel: w1765 -> [w1783 w1842]
              tunnel: [w1782 w1834] -> w1764
              tunnel: w1761 -> [w1781 w1841]
              tunnel: w1759 -> [w1780 w1840]
              tunnel: w1756 -> [w1779 w1839]
              tunnel: w1755 -> [w1778 w1838]
              tunnel: w1752 -> [w1777 w1837]
              tunnel: w1751 -> [w1776 w1836]
              tunnel: w1750 -> [w1775 _]
              tunnel: w1748 -> [w1774 _]
              tunnel: w1725 -> [w1773 _]
              tunnel: w1739 -> [w1772 _]
              tunnel: w1726 -> [_ w1825]
              tunnel: [w1771 w1826] -> w1728
              tunnel: [w1770 FALSE ("Abort Change")] -> w1729
              frame False {
                n789 = for {
                  N: w1773 -> [_]
                  tunnel: w1774 -> [w1818]
                  tunnel: w1772 -> [w1817]
                  tunnel: w1778 -> [w1815]
                  tunnel: w1779 -> [w1814]
                  tunnel: [w1813] -> w1788
                  tunnel: w1787 -> [w1794]
                  tunnel: w1786 -> [w1795]
                  tunnel: w1785 -> [w1809]
                  tunnel: w1784 -> [w1808]
                  tunnel: w1781 -> [w1797]
                  tunnel: w1780 -> [w1805]
                  tunnel: w1777 -> [w1803]
                  shift-right: [w1812] -> w1782
                  shift-left: w1783 -> [w1807]
                  tunnel: w1775 -> [w1799]
                  tunnel: w1776 -> [w1798]
                  tunnel: [w1790] -> w1771
                  tunnel: [w1792] -> w1770
                  i -> [w1819]
                  stop <- w1792 stop-if-true
                  n790 = local write "Actual output Amplitude (V)"(w1795) -> ()
                  n791 = call "Gen_Square_0to10V.vi"("sampling info"=w1798, "error in (no error)"=w1808, "Width (ms)"=w1794, "amplitude"=w1795, "frequency"=w1809) -> ("error out"=w1810:errorcluster, "signal out"=w1796:waveform(dbl))  [unwired: 5 in]
                  n792 = Increment(x=w1819) -> (x+1=w1820:i32)
                  n793 = property on="Actual Y Output (V)" class="DigNum (strict)"("Blinking"=TRUE) -> ()  [unwired: 2 in, 2 out]
                  n794 = local write "Output waveform"(w1796) -> ()
                  n795 = Multiply(x=w1818, y=w1820) -> (x*y=w1801:dbl)
                  n796 = Negate(x=w1801) -> (-x=w1802:dbl)
                  n797 = Select(t=w1801, s=w1799, f=w1802) -> (s? t:f=w1800:dbl)
                  n798 = Add(x=w1817, y=w1800) -> (x+y=w1790:dbl)
                  n799 = call "scale xy steering.vi"("-2.5 to 2.5 V input"=w1790) -> ("0 to 9 V output"=w1789:dbl)  [unwired: 1 in, 1 out]
                  n800 = local write "Actual Y Output (V)"(w1789) -> ()
                  n801 = Initialize Array(w1789, w1814) -> (w1816:dbl[])
                  n802 = Bundle By Name("Y"=w1816, "dt"=w1815) -> (w1804:waveform(dbl))  [unwired: 1 in]
                  n803 = Merge Signals(w1796, w1797, w1805, w1804, w1803) -> (w1811:dynamicdata)
                  n804 = local read "Abort Change"() -> (w1793:bool)
                  n805 = local read "stop"() -> (w1791:bool)
                  n806 = call-poly <vilib>:"DAQmx Write.vi"("task/channels in"=w1807, "data"=w1811, "error in"=w1810) -> ("task out"=w1812:refnum<k21>, "error out"=w1813:errorcluster)  [unwired: 10 in, 1 out]
                  n807 = Or(x=w1793, y=w1791) -> (x .or. y?=w1792:bool)
                  n808 = case shown="True" w1792 {
                    tunnel: w1790 -> [_ w1822]
                    frame False {
                    }
                    frame True {
                      w1821 = T5 4 items=["Get", "Set X", "Set Y", "Set XY", "Internal"] ("Ring")
                      w1824 = T5 0 items=["Get", "Set X", "Set Y", "Set XY", "Internal"] ("Ring")
                      n809 = local write "Y Voltage"(w1822) -> ()
                      n810 = call "XYVoltageFGV.vi"("Ring"=w1824) -> ("X Voltage 2"=w1823:dbl)  [unwired: 7 in, 2 out]
                      n811 = call "XYVoltageFGV.vi"("X Voltage"=w1823, "Y Voltage"=w1822, "Ring"=w1821) -> ()  [unwired: 5 in, 3 out]
                    }
                  }
                }
              }
              frame True {
                n812 = local write "Actual output Amplitude (V)"(w1845) -> ()
                n813 = call "Gen_Square_0to10V.vi"("sampling info"=w1836, "error in (no error)"=w1843, "Width (ms)"=w1846, "amplitude"=w1845, "frequency"=w1844) -> ("error out"=w1831:errorcluster, "signal out"=w1828:waveform(dbl))  [unwired: 5 in]
                n814 = property on="Actual Y Output (V)" class="DigNum (strict)"("Blinking"=TRUE) -> ()  [unwired: 2 in, 2 out]
                n815 = local write "Output waveform"(w1828) -> ()
                n816 = call "scale xy steering.vi"("-2.5 to 2.5 V input"=w1825) -> ("0 to 9 V output"=w1826:dbl)  [unwired: 1 in, 1 out]
                n817 = local write "Actual Y Output (V)"(w1826) -> ()
                n818 = Initialize Array(w1826, w1839) -> (w1835:dbl[])
                n819 = Bundle By Name("Y"=w1835, "dt"=w1838) -> (w1829:waveform(dbl))  [unwired: 1 in]
                n820 = Merge Signals(w1828, w1841, w1840, w1829, w1837) -> (w1832:dynamicdata)
                n821 = call-poly <vilib>:"DAQmx Write.vi"("task/channels in"=w1842, "data"=w1832, "error in"=w1831) -> ("task out"=w1834:refnum<k21>, "error out"=w1833:errorcluster)  [unwired: 10 in, 1 out]
              }
            }
            n822 = Equal To 0?(x=w1725) -> (x = 0?=w1731:bool)
            n823 = Not(x=w1729) -> (.not. x?=w1732:bool)
            n824 = Or(x=w1732, y=w1731) -> (x .or. y?=w1730:bool)
            n825 = Select(t=w1726, s=w1730, f=w1728) -> (s? t:f=w1727:dbl)
          }
          event "Needle Voltage": Value Change {
            (unwired) "needle" ("name (unnamed)")
            w1871 = 0.05 ("y")
            n826 = event-data() -> ("NewVal"=w1848:dbl)  [unwired: 1 in, 4 out]
            n827 = local write "Actual X Output (V)"(w1880) -> ()
            n828 = local write "Actual Y Output (V)"(w1874) -> ()
            n829 = local write "Actual Einzel Output (V)"(w1884) -> ()
            n830 = Greater?(x=w1848, y=w1861) -> (0:w1873:bool)
            n831 = Subtract(x=w1848, y=w1861) -> (x-y=w1867:dbl)
            n832 = Subtract(x=w1861, y=w1848) -> (x-y=w1868:dbl)
            n833 = Initialize Array(w1880, w1878) -> (w1882:dbl[])
            n834 = Initialize Array(w1874, w1878) -> (w1876:dbl[])
            n835 = Initialize Array(w1884, w1878) -> (w1885:dbl[])
            n836 = Greater?(x=w1867, y=w1868) -> (0:w1869:bool)
            n837 = Bundle By Name("Y"=w1882, "dt"=w1877) -> (w1881:waveform(dbl))  [unwired: 1 in]
            n838 = Bundle By Name("Y"=w1876, "dt"=w1877) -> (w1875:waveform(dbl))  [unwired: 1 in]
            n839 = Bundle By Name("Y"=w1885, "dt"=w1877) -> (w1883:waveform(dbl))  [unwired: 1 in]
            n840 = Select(t=w1867, s=w1869, f=w1868) -> (s? t:f=w1866:dbl)
            n841 = Divide(x=w1866, y=w1871) -> (x/y=w1872:dbl)
            n842 = To Long Integer(number=w1872) -> (32bit integer=w1847:i32)
            n843 = for {
              N: w1847 -> [_]
              tunnel: w1871 -> [w1926]
              tunnel: w1861 -> [w1925]
              tunnel: w1877 -> [w1924]
              tunnel: w1878 -> [w1923]
              tunnel: [w1903] -> w1863
              tunnel: w1889 -> [w1901]
              tunnel: w1862 -> [w1902]
              tunnel: w1888 -> [w1919]
              tunnel: w1865 -> [w1918]
              tunnel: w1883 -> [w1915]
              tunnel: w1881 -> [w1907]
              tunnel: w1875 -> [w1914]
              shift-right: [w1922] -> w1886
              shift-left: w1887 -> [w1917]
              tunnel: w1873 -> [w1909]
              tunnel: w1870 -> [w1908]
              tunnel: [w1897] -> w1850
              tunnel: [w1895] -> w1851
              i -> [w1927]
              stop <- w1895 stop-if-true
              n844 = local write "Actual output Amplitude (V)"(w1902) -> ()
              n845 = call "Gen_Square_0to10V.vi"("sampling info"=w1908, "error in (no error)"=w1918, "Width (ms)"=w1901, "amplitude"=w1902, "frequency"=w1919) -> ("error out"=w1920:errorcluster, "signal out"=w1904:waveform(dbl))  [unwired: 5 in]
              n846 = Increment(x=w1927) -> (x+1=w1928:i32)
              n847 = property on="Actual Needle Output (V)" class="DigNum (strict)"("Blinking"=TRUE) -> ()  [unwired: 2 in, 2 out]
              n848 = local write "Output waveform"(w1904) -> ()
              n849 = Multiply(x=w1926, y=w1928) -> (x*y=w1911:dbl)
              n850 = Negate(x=w1911) -> (-x=w1912:dbl)
              n851 = Select(t=w1911, s=w1909, f=w1912) -> (s? t:f=w1910:dbl)
              n852 = Add(x=w1925, y=w1910) -> (x+y=w1906:dbl)
              n853 = Divide(x=w1906, y=1.0) -> (x/y=w1899:dbl)
              n854 = Less Than 0?(x=w1899) -> (x < 0?=w1900:bool)
              n855 = Select(t=0.0, s=w1900, f=w1899) -> (s? t:f=w1897:dbl)
              n856 = local write "Actual Needle Output (V)"(w1897) -> ()
              n857 = Initialize Array(w1897, w1923) -> (w1892:dbl[])
              n858 = In Range and Coerce(upper limit=10.0, x=w1892, lower limit=0.0) -> (coerced(x)=w1891:dbl[])  [unwired: 1 out]
              n859 = Bundle By Name("Y"=w1891, "dt"=w1924) -> (w1913:waveform(dbl))  [unwired: 1 in]
              n860 = Merge Signals(w1904, w1915, w1907, w1914, w1913) -> (w1921:dynamicdata)
              n861 = local read "Abort Change"() -> (w1896:bool)
              n862 = local read "stop"() -> (w1894:bool)
              n863 = call-poly <vilib>:"DAQmx Write.vi"("task/channels in"=w1917, "data"=w1921, "error in"=w1920) -> ("task out"=w1922:refnum<k21>, "error out"=w1903:errorcluster)  [unwired: 10 in, 1 out]
              n864 = Or(x=w1896, y=w1894) -> (x .or. y?=w1895:bool)
              n865 = case shown="True" w1895 {
                tunnel: w1897 -> [_ w1929]
                frame False {
                }
                frame True {
                  n866 = local write "Needle Voltage"(w1929) -> ()
                }
              }
            }
            n867 = Equal To 0?(x=w1847) -> (x = 0?=w1853:bool)
            n868 = Not(x=w1851) -> (.not. x?=w1854:bool)
            n869 = Merge Errors(w1863) -> (w1864:errorcluster)
            n870 = Or(x=w1854, y=w1853) -> (x .or. y?=w1852:bool)
            n871 = Select(t=w1848, s=w1852, f=w1850) -> (s? t:f=w1849:dbl)
          }
          event "stop": Value Change {
            w1943 = 0.0 ("Width (ms) : 3.5")
            w1946 = TRUE ("Blinking")
            n872 = event-data() -> ()  [unwired: 1 in, 1 out]
            n873 = property on="Actual Y Output (V)" class="DigNum (strict)"("Blinking"=w1946) -> ()  [unwired: 2 in, 2 out]
            n874 = property on="Actual Needle Output (V)" class="DigNum (strict)"("Blinking"=w1946) -> ()  [unwired: 2 in, 2 out]
            n875 = property on="Actual output Amplitude (V)" class="DigNum (strict)"("Blinking"=w1946) -> ()  [unwired: 2 in, 2 out]
            n876 = property on="Actual X Output (V)" class="DigNum (strict)"("Blinking"=w1946) -> ()  [unwired: 2 in, 2 out]
            n877 = property on="Actual Einzel Output (V)" class="DigNum (strict)"("Blinking"=w1946) -> ()  [unwired: 2 in, 2 out]
            n878 = Build Array(w1936, w1935) -> (w1934:dbl[])
            n879 = Equal To 0?(x=w1934) -> (x = 0?=w1933:bool[])
            n880 = Or Array Elements(Boolean array=w1933) -> (logical OR=w1932:bool)
            n881 = Not(x=w1932) -> (.not. x?=w1931:bool)
            n882 = Select(t=w1942, s=w1931, f=0.0) -> (s? t:f=w1938:dbl)
            n883 = Greater?(x=w1938, y=w1937) -> (0:w1956:bool)
            n884 = Select(t=w1938, s=w1956, f=w1937) -> (s? t:f=w1947:dbl)
            n885 = Greater?(x=w1941, y=w1947) -> (0:w1950:bool)
            n886 = Select(t=w1941, s=w1950, f=w1947) -> (s? t:f=w1944:dbl)
            n887 = Multiply(x=20.0, y=w1944) -> (x*y=w1940:dbl)
            n888 = Increment(x=w1940) -> (x+1=w1945:dbl)
            n889 = for {
              N: w1945 -> [w1966]
              tunnel: w1935 -> [w1980]
              tunnel: w1936 -> [w1979]
              tunnel: w1958 -> [w1973]
              tunnel: w1942 -> [w1981]
              tunnel: w1954 -> [w1970]
              tunnel: w1955 -> [w1969]
              tunnel: w1937 -> [w1971]
              tunnel: [w1969] -> _ mode=indexing
              shift-right: [w1975] -> w1949
              shift-left: w1957 -> [w1974]
              tunnel: w1941 -> [w1962]
              tunnel: w1952 -> [w1977]
              tunnel: [w1978] -> w1953
              i -> [w1968]
              n890 = Subtract(x=w1966, y=1) -> (x-y=w1965:i32)
              n891 = Wait (ms)(milliseconds to wait=u32 250) -> ()  [unwired: 1 out]
              n892 = Equal?(x=w1965, y=w1968) -> (x = y?=w1967:bool)
              n893 = case shown="False" w1967 {
                tunnel: w1981 -> [w2021 _]
                tunnel: w1980 -> [w2020 _]
                tunnel: w1979 -> [w2019 _]
                tunnel: [w2018 w2029] -> w1976
                tunnel: w1974 -> [w2017 w2029]
                tunnel: w1973 -> [w2013 _]
                tunnel: [w2012 w2030] -> w1972
                tunnel: w1971 -> [w2008 _]
                tunnel: w1966 -> [w2000 _]
                tunnel: w1970 -> [w1996 w2026]
                tunnel: w1969 -> [w1998 w2027]
                tunnel: w1968 -> [w1988 _]
                tunnel: w1962 -> [w1999 _]
                tunnel: [w1990 w2028] -> w1961
                frame False {
                  w1986 = T5 4 items=["Get", "Set X", "Set Y", "Set XY", "Internal"] ("Ring")
                  w1987 = 0.0 ("t")
                  w1995 = 1.0 ("y")
                  n894 = Divide(x=w2008, y=w2000) -> (x/y=w2010:dbl)
                  n895 = Divide(x=w1999, y=w2000) -> (x/y=w2002:dbl)
                  n896 = Divide(x=w2021, y=w2000) -> (x/y=w2016:dbl)
                  n897 = call "XYVoltageFGV.vi"("X Voltage"=w1987, "Y Voltage"=w1987, "Ring"=w1986) -> ("X Voltage 2"=w1984:dbl, "Y Voltage 2"=w1983:dbl)  [unwired: 5 in, 1 out]
                  n898 = Multiply(x=w2010, y=w1988) -> (x*y=w2009:dbl)
                  n899 = Multiply(x=w2002, y=w1988) -> (x*y=w2001:dbl)
                  n900 = Multiply(x=w2016, y=w1988) -> (x*y=w2015:dbl)
                  n901 = call "scale xy steering.vi"("-2.5 to 2.5 V input"=w1983) -> ("0 to 9 V output"=w1982:dbl)  [unwired: 1 in, 1 out]
                  n902 = call "scale xy steering.vi"("-2.5 to 2.5 V input"=w1984) -> ("0 to 9 V output"=w1985:dbl)  [unwired: 1 in, 1 out]
                  n903 = local write "Actual X Output (V)"(w1985) -> ()
                  n904 = local write "Actual Y Output (V)"(w1982) -> ()
                  n905 = Subtract(x=w2008, y=w2009) -> (x-y=w1991:dbl)
                  n906 = Subtract(x=w1999, y=w2001) -> (x-y=w1993:dbl)
                  n907 = Subtract(x=w2021, y=w2015) -> (x-y=w2014:dbl)
                  n908 = Initialize Array(w1985, w1996) -> (w2006:dbl[])
                  n909 = Initialize Array(w1982, w1996) -> (w2004:dbl[])
                  n910 = local write "Actual output Amplitude (V)"(w2014) -> ()
                  n911 = call "Gen_Square_0to10V.vi"("sampling info"=w2013, "error in (no error)"=w2017, "Width (ms)"=w2020, "amplitude"=w2014, "frequency"=w2019) -> ("error out"=w2018:errorcluster, "signal out"=w1990:waveform(dbl))  [unwired: 5 in]
                  n912 = Bundle By Name("Y"=w2006, "dt"=w1998) -> (w2005:waveform(dbl))  [unwired: 1 in]
                  n913 = Bundle By Name("Y"=w2004, "dt"=w1998) -> (w2003:waveform(dbl))  [unwired: 1 in]
                  n914 = Divide(x=w1991, y=w1995) -> (x/y=w1992:dbl)
                  n915 = Divide(x=w1993, y=w1995) -> (x/y=w1994:dbl)
                  n916 = local write "Actual Einzel Output (V)"(w1992) -> ()
                  n917 = local write "Actual Needle Output (V)"(w1994) -> ()
                  n918 = Initialize Array(w1992, w1996) -> (w2011:dbl[])
                  n919 = Initialize Array(w1994, w1996) -> (w1997:dbl[])
                  n920 = Bundle By Name("Y"=w2011, "dt"=w1998) -> (w2007:waveform(dbl))  [unwired: 1 in]
                  n921 = Bundle By Name("Y"=w1997, "dt"=w1998) -> (w1989:waveform(dbl))  [unwired: 1 in]
                  n922 = Merge Signals(w1990, w2007, w2005, w2003, w1989) -> (w2012:dynamicdata)
                }
                frame True {
                  w2023 = 0.0 ("element")
                  n923 = local write "Actual Needle Output (V)"(w2023) -> ()
                  n924 = local write "Needle Voltage"(w2023) -> ()
                  n925 = local write "Desired Amplitude (V)"(w2023) -> ()
                  n926 = local write "Einzel Voltage"(w2023) -> ()
                  n927 = local write "Actual output Amplitude (V)"(w2023) -> ()
                  n928 = local write "X Voltage"(w2023) -> ()
                  n929 = local write "Y Voltage"(w2023) -> ()
                  n930 = local write "Actual Einzel Output (V)"(w2023) -> ()
                  n931 = Initialize Array(w2023, w2026) -> (w2031:dbl[])
                  n932 = call "scale xy steering.vi"("-2.5 to 2.5 V input"=w2023) -> ("0 to 9 V output"=w2022:dbl)  [unwired: 1 in, 1 out]
                  n933 = local write "Actual X Output (V)"(w2022) -> ()
                  n934 = local write "Actual Y Output (V)"(w2022) -> ()
                  n935 = Bundle By Name("Y"=w2031, "dt"=w2027) -> (w2028:waveform(dbl))  [unwired: 1 in]
                  n936 = Initialize Array(w2022, w2026) -> (w2025:dbl[])
                  n937 = Bundle By Name("Y"=w2025, "dt"=w2027) -> (w2024:waveform(dbl))  [unwired: 1 in]
                  n938 = Merge Signals(w2028, w2028, w2024, w2024, w2028) -> (w2030:dynamicdata)
                }
              }
              n939 = local write "Output waveform"(w1961) -> ()
              n940 = call-poly <vilib>:"DAQmx Write.vi"("task/channels in"=w1977, "data"=w1972, "error in"=w1976) -> ("task out"=w1978:refnum<k21>, "error out"=w1975:errorcluster)  [unwired: 10 in, 1 out]
            }
            n941 = flat-sequence {
              tunnel: w1949 -> [w1960]
              tunnel: [w1960] -> w1948
              frame #0 {
                w1959 = TRUE ("Finished")
                n942 = local write "stop"(w1959) -> ()
                "Finished" <- w1959
              }
            }
          }
          event "Desired Amplitude (V)": Value Change {
            w2060 = 0.05 ("y")
            n943 = event-data() -> ("NewVal"=w2039:dbl)  [unwired: 1 in, 1 out]
            n944 = local write "Actual X Output (V)"(w2073) -> ()
            n945 = local write "Actual Needle Output (V)"(w2063) -> ()
            n946 = local write "Actual Einzel Output (V)"(w2076) -> ()
            n947 = Greater?(x=w2039, y=w2052) -> (0:w2062:bool)
            n948 = Subtract(x=w2039, y=w2052) -> (x-y=w2058:dbl)
            n949 = Subtract(x=w2052, y=w2039) -> (x-y=w2056:dbl)
            n950 = Initialize Array(w2073, w2067) -> (w2074:dbl[])
            n951 = Initialize Array(w2071, w2067) -> (w2070:dbl[])
            n952 = Initialize Array(w2063, w2067) -> (w2065:dbl[])
            n953 = Initialize Array(w2076, w2067) -> (w2078:dbl[])
            n954 = Greater?(x=w2058, y=w2056) -> (0:w2059:bool)
            n955 = Bundle By Name("Y"=w2074, "dt"=w2066) -> (w2072:waveform(dbl))  [unwired: 1 in]
            n956 = Bundle By Name("Y"=w2070, "dt"=w2066) -> (w2069:waveform(dbl))  [unwired: 1 in]
            n957 = Bundle By Name("Y"=w2065, "dt"=w2066) -> (w2064:waveform(dbl))  [unwired: 1 in]
            n958 = Bundle By Name("Y"=w2078, "dt"=w2066) -> (w2077:waveform(dbl))  [unwired: 1 in]
            n959 = Select(t=w2058, s=w2059, f=w2056) -> (s? t:f=w2057:dbl)
            n960 = Quotient & Remainder(x=w2057, y=w2060) -> (floor(x/y)=w2061:dbl)  [unwired: 1 out]
            n961 = Build Array(w2037, w2035) -> (w2034:dbl[])
            n962 = Equal To 0?(x=w2034) -> (x = 0?=w2033:bool[])
            n963 = To Long Integer(number=w2061) -> (32bit integer=w2038:i32)
            n964 = Or Array Elements(Boolean array=w2033) -> (logical OR=w2032:bool)
            n965 = case shown="True" w2032 {
              tunnel: w2037 -> [w2099 w2117]
              tunnel: w2035 -> [w2098 w2116]
              tunnel: w2080 -> [w2097 w2115]
              tunnel: w2079 -> [w2096 w2114]
              tunnel: w2077 -> [w2095 w2113]
              tunnel: [w2094 w2112] -> w2075
              tunnel: w2072 -> [w2093 w2111]
              tunnel: w2069 -> [w2092 w2110]
              tunnel: w2064 -> [w2091 w2109]
              tunnel: w2062 -> [_ w2108]
              tunnel: w2060 -> [_ w2107]
              tunnel: w2055 -> [w2090 w2106]
              tunnel: [w2089 w2105] -> w2054
              tunnel: w2052 -> [_ w2104]
              tunnel: [w2088 w2103] -> w2042
              tunnel: [w2081 w2102] -> w2041
              tunnel: w2038 -> [_ w2101]
              tunnel: w2036 -> [w2081 _]
              frame True {
                n966 = property on="Actual output Amplitude (V)" class="DigNum (strict)"("Blinking"=TRUE) -> ()  [unwired: 2 in, 2 out]
                n967 = local write "Actual output Amplitude (V)"(w2081) -> ()
                n968 = call "Gen_Square_0to10V.vi"("sampling info"=w2096, "error in (no error)"=w2090, "Width (ms)"=w2099, "amplitude"=w2081, "frequency"=w2098) -> ("error out"=w2087:errorcluster, "signal out"=w2084:waveform(dbl))  [unwired: 5 in]
                n969 = local write "Output waveform"(w2084) -> ()
                n970 = Merge Signals(w2084, w2095, w2093, w2092, w2091) -> (w2085:dynamicdata)
                n971 = call-poly <vilib>:"DAQmx Write.vi"("task/channels in"=w2097, "data"=w2085, "error in"=w2087) -> ("task out"=w2094:refnum<k21>, "error out"=w2089:errorcluster)  [unwired: 10 in, 1 out]
                n972 = local read "Abort Change"() -> (w2083:bool)
                n973 = local read "stop"() -> (w2082:bool)
                n974 = Or(x=w2083, y=w2082) -> (x .or. y?=w2088:bool)
                n975 = case shown="True" w2088 {
                  tunnel: w2081 -> [_ w2100]
                  frame False {
                  }
                  frame True {
                    n976 = local write "Desired Amplitude (V)"(w2100) -> ()
                  }
                }
              }
              frame False {
                n977 = for {
                  N: w2101 -> [_]
                  tunnel: w2117 -> [w2143]
                  tunnel: w2116 -> [w2142]
                  tunnel: w2104 -> [w2140]
                  tunnel: w2106 -> [w2139]
                  tunnel: [w2137] -> w2105
                  tunnel: w2114 -> [w2135]
                  tunnel: w2107 -> [w2132]
                  tunnel: w2113 -> [w2130]
                  tunnel: w2111 -> [w2128]
                  tunnel: w2110 -> [w2129]
                  tunnel: w2109 -> [w2127]
                  shift-right: [w2136] -> w2112
                  shift-left: w2115 -> [w2138]
                  tunnel: w2108 -> [w2123]
                  tunnel: [w2121] -> w2102
                  tunnel: [w2119] -> w2103
                  i -> [w2141]
                  stop <- w2119 stop-if-true
                  n978 = Increment(x=w2141) -> (x+1=w2134:i32)
                  n979 = property on="Actual output Amplitude (V)" class="DigNum (strict)"("Blinking"=TRUE) -> ()  [unwired: 2 in, 2 out]
                  n980 = Multiply(x=w2132, y=w2134) -> (x*y=w2124:dbl)
                  n981 = Negate(x=w2124) -> (-x=w2126:dbl)
                  n982 = Select(t=w2124, s=w2123, f=w2126) -> (s? t:f=w2125:dbl)
                  n983 = Add(x=w2140, y=w2125) -> (x+y=w2121:dbl)
                  n984 = local write "Actual output Amplitude (V)"(w2121) -> ()
                  n985 = call "Gen_Square_0to10V.vi"("sampling info"=w2135, "error in (no error)"=w2139, "Width (ms)"=w2143, "amplitude"=w2121, "frequency"=w2142) -> ("error out"=w2144:errorcluster, "signal out"=w2122:waveform(dbl))  [unwired: 5 in]
                  n986 = local write "Output waveform"(w2122) -> ()
                  n987 = Merge Signals(w2122, w2130, w2128, w2129, w2127) -> (w2131:dynamicdata)
                  n988 = call-poly <vilib>:"DAQmx Write.vi"("task/channels in"=w2138, "data"=w2131, "error in"=w2144) -> ("task out"=w2136:refnum<k21>, "error out"=w2137:errorcluster)  [unwired: 10 in, 1 out]
                  n989 = local read "Abort Change"() -> (w2120:bool)
                  n990 = local read "stop"() -> (w2118:bool)
                  n991 = Or(x=w2120, y=w2118) -> (x .or. y?=w2119:bool)
                  n992 = case shown="True" w2119 {
                    tunnel: w2121 -> [_ w2145]
                    frame False {
                    }
                    frame True {
                      n993 = local write "Desired Amplitude (V)"(w2145) -> ()
                    }
                  }
                }
              }
            }
            n994 = Equal To 0?(x=w2038) -> (x = 0?=w2044:bool)
            n995 = Not(x=w2042) -> (.not. x?=w2045:bool)
            n996 = Merge Errors(w2054) -> (w2053:errorcluster)
            n997 = Or(x=w2045, y=w2044) -> (x .or. y?=w2043:bool)
            n998 = Select(t=w2039, s=w2043, f=w2041) -> (s? t:f=w2040:dbl)
          }
          event "Frequency": Value Change {
            w2173 = 0.5 ("y")
            n999 = event-data() -> ("NewVal"=w2153:dbl)  [unwired: 1 in, 1 out]
            n1000 = local write "Actual X Output (V)"(w2186) -> ()
            n1001 = local write "Actual Needle Output (V)"(w2176) -> ()
            n1002 = local write "Actual Einzel Output (V)"(w2189) -> ()
            n1003 = Greater?(x=w2153, y=w2165) -> (0:w2175:bool)
            n1004 = Subtract(x=w2153, y=w2165) -> (x-y=w2171:dbl)
            n1005 = Subtract(x=w2165, y=w2153) -> (x-y=w2169:dbl)
            n1006 = Initialize Array(w2186, w2180) -> (w2187:dbl[])
            n1007 = Initialize Array(w2184, w2180) -> (w2183:dbl[])
            n1008 = Initialize Array(w2176, w2180) -> (w2178:dbl[])
            n1009 = Initialize Array(w2189, w2180) -> (w2191:dbl[])
            n1010 = Greater?(x=w2171, y=w2169) -> (0:w2172:bool)
            n1011 = Bundle By Name("Y"=w2187, "dt"=w2179) -> (w2185:waveform(dbl))  [unwired: 1 in]
            n1012 = Bundle By Name("Y"=w2183, "dt"=w2179) -> (w2182:waveform(dbl))  [unwired: 1 in]
            n1013 = Bundle By Name("Y"=w2178, "dt"=w2179) -> (w2177:waveform(dbl))  [unwired: 1 in]
            n1014 = Bundle By Name("Y"=w2191, "dt"=w2179) -> (w2190:waveform(dbl))  [unwired: 1 in]
            n1015 = Select(t=w2171, s=w2172, f=w2169) -> (s? t:f=w2170:dbl)
            n1016 = Build Array(w2149, w2150) -> (w2148:dbl[])
            n1017 = Quotient & Remainder(x=w2170, y=w2173) -> (floor(x/y)=w2174:dbl)  [unwired: 1 out]
            n1018 = Equal To 0?(x=w2148) -> (x = 0?=w2147:bool[])
            n1019 = Or Array Elements(Boolean array=w2147) -> (logical OR=w2146:bool)
            n1020 = To Long Integer(number=w2174) -> (32bit integer=w2152:i32)
            n1021 = case shown="False" w2146 {
              tunnel: w2149 -> [w2213 w2232]
              tunnel: w2194 -> [w2195 w2231]
              tunnel: w2193 -> [w2212 w2230]
              tunnel: w2192 -> [w2211 w2229]
              tunnel: w2190 -> [w2210 w2228]
              tunnel: [w2209 w2227] -> w2188
              tunnel: w2185 -> [w2208 w2226]
              tunnel: w2182 -> [w2207 w2225]
              tunnel: w2177 -> [w2206 w2224]
              tunnel: w2175 -> [_ w2223]
              tunnel: w2173 -> [_ w2222]
              tunnel: w2168 -> [w2205 w2221]
              tunnel: [w2204 w2220] -> w2167
              tunnel: w2150 -> [w2203 w2219]
              tunnel: w2165 -> [_ w2218]
              tunnel: [w2202 w2217] -> w2155
              tunnel: [w2195 w2216] -> w2154
              tunnel: w2152 -> [_ w2215]
              frame True {
                n1022 = property on="Actual output Frequency" class="DigNum (strict)"("Blinking"=TRUE) -> ()  [unwired: 2 in, 2 out]
                n1023 = call "Gen_Square_0to10V.vi"("sampling info"=w2211, "error in (no error)"=w2205, "Width (ms)"=w2213, "amplitude"=w2203, "frequency"=w2195) -> ("error out"=w2201:errorcluster, "signal out"=w2199:waveform(dbl))  [unwired: 5 in]
                n1024 = local write "Actual output Frequency"(w2195) -> ()
                n1025 = local write "Output waveform"(w2199) -> ()
                n1026 = Merge Signals(w2199, w2210, w2208, w2207, w2206) -> (w2200:dynamicdata)
                n1027 = local read "Abort Change"() -> (w2197:bool)
                n1028 = call-poly <vilib>:"DAQmx Write.vi"("task/channels in"=w2212, "data"=w2200, "error in"=w2201) -> ("task out"=w2209:refnum<k21>, "error out"=w2204:errorcluster)  [unwired: 10 in, 1 out]
                n1029 = local read "stop"() -> (w2196:bool)
                n1030 = Or(x=w2197, y=w2196) -> (x .or. y?=w2202:bool)
                n1031 = case shown="True" w2202 {
                  tunnel: w2195 -> [_ w2214]
                  frame False {
                  }
                  frame True {
                    n1032 = local write "Frequency"(w2214) -> ()
                  }
                }
              }
              frame False {
                n1033 = for {
                  N: w2215 -> [_]
                  tunnel: w2232 -> [w2258]
                  tunnel: w2231 -> [_]
                  tunnel: w2218 -> [w2256]
                  tunnel: w2221 -> [w2255]
                  tunnel: [w2253] -> w2220
                  tunnel: w2229 -> [w2251]
                  tunnel: w2222 -> [w2249]
                  tunnel: w2228 -> [w2247]
                  tunnel: w2226 -> [w2245]
                  tunnel: w2225 -> [w2246]
                  tunnel: w2224 -> [w2244]
                  shift-right: [w2252] -> w2227
                  shift-left: w2230 -> [w2254]
                  tunnel: w2223 -> [w2240]
                  tunnel: w2219 -> [w2237]
                  tunnel: [w2236] -> w2216
                  tunnel: [w2234] -> w2217
                  i -> [w2257]
                  stop <- w2234 stop-if-true
                  n1034 = Increment(x=w2257) -> (x+1=w2250:i32)
                  n1035 = Multiply(x=w2249, y=w2250) -> (x*y=w2241:dbl)
                  n1036 = property on="Actual output Frequency" class="DigNum (strict)"("Blinking"=TRUE) -> ()  [unwired: 2 in, 2 out]
                  n1037 = Negate(x=w2241) -> (-x=w2243:dbl)
                  n1038 = Select(t=w2241, s=w2240, f=w2243) -> (s? t:f=w2242:dbl)
                  n1039 = Add(x=w2256, y=w2242) -> (x+y=w2236:dbl)
                  n1040 = call "Gen_Square_0to10V.vi"("sampling info"=w2251, "error in (no error)"=w2255, "Width (ms)"=w2258, "amplitude"=w2237, "frequency"=w2236) -> ("error out"=w2259:errorcluster, "signal out"=w2239:waveform(dbl))  [unwired: 5 in]
                  n1041 = local write "Actual output Frequency"(w2236) -> ()
                  n1042 = local write "Output waveform"(w2239) -> ()
                  n1043 = Merge Signals(w2239, w2247, w2245, w2246, w2244) -> (w2248:dynamicdata)
                  n1044 = local read "Abort Change"() -> (w2235:bool)
                  n1045 = call-poly <vilib>:"DAQmx Write.vi"("task/channels in"=w2254, "data"=w2248, "error in"=w2259) -> ("task out"=w2252:refnum<k21>, "error out"=w2253:errorcluster)  [unwired: 10 in, 1 out]
                  n1046 = local read "stop"() -> (w2233:bool)
                  n1047 = Or(x=w2235, y=w2233) -> (x .or. y?=w2234:bool)
                  n1048 = case shown="True" w2234 {
                    tunnel: w2236 -> [_ w2260]
                    frame False {
                    }
                    frame True {
                      n1049 = local write "Frequency"(w2260) -> ()
                    }
                  }
                }
              }
            }
            n1050 = Equal To 0?(x=w2152) -> (x = 0?=w2157:bool)
            n1051 = Not(x=w2155) -> (.not. x?=w2158:bool)
            n1052 = Merge Errors(w2167) -> (w2166:errorcluster)
            n1053 = Or(x=w2158, y=w2157) -> (x .or. y?=w2156:bool)
            n1054 = Select(t=w2153, s=w2156, f=w2154) -> (s? t:f=w2151:dbl)
          }
          event "Width (ms) : 0.1": Value Change {
            w2288 = 0.1 ("y")
            n1055 = event-data() -> ("NewVal"=w2266:dbl)  [unwired: 1 in, 1 out]
            n1056 = local write "Actual X Output (V)"(w2301) -> ()
            n1057 = local write "Actual Needle Output (V)"(w2291) -> ()
            n1058 = local write "Actual Einzel Output (V)"(w2304) -> ()
            n1059 = Greater?(x=w2266, y=w2280) -> (0:w2290:bool)
            n1060 = Subtract(x=w2266, y=w2280) -> (x-y=w2286:dbl)
            n1061 = Subtract(x=w2280, y=w2266) -> (x-y=w2284:dbl)
            n1062 = Initialize Array(w2301, w2295) -> (w2302:dbl[])
            n1063 = Initialize Array(w2299, w2295) -> (w2298:dbl[])
            n1064 = Initialize Array(w2291, w2295) -> (w2293:dbl[])
            n1065 = Initialize Array(w2304, w2295) -> (w2306:dbl[])
            n1066 = Greater?(x=w2286, y=w2284) -> (0:w2287:bool)
            n1067 = Bundle By Name("Y"=w2302, "dt"=w2294) -> (w2300:waveform(dbl))  [unwired: 1 in]
            n1068 = Bundle By Name("Y"=w2298, "dt"=w2294) -> (w2297:waveform(dbl))  [unwired: 1 in]
            n1069 = Bundle By Name("Y"=w2293, "dt"=w2294) -> (w2292:waveform(dbl))  [unwired: 1 in]
            n1070 = Bundle By Name("Y"=w2306, "dt"=w2294) -> (w2305:waveform(dbl))  [unwired: 1 in]
            n1071 = Select(t=w2286, s=w2287, f=w2284) -> (s? t:f=w2285:dbl)
            n1072 = Build Array(w2265, w2264) -> (w2263:dbl[])
            n1073 = Quotient & Remainder(x=w2285, y=w2288) -> (floor(x/y)=w2289:dbl)  [unwired: 1 out]
            n1074 = Equal To 0?(x=w2263) -> (x = 0?=w2262:bool[])
            n1075 = Or Array Elements(Boolean array=w2262) -> (logical OR=w2261:bool)
            n1076 = To Long Integer(number=w2289) -> (32bit integer=w2270:i32)
            n1077 = case shown="True" w2261 {
              tunnel: w2309 -> [w2310 w2347]
              tunnel: w2265 -> [w2328 w2346]
              tunnel: w2308 -> [w2327 w2345]
              tunnel: w2307 -> [w2326 w2344]
              tunnel: w2305 -> [w2325 w2343]
              tunnel: [w2324 w2342] -> w2303
              tunnel: w2300 -> [w2323 w2341]
              tunnel: w2297 -> [w2322 w2340]
              tunnel: w2292 -> [w2321 w2339]
              tunnel: w2290 -> [_ w2338]
              tunnel: w2288 -> [_ w2337]
              tunnel: w2283 -> [w2320 w2336]
              tunnel: [w2319 w2335] -> w2282
              tunnel: w2264 -> [w2318 w2334]
              tunnel: w2280 -> [_ w2333]
              tunnel: [w2317 w2332] -> w2273
              tunnel: w2270 -> [_ w2331]
              tunnel: [w2310 w2330] -> w2267
              frame True {
                n1078 = property on="Actual output width (ms)" class="DigNum (strict)"("Blinking"=TRUE) -> ()  [unwired: 2 in, 2 out]
                n1079 = call "Gen_Square_0to10V.vi"("sampling info"=w2326, "error in (no error)"=w2320, "Width (ms)"=w2310, "amplitude"=w2318, "frequency"=w2328) -> ("error out"=w2316:errorcluster, "signal out"=w2314:waveform(dbl))  [unwired: 5 in]
                n1080 = local write "Actual output width (ms)"(w2310) -> ()
                n1081 = local write "Output waveform"(w2314) -> ()
                n1082 = Merge Signals(w2314, w2325, w2323, w2322, w2321) -> (w2315:dynamicdata)
                n1083 = local read "Abort Change"() -> (w2312:bool)
                n1084 = call-poly <vilib>:"DAQmx Write.vi"("task/channels in"=w2327, "data"=w2315, "error in"=w2316) -> ("task out"=w2324:refnum<k21>, "error out"=w2319:errorcluster)  [unwired: 10 in, 1 out]
                n1085 = local read "stop"() -> (w2311:bool)
                n1086 = Or(x=w2311, y=w2312) -> (x .or. y?=w2317:bool)
                n1087 = case shown="True" w2317 {
                  tunnel: w2310 -> [_ w2329]
                  frame False {
                  }
                  frame True {
                    n1088 = local write "Width (ms) : 0.1"(w2329) -> ()
                  }
                }
              }
              frame False {
                n1089 = for {
                  N: w2331 -> [_]
                  tunnel: w2347 -> [_]
                  tunnel: w2346 -> [w2373]
                  tunnel: w2333 -> [w2371]
                  tunnel: w2336 -> [w2370]
                  tunnel: [w2368] -> w2335
                  tunnel: w2344 -> [w2366]
                  tunnel: w2337 -> [w2364]
                  tunnel: w2343 -> [w2362]
                  tunnel: w2341 -> [w2360]
                  tunnel: w2340 -> [w2361]
                  tunnel: w2339 -> [w2359]
                  shift-right: [w2367] -> w2342
                  shift-left: w2345 -> [w2369]
                  tunnel: w2338 -> [w2355]
                  tunnel: w2334 -> [w2353]
                  tunnel: [w2351] -> w2330
                  tunnel: [w2349] -> w2332
                  i -> [w2372]
                  stop <- w2349 stop-if-true
                  n1090 = Increment(x=w2372) -> (x+1=w2365:i32)
                  n1091 = Multiply(x=w2364, y=w2365) -> (x*y=w2356:dbl)
                  n1092 = property on="Actual output width (ms)" class="DigNum (strict)"("Blinking"=TRUE) -> ()  [unwired: 2 in, 2 out]
                  n1093 = Negate(x=w2356) -> (-x=w2358:dbl)
                  n1094 = Select(t=w2356, s=w2355, f=w2358) -> (s? t:f=w2357:dbl)
                  n1095 = Add(x=w2371, y=w2357) -> (x+y=w2351:dbl)
                  n1096 = call "Gen_Square_0to10V.vi"("sampling info"=w2366, "error in (no error)"=w2370, "Width (ms)"=w2351, "amplitude"=w2353, "frequency"=w2373) -> ("error out"=w2374:errorcluster, "signal out"=w2354:waveform(dbl))  [unwired: 5 in]
                  n1097 = local write "Actual output width (ms)"(w2351) -> ()
                  n1098 = local write "Output waveform"(w2354) -> ()
                  n1099 = Merge Signals(w2354, w2362, w2360, w2361, w2359) -> (w2363:dynamicdata)
                  n1100 = local read "Abort Change"() -> (w2350:bool)
                  n1101 = call-poly <vilib>:"DAQmx Write.vi"("task/channels in"=w2369, "data"=w2363, "error in"=w2374) -> ("task out"=w2367:refnum<k21>, "error out"=w2368:errorcluster)  [unwired: 10 in, 1 out]
                  n1102 = local read "stop"() -> (w2348:bool)
                  n1103 = Or(x=w2348, y=w2350) -> (x .or. y?=w2349:bool)
                  n1104 = case shown="True" w2349 {
                    tunnel: w2351 -> [_ w2375]
                    frame False {
                    }
                    frame True {
                      n1105 = local write "Width (ms) : 0.1"(w2375) -> ()
                    }
                  }
                }
              }
            }
            n1106 = Equal To 0?(x=w2270) -> (x = 0?=w2271:bool)
            n1107 = Not(x=w2273) -> (.not. x?=w2272:bool)
            n1108 = Or(x=w2272, y=w2271) -> (x .or. y?=w2269:bool)
            n1109 = Merge Errors(w2282) -> (w2281:errorcluster)
            n1110 = Select(t=w2266, s=w2269, f=w2267) -> (s? t:f=w2268:dbl)
          }
        }
        n1111 = call-poly <userlib>:"Data Changed__ogtk.vi"("Boolean"=w1270) -> ("Changed"=w1271:bool)
        n1112 = And(x=w1293, y=w1270) -> (x .and. y?=w1292:bool)
        n1113 = Or(x=w1292, y=w1271) -> (x .or. y?=w1294:bool)
        n1114 = case shown="True" w1294 {
          tunnel: w1270 -> [_ w1341]
          tunnel: w1296 -> [w1338 w1346]
          tunnel: [w1338 w1345] -> w1295
          tunnel: w1292 -> [_ w1340]
          tunnel: w1269 -> [w1337 w1344]
          tunnel: [w1337 w1343] -> w1268
          frame False {
          }
          frame True {
            n1115 = Select(t=FALSE, s=w1340, f=w1341) -> (s? t:f=w1342:bool)
            n1116 = case shown="True" w1342 {
              tunnel: w1346 -> [w1368 w1409]
              tunnel: [w1365 w1409] -> w1345
              tunnel: w1344 -> [w1347 _]
              tunnel: [w1347 w1407] -> w1343
              frame False {
                n1117 = Get Date/Time In Seconds() -> (seconds since 1Jan1904=w1371:timestamp)
                n1118 = call "timestamp_conversion.vi"("error in (no error)"=w1368, "Time Stamp"=w1371) -> ("error out"=w1369:errorcluster, "Integer Time"=w1348:i64)  [unwired: 7 in]
                n1119 = call "connect in.vi"("error in (no error)"=w1369) -> ("error out"=w1363:errorcluster, "Database Connection"=w1364:T8)  [unwired: 6 in, 1 out]
                n1120 = call-poly <vilib>:"DB Tools Execute Query.vi"("error in (no error)"=w1363, "SQL query"="SELECT id_experiment_settings\nFROM experiment_settings\nORDER BY integer_timestamp DESC\nLIMIT 1; ", "connection reference"=w1364) -> ("error out"=w1361:errorcluster, "recordset reference"=w1362:T9)  [unwired: 5 in]
                n1121 = call-poly <vilib>:"DB Tools Fetch Recordset Data.vi"("error in (no error)"=w1361, "recordset reference"=w1362) -> ("error out"=w1350:errorcluster, "recordset data"=w1356:variant[][], "recordset reference out"=w1360:T9)  [unwired: 3 in]
                n1122 = Index Array(array=w1356, index (row)=0, index (col)=0 ("disabled index (col)")) -> (element=w1353:variant)
                n1123 = xnode "Database Variant To Data"("database variant"=w1353, "error in (no error)"=w1350, "type"=0) -> ("data"=w1351:i32, "error out"=w1349:errorcluster)
                n1124 = Bundle("Integer Time"=w1347, "Integer Time"=w1348, "data"=w1351) -> (w1370:T14)  [unwired: 1 in]
                n1125 = call-poly <vilib>:"DB Tools Free Object.vi"("error in (no error)"=w1349, "recordset reference"=w1360) -> ("error out"=w1358:errorcluster, "connection reference"=w1359:T8)  [unwired: 8 in]
                n1126 = call <vilib>:"DB Tools Insert Data.vi"("create table? (F)"=FALSE, "data"=w1370, "error in (no error)"=w1358, "table"="run_times", "connection reference"=w1359) -> ("error out"=w1366:errorcluster, "connection reference out"=w1373:T8)  [unwired: 5 in]
                n1127 = call "connect out.vi"("error in (no error)"=w1363, "connection reference"=w1373) -> ("error out"=w1367:errorcluster)  [unwired: 9 in]
                n1128 = Merge Errors(w1366, w1367) -> (w1365:errorcluster)
              }
              frame True {
                n1129 = Get Date/Time In Seconds() -> (seconds since 1Jan1904=w1408:timestamp)
                n1130 = call "timestamp_conversion.vi"("Time Stamp"=w1408) -> ("Integer Time"=w1407:i64)  [unwired: 8 in, 1 out]
              }
            }
          }
        }
        n1131 = Unbundle By Name(w1295) -> ("status"=w1264:bool)
        n1132 = local read "Testing"() -> (w1265:bool)
        n1133 = call <vilib>:"Simple Error Handler.vi"("type of dialog (OK msg:1)"=w1323, "error in (no error)"=w1295) -> ("error?"=w1267:bool, "error out"=w1324:errorcluster)  [unwired: 3 in, 3 out]
        n1134 = Not(x=w1265) -> (.not. x?=w1262:bool)
        n1135 = And(x=w1262, y=w1267) -> (x .and. y?=→"error?":bool)
        n1136 = And(x=w1264, y=w1262) -> (x .and. y?=w1263:bool)
        n1137 = Or(x=w1263, y=w1293) -> (x .or. y?=w1325:bool)
        "Execution Number:" <- w1332
      }
      n1138 = call <vilib>:"DAQmx Clear Task.vi"("task in"=w62, "error in"=w77) -> ("error out"=w76:errorcluster)  [unwired: 13 in]
      n1139 = call <vilib>:"DAQmx Stop Task.vi"("task/channels in"=w113, "error in"=w112) -> ("task out"=w105:refnum<k21>, "error out"=w104:errorcluster)  [unwired: 12 in]
      n1140 = call <vilib>:"DAQmx Stop Task.vi"("task/channels in"=w111, "error in"=w110) -> ("task out"=w103:refnum<k21>, "error out"=w102:errorcluster)  [unwired: 12 in]
      n1141 = call <vilib>:"DAQmx Stop Task.vi"("task/channels in"=w107, "error in"=w106) -> ("task out"=w99:refnum<k21>, "error out"=w98:errorcluster)  [unwired: 12 in]
      n1142 = call <vilib>:"DAQmx Stop Task.vi"("task/channels in"=w109, "error in"=w108) -> ("task out"=w101:refnum<k21>, "error out"=w100:errorcluster)  [unwired: 12 in]
      n1143 = call <vilib>:"DAQmx Clear Task.vi"("task in"=w105, "error in"=w104) -> ("error out"=w87:errorcluster)  [unwired: 13 in]
      n1144 = call <vilib>:"DAQmx Clear Task.vi"("task in"=w103, "error in"=w102) -> ("error out"=w86:errorcluster)  [unwired: 13 in]
      n1145 = call <vilib>:"DAQmx Clear Task.vi"("task in"=w99, "error in"=w98) -> ("error out"=w84:errorcluster)  [unwired: 13 in]
      n1146 = call <vilib>:"DAQmx Clear Task.vi"("task in"=w101, "error in"=w100) -> ("error out"=w85:errorcluster)  [unwired: 13 in]
      n1147 = Merge Errors(w87, w86, w85, w84, w88) -> (w82:errorcluster)
      n1148 = call <vilib>:"DAQmx Clear Task.vi"("task in"=w132, "error in"=w128) -> ("error out"=w131:errorcluster)  [unwired: 13 in]
      n1149 = call <vilib>:"Simple Error Handler.vi"("type of dialog (OK msg:1)"=w147, "error in (no error)"=w131) -> ("error out"=w130:errorcluster)  [unwired: 3 in, 4 out]
      n1150 = Merge Errors(w130, w82, w76, w83) -> (w43:errorcluster)
    }
    frame Error {
    }
  }
  "error out" <- w42
